vi "MotorSPS.vi"() -> ()   [LabVIEW 2010]
uses:
  StepMotor.lvclass
  Archive.lvclass
  <vilib>/Utility/miscctls.llb/LVScalePositionTypeDef.ctl
  <vilib>/Utility/xml.llb/Write to XML File(string).vi
  <vilib>/Utility/xml.llb/Read From XML File(string).vi
  Параметры СПШ.vi
  <vilib>/Utility/miscctls.llb/LVRowAndColumnTypeDef.ctl
panel:
  in  "Reload":bool
  out "Разрешение энкодера":dbl format="%#_10g"
  in  "Макс скорость двигателя":dbl caption="max скорость двигателя"
  in  "Редукция":dbl
  in  "Останов":bool
  out "Archive Data":refnum<class "Archive.lvclass">
  out "Archive Event":refnum<class "Archive.lvclass">
  out "Статус связи с СПШ":bool
  in  "Скорость передачи":i32(ring)=16 items=["75", "110", "134", "150", "300", "600", "1200", "1800", "2400", "4800", "7200", "9600", "14400", "19200", "38400", "57600", "115200", "128000"]
  in  "Имя порта":refnum<visa-resource-name>="COM6"
  out "Индикатор Статуса Конт":bool
  in  "Статус контроллера СПШ":T1(ring)
  out "StepMotor":refnum<class "StepMotor.lvclass">
  in  "Выход из программы":bool
  in  "Tab Control":T2(tab)
  out "Начальная позиция":dbl
  in  "Контроль концевиков":bool=TRUE
  out "Текущая позиция":dbl
  out "Условие энкодер":bool
  out "Инкремент импульсов":dbl
  in  "Контроль энкодера":bool
  out "Условие время":bool
  out "Лимит времени":dbl format="%<%M:%S>T"
  in  "Контроль времени":bool
  in  "Способ управления СПШ":T3(radio) caption="Способ управления двигателем"
  out "СкорРучРежРед":dbl caption="Скорость вала редуктора" format="%#_g об/мин"
  in  "Расчитать скорость":bool
  in  "Поворт экрана":dbl=180.0 min=0.0 max=360.0 step=1.0 format="%#_g °"
  in  "Время в мин":dbl=18.0 min=1.0 max=60.0 step=1.0 format="%2d мин"
  out "СкорРучРежМот":dbl caption="Скорость вала мотора" format="%#_g об/мин"
  in  "Напраление вращения":enum32{"Лево", "Право"}(radio)
  in  "Стоп Руч":bool
  in  "Пуск Руч":bool caption="Пуск ручной"
  out "ИсхСостСтарСтоп":bool
  in  "Двигатель в исходное сотояние":bool
  in  "Скорость двигателя":dbl caption="Скорость двигателя  об/мин" min=0.0 max=720.0 step=5.0
  out "Скорость редуктора":dbl caption="Скорость редуктора об/мин"
  in  "КонтрольКон":T4(radio)=enum."КонтрольПравКон" caption="Контроль концевика"
  out "РучнойСтартСтоп":bool
  out "Журнал событий":i32(listbox)
  in  "Количество циклов":i32
  out "ЦиклСтартСтоп":bool
  in  "Остоновить цикл":bool
  in  "Запустить цикл":bool
  in  "Шаги одного цикла":string[][](table)=[["7", "37"], ["4", "37"], ["4", "37"], ["9", "37"]]
  in  "Режим работы двигателя":T5(radio)=enum."Цикл реверсирования 180°"
  out "Прав.Конц":bool
  out "Лев.Конц":bool
  out "GaugeAngle":cluster{dbl, dbl}(knob) caption="Gauge" scale=0.0..360.0
  out "Значение энкодера":dbl caption="Лимит импульсов энкодера"
  out "Выбег":dbl
  out "Заданная позиция":dbl
  in  "SpeedSlide":dbl(slide) step=5.0 scale=0.0..720.0
  in  "Tree":string(tree)
  out "Waveform Chart":dynamicdata(graph)
  out "error":errorcluster
  in  "Период регистрации":string(combo)="1" caption="Период регистрации файла"
  in  "Номер банка программ":u16(ring) items=["0", "1", "2", "3", "4", "5", "6", "7"]
  in  "OK Button":bool
  # "Параметры установки"
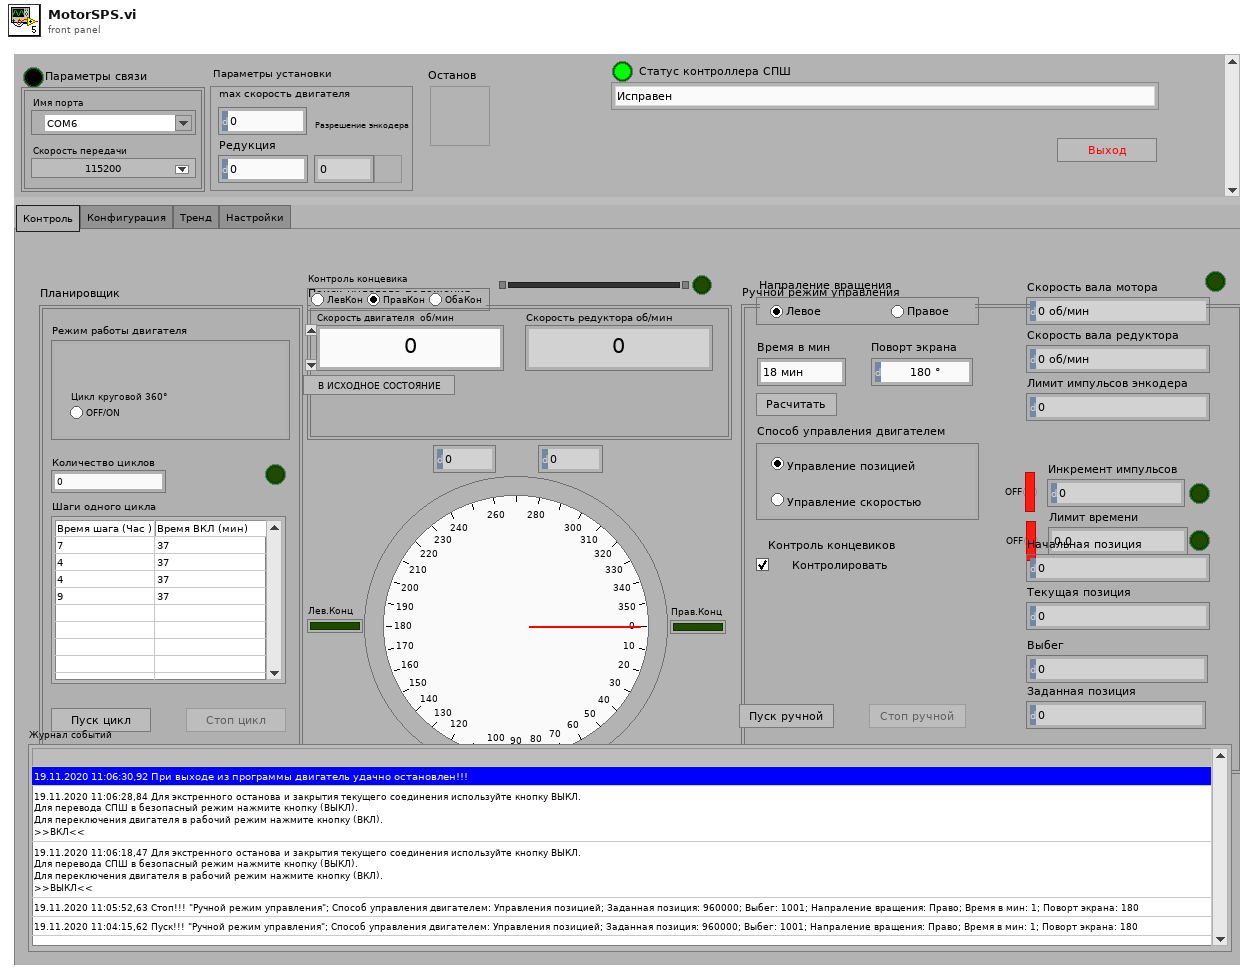
[diagram p1: front panel]
types:
  T1 = enum16{"Исправен", "Останов по команде", "Останов - высокое противодействующее усилие", "Останов - короткое замыкангие", "Выход из температурного диапазона", "Повышенное силовое напряжение", "Низкое силовое напряжение", "Повышанное цифровое напряжение", "Низкое цифровое напряжение", "Силовое напряжение превышает напряжение, установленое пользователем", "Останов - превышение допустимой перегрузки", "Останов - сработала защита IGBT модуля", "Останов - ощибка поиска фаз по UVW трекам", "Останов - ошибка в настройках энкодера", "Останов - сбой в работе энкодера", "Останов - ошибка фазировки двигателя"}
  T2 = enum32{"Контроль", "Конфигурация", "Тренд", "Настройки"}
  T3 = enum32{"Управления позицией", "Управления скоростью"}
  T4 = enum32{"КонтрольЛевКон", "КонтрольПравКон", "КонтрольОбаКон"}
  T5 = enum32{"Цикл круговой 360° ", "Цикл реверсирования 180°"}
  T6 = enum8{"Enabled", "Disabled", "Disabled and Grayed Out"}
  T7 = cluster{"Имя порта":refnum<visa-resource-name>, "Скорость передачи":i32, "Макс скорост двигатенля":dbl, "Редукция":dbl, "Разрешение энкодера":dbl, "Период регистрации":string}
  T8 = enum16{"open", "replace", "create", "open or create", "replace or create", "replace or create with confirmation"}
  T9 = enum16{"Порт ввода 1", "Порт ввода 2", "Порт ввода 3", "Порт ввода 4"}
  T10 = typedef "LVScalePositionTypeDef.ctl" = cluster{"Start":dbl, "Range":dbl}
  T11 = cluster{"Имя":string, "Группа":string, "Наименование":string, "Ед. изм":u16, "Список":string, "Адрес":u32, "Описание":string, "Мин":i32, "Макс":i32, "Сервис":bool, "Только чтение":bool, "Разработка":bool, "К-во бит":u16, "Шаг":u32, "Обработка":bool, "Макрос":string}[]
  T12 = cluster{"Двигатель в исходное сотояние":bool, "DisabledEnum":enum8{"Enabled", "Disabled", "Disabled and Grayed Out"}}
  T13 = cluster{"Стоп Руч":bool, "DisabledEnum":enum8{"Enabled", "Disabled", "Disabled and Grayed Out"}}
  T14 = cluster{"Пуск Руч":bool, "DisabledEnum":enum8{"Enabled", "Disabled", "Disabled and Grayed Out"}}
  T15 = cluster{"Скорость двигателя":dbl, "Maximum":dbl, "Minimum":dbl}
  T16 = cluster{"SpeedSlide":dbl, "Scale.Maximum":dbl, "Scale.Minimum":dbl}
  T17 = cluster{"GaugeAngle":cluster{dbl, dbl}, "Scale.Flipped":bool, "Scale.SclPos":T10}
  T18 = cluster{"РучнойСтартСтоп":bool, "Напраление вращения":enum32{"Лево", "Право"}, "Время в мин":dbl, "Поворт экрана":dbl, "СкорРучРежМот":dbl, "СкорРучРежРед":dbl, "Значение энкодера":dbl, "Расчитать скорость":bool, "Способ управления СПШ":enum32{"Управления позицией", "Управления скоростью"}, "Контроль энкодера":bool, "Инкремент импульсов":dbl, "Условие энкодер":bool, "Контроль времени":bool, "Лимит времени":dbl, "Условие время":bool, "Контроль концевиков":bool, "Начальная позиция":dbl, "Текущая позиция":dbl, "Выбег":dbl, "Заданная позиция":dbl, cluster{"Пуск Руч":bool, "DisabledEnum":enum8{"Enabled", "Disabled", "Disabled and Grayed Out"}}, cluster{"Стоп Руч":bool, "DisabledEnum":enum8{"Enabled", "Disabled", "Disabled and Grayed Out"}}}
  T19 = cluster{"ИсхСостСтарСтоп":bool, "КонтрольКон":enum32{"КонтрольЛевКон", "КонтрольПравКон", "КонтрольОбаКон"}, cluster{"SpeedSlide":dbl, "Scale.Maximum":dbl, "Scale.Minimum":dbl}, cluster{"Скорость двигателя":dbl, "Maximum":dbl, "Minimum":dbl}, "Скорость редуктора":dbl, cluster{"Двигатель в исходное сотояние":bool, "DisabledEnum":enum8{"Enabled", "Disabled", "Disabled and Grayed Out"}}}
  T20 = cluster{"Ручной режим управления":cluster{"РучнойСтартСтоп":bool, "Напраление вращения":enum32{"Лево", "Право"}, "Время в мин":dbl, "Поворт экрана":dbl, "СкорРучРежМот":dbl, "СкорРучРежРед":dbl, "Значение энкодера":dbl, "Расчитать скорость":bool, "Способ управления СПШ":enum32{"Управления позицией", "Управления скоростью"}, "Контроль энкодера":bool, "Инкремент импульсов":dbl, "Условие энкодер":bool, "Контроль времени":bool, "Лимит времени":dbl, "Условие время":bool, "Контроль концевиков":bool, "Начальная позиция":dbl, "Текущая позиция":dbl, "Выбег":dbl, "Заданная позиция":dbl, "ПускРуч":cluster{"Пуск Руч":bool, "DisabledEnum":enum8{"Enabled", "Disabled", "Disabled and Grayed Out"}}, "СтопРуч":cluster{"Стоп Руч":bool, "DisabledEnum":enum8{"Enabled", "Disabled", "Disabled and Grayed Out"}}}, "Поиск нулевого положения":cluster{"ИсхСостСтарСтоп":bool, "КонтрольКон":enum32{"КонтрольЛевКон", "КонтрольПравКон", "КонтрольОбаКон"}, "Слайдер скорости":cluster{"SpeedSlide":dbl, "Scale.Maximum":dbl, "Scale.Minimum":dbl}, "Индикатор скорости":cluster{"Скорость двигателя":dbl, "Maximum":dbl, "Minimum":dbl}, "Скорость редуктора":dbl, "Двигаться в исходное состояние":cluster{"ПускИсход":bool, "DisabledEnum":enum8{"Enabled", "Disabled", "Disabled and Grayed Out"}}}, "Прав.Конц":bool, "Лев.Конц":bool, "Стрелочный индикатор":cluster{"GaugeAngle":cluster{dbl, dbl}, "Scale.Flipped":bool, "Scale.SclPos":T10}, "Индикатор Статуса Конт":bool, "Статус контроллера СПШ":enum16{"Исправен", "Останов по команде", "Останов - высокое противодействующее усилие", "Останов - короткое замыкангие", "Выход из температурного диапазона", "Повышенное силовое напряжение", "Низкое силовое напряжение", "Повышанное цифровое напряжение", "Низкое цифровое напряжение", "Силовое напряжение превышает напряжение, установленое пользователем", "Останов - превышение допустимой перегрузки", "Останов - сработала защита IGBT модуля", "Останов - ощибка поиска фаз по UVW трекам", "Останов - ошибка в настройках энкодера", "Останов - сбой в работе энкодера", "Останов - ошибка фазировки двигателя"}, "Журнал событий":cluster{"Item Names":string[], "CellBG":u32}}
  T21 = typedef "LVRowAndColumnTypeDef.ctl" = cluster{"Row":i32, "Column":i32}
  T22 = typedef "LVDateTimeRec.ctl" = cluster{"fractional second":dbl, "second":i32, "minute":i32, "hour":i32, "day of month":i32, "month":i32, "year":i32, "day of week":i32, "day of year":i32, "DST":i32}
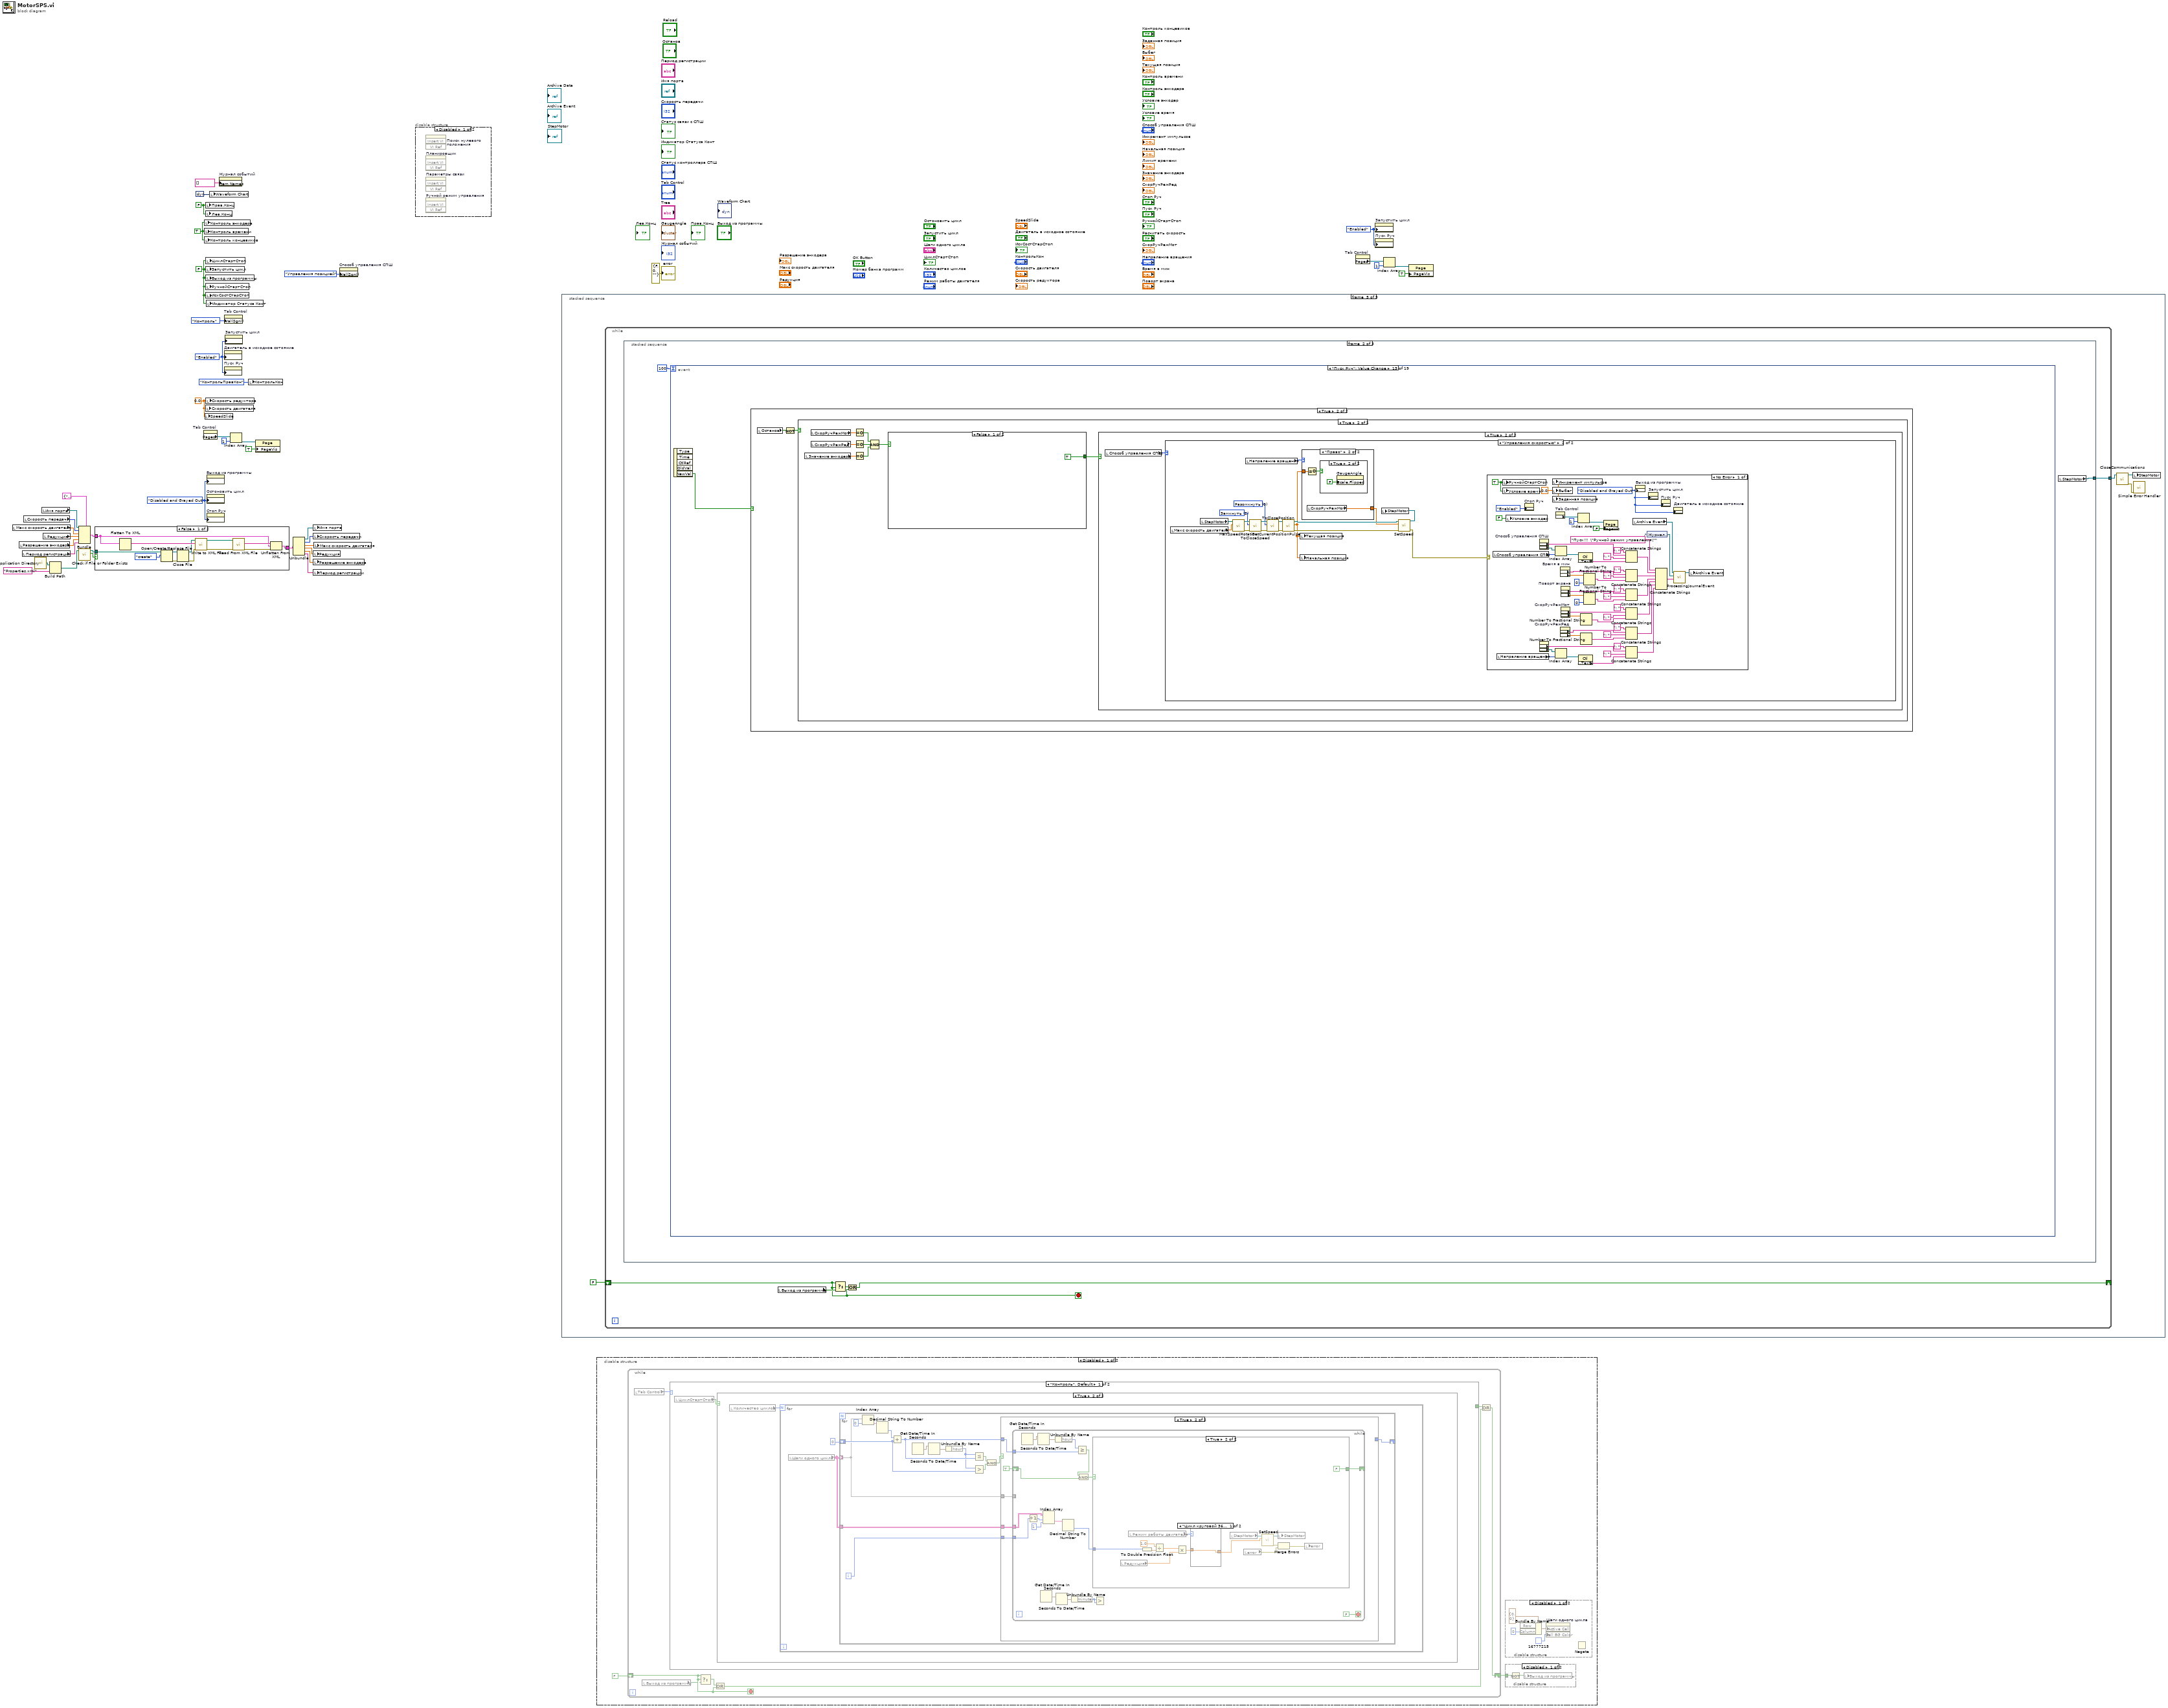
[diagram p0: block diagram]
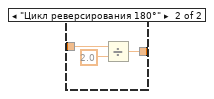
[diagram p7: hidden frame]
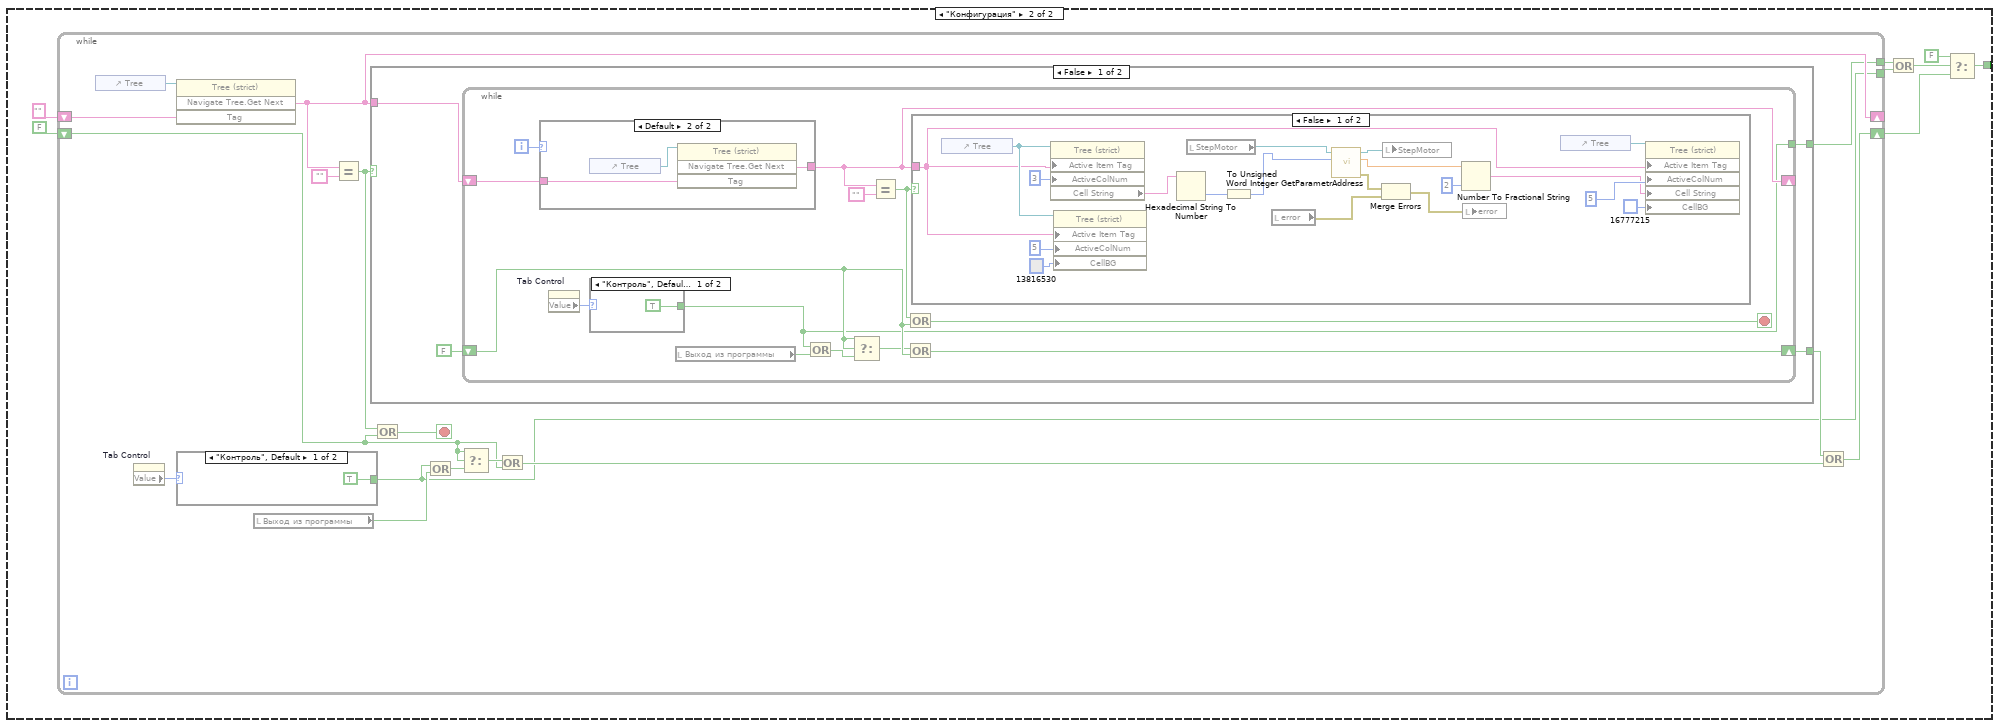
[diagram p8: hidden frame]
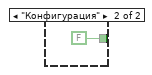
[diagram p9: hidden frame]
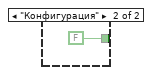
[diagram p10: hidden frame]
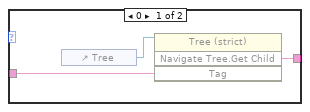
[diagram p12: hidden frame]
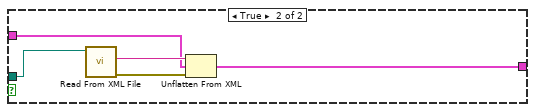
[diagram p15: hidden frame]
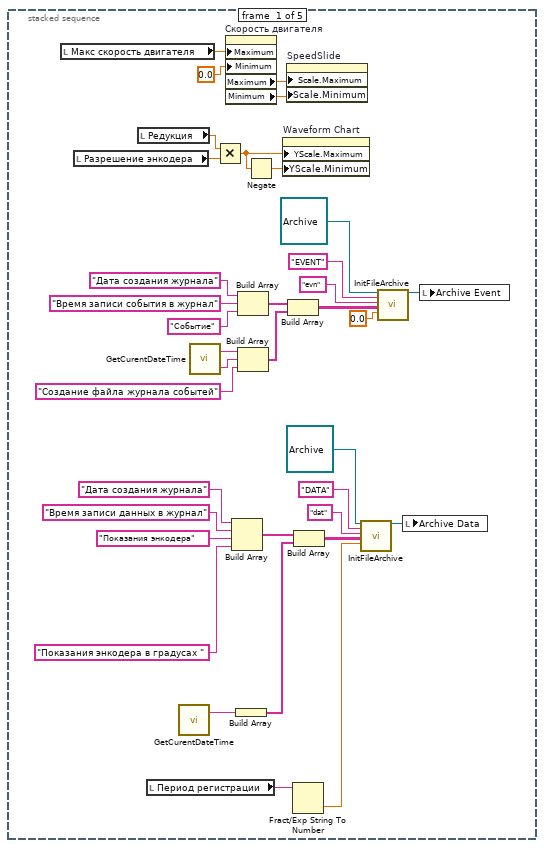
[diagram p17: hidden frame]
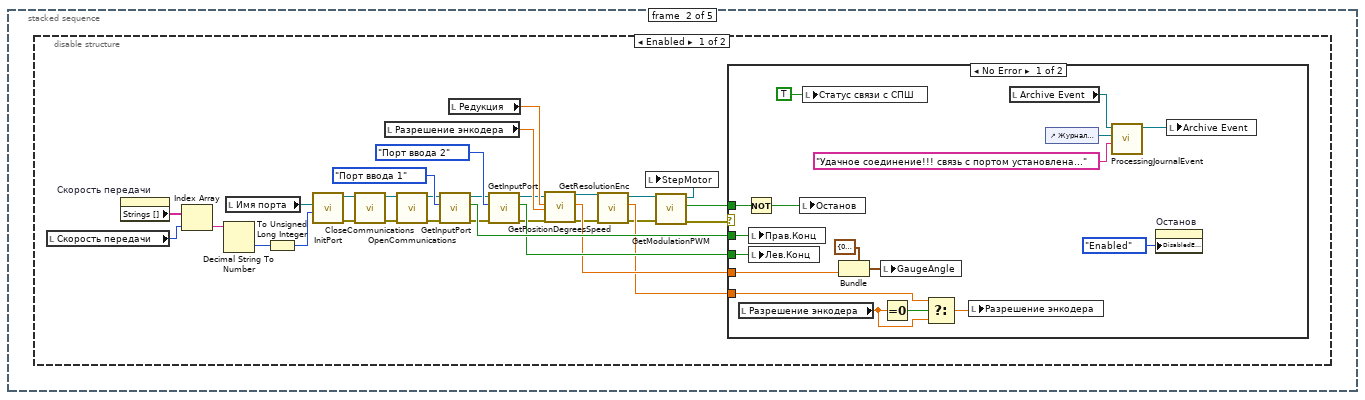
[diagram p18: hidden frame]
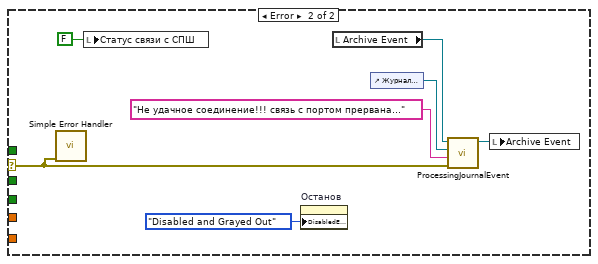
[diagram p19: hidden frame]
diagram:
  w3 = T6."Enabled" ("Disabled")
  w29 = TRUE ("Контроль времени")
  w31 = FALSE ("Прав.Конц")
  w30 = 0.0 ("Скорость об/мин")
  w33 = T6."Enabled" ("Disabled")
  w34 = T6."Disabled and Grayed Out" ("Disabled")
  w8 = FALSE ("Запустить цикл")
  n1 = local read "Макс скорость двигателя"() -> (w20:dbl)
  n2 = local read "Разрешение энкодера"() -> (w18:dbl)
  n3 = local read "Период регистрации"() -> (w17:string)
  n4 = local read "Скорость передачи"() -> (w21:i32)
  n5 = call <vilib>:"Application Directory.vi"() -> ("Application Directory"=w24:path)
  n6 = local read "Имя порта"() -> (w22:refnum<visa-resource-name>)
  n7 = local read "Редукция"() -> (w19:dbl)
  n8 = Build Path(base path=w24, name or relative path="Properties.xml" ("string")) -> (appended path=w27:path)
  n9 = Bundle(cluster=T7 {"Имя порта"="", "Скорость передачи"=0, "Макс скорост двигатенля"=0.0, "Редукция"=0.0, "Разрешение энкодера"=0.0, "Период регистрации"=""} ("Properties"), "Имя порта"=w22, "Скорость передачи"=w21, "Макс скорост двигатенля"=w20, "Редукция"=w19, "Разрешение энкодера"=w18, "Период регистрации"=w17) -> (w16:T7)
  n10 = call <vilib>:"Check if File or Folder Exists.vi"("path"=w27) -> ("file or folder exists?"=w25:bool, "dup path"=w23:path)  [unwired: 8 in, 1 out]
  n11 = case shown="False" w25 {
    tunnel: [w44 w57] -> w10
    tunnel: w23 -> [w43 w56]
    tunnel: w16 -> [w42 w55]
    frame False {
      n12 = Flatten To XML(anything=w42) -> (xml string=w53:string)
      n13 = Open/Create/Replace File(file path (use dialog)=w43, operation (0:open)=T8."create") -> (refnum out=w52:refnum<file>, error out=w51:errorcluster)  [unwired: 4 in, 1 out]
      n14 = Close File(refnum=w52, error in=w51) -> (path=w50:path, error out=w47:errorcluster)
      n15 = call-poly <vilib>:"Write to XML File.vi"("error in (no error)"=w47, "XML Input"=w53, "XML File Path"=w50) -> ("error out"=w48:errorcluster, "XML File Path(duplicate)"=w49:path)  [unwired: 6 in, 1 out]
      n16 = call-poly <vilib>:"Read From XML File.vi"("error in (no error)"=w48, "XML File Path"=w49) -> ("error out"=w45:errorcluster, "XML Elements"=w46:string)  [unwired: 7 in, 1 out]
      n17 = Unflatten From XML(xml string=w46, type=w42, error in (no error)=w45) -> (value=w44:T7)  [unwired: 1 out]
    }
    frame True {
      n18 = call-poly <vilib>:"Read From XML File.vi"("XML File Path"=w56) -> ("error out"=w58:errorcluster, "XML Elements"=w59:string)  [unwired: 8 in, 1 out]
      n19 = Unflatten From XML(xml string=w59, type=w55, error in (no error)=w58) -> (value=w57:T7)  [unwired: 1 out]
    }
  }
  n20 = property on="Tab Control" class="TabCtl (strict)"() -> ("Pages"=w36:refnum<vi>[])  [unwired: 2 in, 2 out]
  n21 = local write "Контроль энкодера"(w29) -> ()
  n22 = local write "Контроль времени"(w29) -> ()
  n23 = local write "Контроль концевиков"(w29) -> ()
  n24 = local write "SpeedSlide"(w30) -> ()
  n25 = local write "Прав.Конц"(w31) -> ()
  n26 = local write "Лев.Конц"(w31) -> ()
  n27 = local write "Скорость двигателя"(w30) -> ()
  n28 = local write "ЦиклСтартСтоп"(w8) -> ()
  n29 = local write "Запустить цикл"(w8) -> ()
  n30 = local write "Выход из программы"(w8) -> ()
  n31 = local write "РучнойСтартСтоп"(w8) -> ()
  n32 = local write "ИсхСостСтарСтоп"(w8) -> ()
  n33 = local write "Скорость редуктора"(w30) -> ()
  n34 = local write "Индикатор Статуса Конт"(w8) -> ()
  n35 = property on="Выход из программы" class="Bool (strict)"("DisabledEnum"=w34) -> ()  [unwired: 2 in, 2 out]
  n36 = property on="Остоновить цикл" class="Bool (strict)"("DisabledEnum"=w34) -> ()  [unwired: 2 in, 2 out]
  n37 = property on="Стоп Руч" class="Bool (strict)"("DisabledEnum"=w34) -> ()  [unwired: 2 in, 2 out]
  n38 = local write "Waveform Chart"(dynamicdata [] ("Waveform Chart")) -> ()
  n39 = property on="Журнал событий" class="LstBox (strict)"("Item Names"=string[] []) -> ()  [unwired: 2 in, 2 out]
  n40 = property on="Tab Control" class="TabCtl (strict)"("Val(Sgnl)"=enum32{"Контроль", "Конфигурация"}."Контроль" ("Value (Signaling)")) -> ()  [unwired: 2 in, 2 out]
  n41 = property on="Двигатель в исходное сотояние" class="Bool (strict)"("DisabledEnum"=w33) -> ()  [unwired: 2 in, 2 out]
  n42 = property on="Пуск Руч" class="Bool (strict)"("DisabledEnum"=w33) -> ()  [unwired: 2 in, 2 out]
  n43 = property on="Запустить цикл" class="Bool (strict)"("DisabledEnum"=w33) -> ()  [unwired: 2 in, 2 out]
  n44 = Index Array(array=w36, index=1) -> (element=w38:refnum<vi>)
  n45 = local write "КонтрольКон"(enum32{"КонтрольЛевКон", "КонтрольПравКон"}."КонтрольПравКон" ("КонтрольКон")) -> ()
  n46 = property class="Page"(reference=w38, "PageVis"=TRUE ("Page Visible")) -> ()  [unwired: 1 in, 2 out]
  n47 = Unbundle(w10) -> ("Имя порта"=w15:refnum<visa-resource-name>, "Скорость передачи"=w14:i32, "Макс скорост двигатенля"=w1:dbl, "Редукция"=w13:dbl, "Разрешение энкодера"=w12:dbl, "Период регистрации"=w9:string)
  n48 = local write "Имя порта"(w15) -> ()
  n49 = local write "Скорость передачи"(w14) -> ()
  n50 = local write "Редукция"(w13) -> ()
  n51 = local write "Разрешение энкодера"(w12) -> ()
  n52 = local write "Период регистрации"(w9) -> ()
  n53 = local write "Макс скорость двигателя"(w1) -> ()
  n54 = property on="Способ управления СПШ" class="RadioBtnsControl (strict)"("Val(Sgnl)"=T3."Управления позицией" ("Value (Signaling)")) -> ()  [unwired: 2 in, 2 out]
  n55 = disable-structure shown="Disabled" {
    frame Disabled {
      n56 = invoke on="Поиск нулевого положения" class="SubPanel" method="Insert VI"() -> ()  [unwired: 4 in, 4 out]
      n57 = invoke on="Планировщик" class="SubPanel" method="Insert VI"() -> ()  [unwired: 4 in, 4 out]
      n58 = invoke on="Параметры связи" class="SubPanel" method="Insert VI"() -> ()  [unwired: 4 in, 4 out]
      n59 = invoke on="Ручной режим управления" class="SubPanel" method="Insert VI"() -> ()  [unwired: 4 in, 4 out]
    }
    frame Enabled {
    }
  }
  n60 = stacked-sequence {
    frame #0 {
      n61 = local read "Макс скорость двигателя"() -> (w95:dbl)
      n62 = local read "Разрешение энкодера"() -> (w92:dbl)
      n63 = local read "Редукция"() -> (w91:dbl)
      n64 = local read "Период регистрации"() -> (w73:string)
      n65 = call "GetCurentDateTime.vi"() -> ("date"=w70:string)  [unwired: 2 in, 1 out]
      n66 = call "GetCurentDateTime.vi"() -> ("time"=w85:string, "date"=w84:string)  [unwired: 2 in]
      n67 = Multiply(x=w91, y=w92) -> (x*y=w93:dbl)
      n68 = property on="Скорость двигателя" class="DigNum (strict)"("Maximum"=w95, "Minimum"=0.0 ("Data Entry Limits:Minimum")) -> ("Maximum"=w89:dbl, "Minimum"=w90:dbl)  [unwired: 2 in, 2 out]
      n69 = Build Array("Дата создания журнала", "Время записи данных в журнал", "Показания энкодера" ("element"), "Показания энкодера в градусах " ("element")) -> (w62:string[])
      n70 = Build Array(w70) -> (w66:string[])
      n71 = Build Array("Дата создания журнала", "Время записи события в журнал", "Событие" ("element")) -> (w79:string[])
      n72 = Build Array(w84, w85, "Создание файла журнала событей" ("element")) -> (w75:string[])
      n73 = Negate(x=w93) -> (-x=w94:dbl)
      n74 = property on="Waveform Chart" class="WFChart (strict)"("YScale.Maximum"=w93, "YScale.Minimum"=w94) -> ()  [unwired: 2 in, 2 out]
      n75 = property on="SpeedSlide" class="Slide (strict)"("Scale.Maximum"=w89, "Scale.Minimum"=w90) -> ()  [unwired: 2 in, 2 out]
      n76 = Build Array(w79, w75) -> (w82:string[][])
      n77 = Fract/Exp String To Number(string=w73) -> (number=w72:dbl)  [unwired: 3 in, 1 out]
      n78 = Build Array(w62, w66) -> (w68:string[][])
      n79 = call-dynamic "InitFileArchive.vi"("Archive In"=refnum<class "Archive.lvclass"> refnum ("Archive.lvclass"), "Имя папки"="DATA", "Расширение имени файла"="dat", "Заголовок таблицы"=w68, "Период регистрации"=w72) -> ("Archive out"=w69:refnum<class "Archive.lvclass">)  [unwired: 13 in, 1 out]
      n80 = call-dynamic "InitFileArchive.vi"("Archive In"=refnum<class "Archive.lvclass"> refnum ("Archive.lvclass"), "Имя папки"="EVENT", "Расширение имени файла"="evn", "Заголовок таблицы"=w82, "Период регистрации"=0.0) -> ("Archive out"=w83:refnum<class "Archive.lvclass">)  [unwired: 13 in, 1 out]
      n81 = local write "Archive Data"(w69) -> ()
      n82 = local write "Archive Event"(w83) -> ()
    }
    frame #1 {
      n83 = disable-structure shown="Enabled" {
        frame Enabled {
          n84 = local read "Скорость передачи"() -> (w121:i32)
          n85 = property on="Скорость передачи" class="Ring (strict)"() -> ("Strings []"=w117:string[])  [unwired: 2 in, 2 out]
          n86 = Index Array(array=w117, index=w121) -> (element=w118:string)
          n87 = Decimal String To Number(string=w118) -> (number=w119:i32)  [unwired: 2 in, 1 out]
          n88 = local read "Имя порта"() -> (w122:refnum<visa-resource-name>)
          n89 = To Unsigned Long Integer(number=w119) -> (unsigned 32bit integer=w120:u32)
          n90 = call "InitPort.vi"("Скорость передачи"=w120, "Порт"=w122) -> ("error out"=w126:errorcluster, "StepMotor out"=w125:refnum<class "StepMotor.lvclass">)  [unwired: 8 in]
          n91 = call-dynamic "CloseCommunications .vi"("error in (no error)"=w126, "StepMotor in"=w125) -> ("error out"=w124:errorcluster, "StepMotor out"=w123:refnum<class "StepMotor.lvclass">)  [unwired: 8 in]
          n92 = local read "Разрешение энкодера"() -> (w108:dbl)
          n93 = call-dynamic "OpenCommunications .vi"("error in (no error)"=w124, "StepMotor in"=w123) -> ("error out"=w114:errorcluster, "StepMotor out"=w115:refnum<class "StepMotor.lvclass">)  [unwired: 8 in]
          n94 = call-dynamic "GetInputPort.vi"("error in (no error)"=w114, "PortInput"=T9."Порт ввода 1", "StepMotor in"=w115) -> ("error out"=w110:errorcluster, "Состояние"=w113:bool, "StepMotor out"=w111:refnum<class "StepMotor.lvclass">)  [unwired: 6 in]
          n95 = local read "Редукция"() -> (w107:dbl)
          n96 = call-dynamic "GetInputPort.vi"("error in (no error)"=w110, "PortInput"=T9."Порт ввода 2", "StepMotor in"=w111) -> ("error out"=w105:errorcluster, "Состояние"=w109:bool, "StepMotor out"=w106:refnum<class "StepMotor.lvclass">)  [unwired: 6 in]
          n97 = call "GetPositionDegreesSpeed.vi"("StepMotor in"=w106, "Редукция"=w107, "Разрешение энкодера"=w108, "error in (no error)"=w105) -> ("StepMotor out"=w103:refnum<class "StepMotor.lvclass">, "Значение"=w104:dbl, "error out"=w102:errorcluster)  [unwired: 11 in, 2 out]
          n98 = call-dynamic "GetResolutionEnc.vi"("error in (no error)"=w102, "StepMotor in"=w103) -> ("error out"=w99:errorcluster, "Разрешение энкодера"=w101:dbl, "StepMotor out"=w100:refnum<class "StepMotor.lvclass">)  [unwired: 7 in]
          n99 = call-dynamic "GetModulationPWM.vi"("error in (no error)"=w99, "StepMotor in"=w100) -> ("error out"=w96:errorcluster, "Значение"=w98:bool, "StepMotor out"=w97:refnum<class "StepMotor.lvclass">)  [unwired: 7 in]
          n100 = local write "StepMotor"(w97) -> ()
          n101 = case shown="No Error" w96 {
            selector: w96 -> [_ w145]
            tunnel: w113 -> [w138 _]
            tunnel: w109 -> [w137 _]
            tunnel: w104 -> [w135 _]
            tunnel: w101 -> [w129 _]
            tunnel: w98 -> [w134 _]
            frame No Error {
              n102 = local read "Разрешение энкодера"() -> (w127:dbl)
              n103 = Not(x=w134) -> (.not. x?=w133:bool)
              n104 = local write "Прав.Конц"(w138) -> ()
              n105 = local write "Лев.Конц"(w137) -> ()
              n106 = local write "Останов"(w133) -> ()
              n107 = local write "Статус связи с СПШ"(TRUE ("Статус связи с СПШ")) -> ()
              n108 = Bundle(cluster=cluster{dbl, dbl} {0.0, 0.0} ("GaugeAngle"), w135) -> (w136:cluster{dbl, dbl})  [unwired: 1 in]
              n109 = local write "GaugeAngle"(w136) -> ()
              n110 = Equal To 0?(x=w127) -> (x = 0?=w130:bool)
              n111 = Select(t=w129, s=w130, f=w127) -> (s? t:f=w128:dbl)
              n112 = local write "Разрешение энкодера"(w128) -> ()
              n113 = local read "Archive Event"() -> (w140:refnum<class "Archive.lvclass">)
              n114 = control-ref of="Журнал событий"() -> (w141:refnum<vi>)
              n115 = call "ProcessingJournalEvent.vi"("Новая строка в журнале"="Удачное соединение!!! связь с портом установлена...", "Журнал событий"=w141, "ArchiveInput"=w140) -> ("Archive Out"=w139:refnum<class "Archive.lvclass">)  [unwired: 8 in]
              n116 = property on="Останов" class="Bool (strict)"("DisabledEnum"=T6."Enabled" ("Disabled")) -> ()  [unwired: 2 in, 2 out]
              n117 = local write "Archive Event"(w139) -> ()
            }
            frame Error {
              n118 = call <vilib>:"Simple Error Handler.vi"("error in (no error)"=w145) -> ()  [unwired: 1 in, 8 out]
              n119 = local write "Статус связи с СПШ"(FALSE ("Статус связи с СПШ")) -> ()
              n120 = property on="Останов" class="Bool (strict)"("DisabledEnum"=T6."Disabled and Grayed Out" ("Disabled")) -> ()  [unwired: 2 in, 2 out]
              n121 = local read "Archive Event"() -> (w147:refnum<class "Archive.lvclass">)
              n122 = control-ref of="Журнал событий"() -> (w148:refnum<vi>)
              n123 = call "ProcessingJournalEvent.vi"("error IO"=w145, "Новая строка в журнале"="Не удачное соединение!!! связь с портом прервана…", "Журнал событий"=w148, "ArchiveInput"=w147) -> ("Archive Out"=w146:refnum<class "Archive.lvclass">)  [unwired: 7 in]
              n124 = local write "Archive Event"(w146) -> ()
            }
          }
        }
        frame Disabled {
        }
      }
    }
    frame #2 {
      n125 = disable-structure shown="Enabled" {
        frame Enabled {
          w152 = FALSE ("Visible Items:Symbols Visible")
          n126 = control-ref of="Tree"() -> (w166:refnum<vi>)
          n127 = invoke class="Tree (strict)" method="Edit Tree Items.Delete"(reference=w166, "Delete Children"=TRUE ("Delete Children?")) -> (reference out=w158:refnum<vi>, error out=w157:errorcluster)  [unwired: 3 in, 3 out]
          n128 = property class="VI"() -> (error out=w161:errorcluster, "Panel"=w163:refnum<vi>)  [unwired: 2 in, 1 out]
          n129 = property class="Tree (strict)"(reference=w158, error in=w157, "ColHdrString"=string[] ["Группа", "Наименование", "Единица", "Адрес", "Количество бит", "Значение", "Чтение\\Запись"] ("Child Text")) -> (reference out=w156:refnum<vi>, error out=w155:errorcluster)
          n130 = global read "Параметры СПШ.vi" "Параметры СПШ"() -> (w165:T11)
          n131 = property class="Pnl"(reference=w163, error in=w161, "DeferPanUpdts"=TRUE ("Defer Panel Updates")) -> ()  [unwired: 2 out]
          n132 = for {
            tunnel: w165 -> [w179] mode=indexing
            shift-right: [w175] -> w160
            shift-left: w156 -> [w176]
            shift-right: [w174] -> w151
            shift-left: w155 -> [w177]
            n133 = Unbundle By Name(w179) -> ("Группа"=w178:string)
            n134 = while {
              shift-right: [w221] -> w167
              shift-left: "" ("Tag") -> [w222]
              shift-right: [w218] -> w171
              shift-left: TRUE -> [w217]
              tunnel: w177 -> [w216]
              tunnel: [w215] -> w169
              tunnel: w176 -> [w214]
              tunnel: [w213] -> w168
              shift-right: [w219] -> w172
              shift-left: w178 -> [w223]
              stop <- w220 stop-if-true
              n135 = invoke class="Tree (strict)" method="Navigate Tree.Get Next"(reference=w214, error in=w216, "Tag"=w222) -> (reference out=w213:refnum<vi>, error out=w215:errorcluster, "Navigate Tree:Get Next Item"=w221:string)  [unwired: 1 in, 1 out]
              n136 = Equal?(x=w221, y="") -> (x = y?=w220:bool)
              n137 = case shown="True" w220 {
                tunnel: w221 -> [w228 _]
                tunnel: w223 -> [w229 w235]
                tunnel: [w227 w235] -> w219
                tunnel: [w226 w236] -> w218
                tunnel: w217 -> [w225 w236]
                frame False {
                  n138 = Equal?(x=w228, y=w229) -> (x = y?=w230:bool)
                  n139 = case shown="True" w230 {
                    tunnel: w229 -> [w231 w234]
                    tunnel: [w231 w234] -> w227
                    tunnel: [w232 FALSE] -> w226
                    tunnel: w225 -> [w232 _]
                    frame False {
                    }
                    frame True {
                    }
                  }
                }
                frame True {
                }
              }
            }
            n140 = case shown="True" w171 {
              tunnel: w172 -> [_ w184]
              tunnel: w169 -> [w180 w188]
              tunnel: w168 -> [w181 w187]
              tunnel: [w181 w186] -> w175
              tunnel: [w180 w185] -> w174
              tunnel: w167 -> [_ w183]
              frame False {
              }
              frame True {
                n141 = for {
                  tunnel: w188 -> [w198]
                  tunnel: w187 -> [w197]
                  tunnel: [w196] -> w186
                  tunnel: [w195] -> w185
                  tunnel: w184 -> [w191]
                  tunnel: w183 -> [w194]
                  tunnel: string[][] [["cp", "Контур тока"], ["vp", "Контур скорости"], ["pp", "Контур положения"], ["st", "Общие"], ["ip", "Интерфейс"], ["ep", "Сервисные параметры"], ["io", "Порты ввода-вывода"], ["pd", "Технологический ПИД регулятор"], ["ct", "Параметры управления"], ["dd", "Динамические парамтры"], ["ss", "Системные парамтры"], ["tp", "Параметры тестирования"], ["up", "Пользовательские парметры"]] ("Child Text") -> [w190] mode=indexing
                  n142 = Index Array(array=w190, index=0) -> (element=w192:string)
                  n143 = Equal?(x=w191, y=w192) -> (x = y?=w189:bool)
                  n144 = case shown="True" w189 {
                    tunnel: w198 -> [w199 w212]
                    tunnel: w197 -> [w200 w211]
                    tunnel: [w200 w210] -> w196
                    tunnel: [w199 w209] -> w195
                    tunnel: w194 -> [_ w208]
                    tunnel: w191 -> [_ w201]
                    tunnel: w190 -> [_ w206]
                    frame False {
                    }
                    frame True {
                      n145 = Index Array(array=w206, index=1) -> (element=w203:string)
                      n146 = Concatenate Strings(w201, ": " ("string"), w203) -> (w204:string)
                      n147 = invoke class="Tree (strict)" method="Edit Tree Items.Add Item"(reference=w211, error in=w212, "Parent Tag"=w208, "Child Position"=-1, "Left Cell"=w204, "Child Tag"=w201) -> (reference out=w210:refnum<vi>, error out=w209:errorcluster)  [unwired: 3 in, 7 out]
                    }
                  }
                }
              }
            }
          }
          n148 = property class="Tree (strict)"(reference=w160, error in=w151, "Visible Items:Symbols Visible"=w152) -> (reference out=w154:refnum<vi>)  [unwired: 1 out]
          n149 = invoke class="Tree (strict)" method="Open/Close.Open/Close All"(reference=w154, "Open"=w152) -> (error out=w153:errorcluster)  [unwired: 2 in, 3 out]
          n150 = call <vilib>:"Simple Error Handler.vi"("error in (no error)"=w153) -> ()  [unwired: 4 in, 5 out]
        }
        frame Disabled {
        }
      }
    }
    frame #3 {
      n151 = disable-structure shown="Enabled" {
        frame Enabled {
          n152 = while {
            shift-right: [w247] -> _
            shift-left: "" ("Tag") -> [w249]
            tunnel: [T6."Enabled" ("Disabled")] -> w239
            tunnel: [w241] -> w237
            stop <- w243 stop-if-true
            n153 = control-ref of="Tree"() -> (w250:refnum<vi>)
            n154 = invoke class="Tree (strict)" method="Navigate Tree.Get Next"(reference=w250, "Tag"=w249) -> (error out=w246:errorcluster, "Navigate Tree:Get Next Item"=w245:string)  [unwired: 2 in, 2 out]
            n155 = global read "Параметры СПШ.vi" "Параметры СПШ"() -> (w248:T11)
            n156 = for {
              tunnel: w248 -> [w254] mode=indexing
              tunnel: w245 -> [w253]
              tunnel: [w253] -> w247
              tunnel: w246 -> [_]
              n157 = Unbundle By Name(w254) -> ("Группа"=w252:string)
              n158 = Equal?(x=w253, y=w252) -> (x = y?=w251:bool)
              n159 = case shown="True" w251 {
                tunnel: w254 -> [_ w279]
                tunnel: w253 -> [_ w274]
                frame False {
                }
                frame True {
                  n160 = Unbundle By Name(w279) -> ("Имя"=w257:string, "Наименование"=w278:string, "Ед. изм"=w277:u16, "Адрес"=w275:u32, "К-во бит"=w276:u16, "Только чтение"=w256:bool)
                  n161 = To Long Integer(number=w277) -> (32bit integer=w272:i32)
                  n162 = To Unsigned Word Integer(number=w275) -> (unsigned 16bit integer=w260:u16)
                  n163 = Quotient & Remainder(x=w276, y=u16 8) -> (floor(x/y)=w270:u16)  [unwired: 1 out]
                  n164 = Select(t="Read", s=w256, f="Write\\Read") -> (s? t:f=w265:string)
                  n165 = Index Array(array=string[] ["", "дискрет", "об/(сек^2)", "сек", "об/мин", "А", "имп.", "град.", "В", "мксек", "Банк", "мсек", "кГц", "А2сек", "nсек"] ("Strings []"), index=w272) -> (element=w269:string)
                  n166 = Number To Decimal String(number=w270) -> (decimal integer string=w255:string)  [unwired: 1 in]
                  n167 = Number To Hexadecimal String(1:i16 4 ("width (-)"), 2:w260) -> (0:w258:string)
                  n168 = control-ref of="Tree"() -> (w261:refnum<vi>)
                  n169 = Build Array(w278, w269, w258, w255, "0" ("element"), w265) -> (w273:string[])
                  n170 = invoke class="Tree (strict)" method="Edit Tree Items.Add Item"(reference=w261, "Parent Tag"=w274, "Child Position"=-1, "Left Cell"=w257, "Child Text"=w273, "Child Only?"=TRUE) -> ()  [unwired: 3 in, 9 out]
                }
              }
            }
            n171 = Equal?(x=w245, y="") -> (x = y?=w243:bool)
            n172 = property class="VI"() -> ("Panel"=w241:refnum<vi>)  [unwired: 2 in, 2 out]
          }
          n173 = property on="Выход из программы" class="Bool (strict)"("DisabledEnum"=w239) -> ()  [unwired: 2 in, 2 out]
          n174 = property class="Pnl"(reference=w237, "DeferPanUpdts"=FALSE ("Defer Panel Updates")) -> ()  [unwired: 1 in, 2 out]
        }
        frame Disabled {
        }
      }
    }
    frame #4 {
      n175 = while {
        shift-right: [w285] -> _
        shift-left: FALSE ("Выход из программы") -> [w284]
        tunnel: [w286] -> w281
        stop <- w284 stop-if-true
        n176 = stacked-sequence {
          tunnel: [_ w345 _] -> w286
          frame #0 {
            n177 = local read "Двигатель в исходное сотояние"() -> (w292:bool)
            n178 = local read "Статус контроллера СПШ"() -> (w301:T1)
            n179 = local read "Индикатор Статуса Конт"() -> (w302:bool)
            n180 = local read "Способ управления СПШ"() -> (w335:T3)
            n181 = local read "Напраление вращения"() -> (w342:enum32{"Лево", "Право"})
            n182 = local read "Контроль концевиков"() -> (w328:bool)
            n183 = local read "Инкремент импульсов"() -> (w333:dbl)
            n184 = local read "Скорость редуктора"() -> (w313:dbl)
            n185 = local read "Скорость двигателя"() -> (w320:dbl)
            n186 = local read "Расчитать скорость"() -> (w336:bool)
            n187 = local read "Контроль энкодера"() -> (w334:bool)
            n188 = local read "Значение энкодера"() -> (w337:dbl)
            n189 = local read "Начальная позиция"() -> (w327:dbl)
            n190 = local read "Контроль времени"() -> (w331:bool)
            n191 = local read "Заданная позиция"() -> (w324:dbl)
            n192 = local read "РучнойСтартСтоп"() -> (w343:bool)
            n193 = local read "ИсхСостСтарСтоп"() -> (w317:bool)
            n194 = local read "Текущая позиция"() -> (w326:dbl)
            n195 = local read "Условие энкодер"() -> (w332:bool)
            n196 = local read "СкорРучРежМот"() -> (w339:dbl)
            n197 = local read "СкорРучРежРед"() -> (w338:dbl)
            n198 = local read "Лимит времени"() -> (w330:dbl)
            n199 = local read "Поворт экрана"() -> (w340:dbl)
            n200 = local read "Условие время"() -> (w329:bool)
            n201 = local read "КонтрольКон"() -> (w316:T4)
            n202 = local read "Время в мин"() -> (w341:dbl)
            n203 = property on="SpeedSlide" class="Slide (strict)"() -> ("Scale.Maximum"=w322:dbl, "Scale.Minimum"=w321:dbl)  [unwired: 2 in, 2 out]
            n204 = local read "GaugeAngle"() -> (w312:cluster{dbl, dbl})
            n205 = local read "Прав.Конц"() -> (w305:bool)
            n206 = local read "SpeedSlide"() -> (w323:dbl)
            n207 = local read "Лев.Конц"() -> (w304:bool)
            n208 = property on="GaugeAngle" class="Knob (strict)"() -> ("Scale.Flipped"=w311:bool)  [unwired: 2 in, 2 out]
            n209 = local read "Стоп Руч"() -> (w299:bool)
            n210 = local read "Пуск Руч"() -> (w296:bool)
            n211 = property on="GaugeAngle" class="Knob (strict)"() -> ("Scale.SclPos"=w310:T10)  [unwired: 2 in, 2 out]
            n212 = property on="Журнал событий" class="LstBox (strict)"() -> ("Item Names"=w307:string[])  [unwired: 2 in, 2 out]
            n213 = local read "Выбег"() -> (w325:dbl)
            n214 = property on="Скорость двигателя" class="DigNum (strict)"() -> ("Maximum"=w319:dbl, "Minimum"=w318:dbl)  [unwired: 2 in, 2 out]
            n215 = property on="Пуск Руч" class="Bool (strict)"() -> ("DisabledEnum"=w297:T6)  [unwired: 2 in, 2 out]
            n216 = property on="Стоп Руч" class="Bool (strict)"() -> ("DisabledEnum"=w298:T6)  [unwired: 2 in, 2 out]
            n217 = property on="Двигатель в исходное сотояние" class="Bool (strict)"() -> ("DisabledEnum"=w293:T6)  [unwired: 2 in, 2 out]
            n218 = property on="Журнал событий" class="LstBox (strict)"() -> ("CellBG"=w306:u32)  [unwired: 2 in, 2 out]
            n219 = Bundle("Двигатель в исходное сотояние"=w292, "DisabledEnum"=w293) -> (w291:T12)  [unwired: 1 in]
            n220 = Bundle("Стоп Руч"=w299, "DisabledEnum"=w298) -> (w294:T13)  [unwired: 1 in]
            n221 = Bundle("Пуск Руч"=w296, "DisabledEnum"=w297) -> (w295:T14)  [unwired: 1 in]
            n222 = Bundle("Скорость двигателя"=w320, "Maximum"=w319, "Minimum"=w318) -> (w314:T15)  [unwired: 1 in]
            n223 = Bundle("SpeedSlide"=w323, "Scale.Maximum"=w322, "Scale.Minimum"=w321) -> (w315:T16)  [unwired: 1 in]
            n224 = Bundle("GaugeAngle"=w312, "Scale.Flipped"=w311, "Scale.SclPos"=w310) -> (w303:T17)  [unwired: 1 in]
            n225 = Bundle("Item Names"=w307, "CellBG"=w306) -> (w300:cluster{"Item Names":string[], "CellBG":u32})  [unwired: 1 in]
            n226 = Bundle("РучнойСтартСтоп"=w343, "Напраление вращения"=w342, "Время в мин"=w341, "Поворт экрана"=w340, "СкорРучРежМот"=w339, "СкорРучРежРед"=w338, "Значение энкодера"=w337, "Расчитать скорость"=w336, "Способ управления СПШ"=w335, "Контроль энкодера"=w334, "Инкремент импульсов"=w333, "Условие энкодер"=w332, "Контроль времени"=w331, "Лимит времени"=w330, "Условие время"=w329, "Контроль концевиков"=w328, "Начальная позиция"=w327, "Текущая позиция"=w326, "Выбег"=w325, "Заданная позиция"=w324, w295, w294) -> (w309:T18)  [unwired: 1 in]
            n227 = Bundle("ИсхСостСтарСтоп"=w317, "КонтрольКон"=w316, w315, w314, "Скорость редуктора"=w313, w291) -> (w308:T19)  [unwired: 1 in]
            n228 = shared-variable "My Computer\\Library MotorSPS.lvlib\\MotorSPS Variable"() -> (w289:T20)  [unwired: 1 in, 1 out]
            n229 = Bundle(cluster=w289, "Ручной режим управления"=w309, "Поиск нулевого положения"=w308, "Прав.Конц"=w305, "Лев.Конц"=w304, "Стрелочный индикатор"=w303, "Индикатор Статуса Конт"=w302, "Статус контроллера СПШ"=w301, "Журнал событий"=w300) -> (w290:T20)
            n230 = shared-variable "My Computer\\Library MotorSPS.lvlib\\MotorSPS Variable"(w290) -> ()  [unwired: 1 in, 1 out]
          }
          frame #1 {
            n231 = event shown="[12] \"Пуск Руч\": Value Change" {
              selector: _ -> [_ _ _ _ _ _ _ _ _ _ _ _ _ _ _ _ _ _ _]
              dyn-events: _ -> [_ _ _ _ _ _ _ _ _ _ _ _ _ _ _ _ _ _ _]
              timeout: 100 -> [_ _ _ _ _ _ _ _ _ _ _ _ _ _ _ _ _ _ _]
              event Timeout {
                n232 = event-data() -> ()  [unwired: 1 in, 3 out]
                n233 = local read "Статус связи с СПШ"() -> (w346:bool)
                n234 = case shown="True" w346 {
                  frame False {
                  }
                  frame True {
                    n235 = local read "ИсхСостСтарСтоп"() -> (w348:bool)
                    n236 = local read "РучнойСтартСтоп"() -> (w347:bool)
                    n237 = case shown="True" w348 {
                      frame False {
                      }
                      frame True {
                        n238 = local read "КонтрольКон"() -> (w704:T4)
                        n239 = case shown="\"КонтрольОбаКон\"" w704 {
                          tunnel: [w705 w713 w733] -> w703
                          frame "КонтрольЛевКон", Default {
                            n240 = local read "StepMotor"() -> (w707:refnum<class "StepMotor.lvclass">)
                            n241 = call-dynamic "GetInputPort.vi"("PortInput"=T9."Порт ввода 2", "StepMotor in"=w707) -> ("error out"=w709:errorcluster, "Состояние"=w710:bool, "StepMotor out"=w706:refnum<class "StepMotor.lvclass">)  [unwired: 7 in]
                            n242 = local write "StepMotor"(w706) -> ()
                            n243 = case shown="No Error" w709 {
                              tunnel: w710 -> [w711 _]
                              tunnel: [w711 w712] -> w705
                              frame No Error {
                                n244 = local write "Лев.Конц"(w711) -> ()
                              }
                              frame Error {
                                n245 = local read "Лев.Конц"() -> (w712:bool)
                              }
                            }
                          }
                          frame "КонтрольПравКон" {
                            n246 = local read "StepMotor"() -> (w715:refnum<class "StepMotor.lvclass">)
                            n247 = call-dynamic "GetInputPort.vi"("PortInput"=T9."Порт ввода 1", "StepMotor in"=w715) -> ("error out"=w717:errorcluster, "Состояние"=w718:bool, "StepMotor out"=w714:refnum<class "StepMotor.lvclass">)  [unwired: 7 in]
                            n248 = local write "StepMotor"(w714) -> ()
                            n249 = case shown="No Error" w717 {
                              tunnel: w718 -> [w719 _]
                              tunnel: [w719 w720] -> w713
                              frame No Error {
                                n250 = local write "Прав.Конц"(w719) -> ()
                              }
                              frame Error {
                                n251 = local read "Прав.Конц"() -> (w720:bool)
                              }
                            }
                          }
                          frame "КонтрольОбаКон" {
                            n252 = local read "StepMotor"() -> (w729:refnum<class "StepMotor.lvclass">)
                            n253 = local read "StepMotor"() -> (w724:refnum<class "StepMotor.lvclass">)
                            n254 = call-dynamic "GetInputPort.vi"("PortInput"=T9."Порт ввода 2", "StepMotor in"=w729) -> ("error out"=w727:errorcluster, "Состояние"=w731:bool, "StepMotor out"=w730:refnum<class "StepMotor.lvclass">)  [unwired: 7 in]
                            n255 = local write "StepMotor"(w730) -> ()
                            n256 = call-dynamic "GetInputPort.vi"("PortInput"=T9."Порт ввода 1", "StepMotor in"=w724) -> ("error out"=w726:errorcluster, "Состояние"=w732:bool, "StepMotor out"=w723:refnum<class "StepMotor.lvclass">)  [unwired: 7 in]
                            n257 = local write "StepMotor"(w723) -> ()
                            n258 = case shown="Error" w726 {
                              tunnel: w732 -> [w736 _]
                              tunnel: [w736 w737] -> w721
                              frame No Error {
                                n259 = local write "Прав.Конц"(w736) -> ()
                              }
                              frame Error {
                                n260 = local read "Прав.Конц"() -> (w737:bool)
                              }
                            }
                            n261 = case shown="Error" w727 {
                              tunnel: w731 -> [w734 _]
                              tunnel: [w734 w735] -> w722
                              frame No Error {
                                n262 = local write "Лев.Конц"(w734) -> ()
                              }
                              frame Error {
                                n263 = local read "Лев.Конц"() -> (w735:bool)
                              }
                            }
                            n264 = Or(x=w722, y=w721) -> (x .or. y?=w733:bool)
                          }
                        }
                        n265 = case shown="False" w703 {
                          frame False {
                            n266 = local read "Разрешение энкодера"() -> (w739:dbl)
                            n267 = local read "StepMotor"() -> (w746:refnum<class "StepMotor.lvclass">)
                            n268 = local read "StepMotor"() -> (w744:refnum<class "StepMotor.lvclass">)
                            n269 = local read "Редукция"() -> (w743:dbl)
                            n270 = call-dynamic "GetSpeed.vi"("StepMotor in"=w746) -> ("error out"=w745:errorcluster, "Скорость"=w748:dbl, "StepMotor out"=w747:refnum<class "StepMotor.lvclass">)  [unwired: 8 in]
                            n271 = local write "StepMotor"(w747) -> ()
                            n272 = call "GetPositionDegreesSpeed.vi"("StepMotor in"=w744, "Редукция"=w743, "Разрешение энкодера"=w739) -> ("StepMotor out"=w741:refnum<class "StepMotor.lvclass">, "Значение"=w740:dbl, "+ 0 -"=w738:bool, "error out"=w742:errorcluster)  [unwired: 12 in, 1 out]
                            n273 = local write "StepMotor"(w741) -> ()
                            n274 = case shown="No Error" w745 {
                              selector: w745 -> [_ w752]
                              tunnel: w748 -> [w750 _]
                              frame No Error {
                                n275 = local read "Редукция"() -> (w749:dbl)
                                n276 = Divide(x=w750, y=w749) -> (x/y=w751:dbl)
                                n277 = local write "Скорость редуктора"(w751) -> ()
                              }
                              frame Error {
                                n278 = local read "Archive Event"() -> (w753:refnum<class "Archive.lvclass">)
                                n279 = control-ref of="Журнал событий"() -> (w755:refnum<vi>)
                                n280 = call "ProcessingJournalEvent.vi"("error IO"=w752, "Журнал событий"=w755, "ArchiveInput"=w753) -> ("Archive Out"=w754:refnum<class "Archive.lvclass">)  [unwired: 8 in]
                                n281 = local write "Archive Event"(w754) -> ()
                              }
                            }
                            n282 = case shown="No Error" w742 {
                              selector: w742 -> [_ w767]
                              tunnel: w740 -> [w759 _]
                              tunnel: w738 -> [w758 _]
                              frame No Error {
                                n283 = case shown="True" w758 {
                                frame False {
                                }
                                frame True {
                                n284 = local read "КонтрольКон"() -> (w760:T4)
                                n285 = case shown="\"КонтрольОбаКон\"" w760 {
                                frame "КонтрольЛевКон", Default {
                                n286 = property on="GaugeAngle" class="Knob (strict)"("Scale.Flipped"=TRUE) -> ()  [unwired: 2 in, 2 out]
                                }
                                frame "КонтрольПравКон" {
                                n287 = property on="GaugeAngle" class="Knob (strict)"("Scale.Flipped"=FALSE) -> ()  [unwired: 2 in, 2 out]
                                }
                                frame "КонтрольОбаКон" {
                                n288 = local read "Скорость двигателя"() -> (w764:dbl)
                                n289 = Less Than 0?(x=w764) -> (x < 0?=w763:bool)
                                n290 = case shown="False" w763 {
                                frame False {
                                n291 = property on="GaugeAngle" class="Knob (strict)"("Scale.Flipped"=FALSE) -> ()  [unwired: 2 in, 2 out]
                                }
                                frame True {
                                n292 = property on="GaugeAngle" class="Knob (strict)"("Scale.Flipped"=TRUE) -> ()  [unwired: 2 in, 2 out]
                                }
                                }
                                }
                                }
                                }
                                }
                                n293 = Bundle(cluster=cluster{dbl, dbl} {0.0, 0.0} ("GaugeAngle"), w759) -> (w756:cluster{dbl, dbl})  [unwired: 1 in]
                                n294 = local write "GaugeAngle"(w756) -> ()
                              }
                              frame Error {
                                n295 = local read "Archive Event"() -> (w770:refnum<class "Archive.lvclass">)
                                n296 = control-ref of="Журнал событий"() -> (w768:refnum<vi>)
                                n297 = call "ProcessingJournalEvent.vi"("error IO"=w767, "Журнал событий"=w768, "ArchiveInput"=w770) -> ("Archive Out"=w769:refnum<class "Archive.lvclass">)  [unwired: 8 in]
                                n298 = local write "Archive Event"(w769) -> ()
                              }
                            }
                          }
                          frame True {
                            w784 = u16 2 items=["0", "1", "2", "3", "4", "5", "6", "7"] ("Номер банка программ")
                            n299 = local read "StepMotor"() -> (w774:refnum<class "StepMotor.lvclass">)
                            n300 = local read "Прав.Конц"() -> (w777:bool)
                            n301 = call-dynamic "SetSpeed.vi"("Скорость об/мин"=0.0, "StepMotor in"=w774) -> ("error out"=w775:errorcluster, "StepMotor out"=w776:refnum<class "StepMotor.lvclass">)  [unwired: 8 in]
                            n302 = case shown="True" w777 {
                              frame False {
                              }
                              frame True {
                                n303 = Bundle By Name(cluster=T10 {"Start"=0.0, "Range"=0.0} ("Scale.Scale Position"), "Start"=0.0, "Range"=6.283185307179586) -> (w791:T10)
                                n304 = property on="GaugeAngle" class="Knob (strict)"("Scale.SclPos"=w791) -> ()  [unwired: 2 in, 2 out]
                              }
                            }
                            n305 = call-dynamic "StartProgram.vi"("error in (no error)"=w775, "Номер банка программ"=w784, "StepMotor in"=w776) -> ("error out"=w779:errorcluster, "StepMotor out"=w780:refnum<class "StepMotor.lvclass">)  [unwired: 7 in]
                            n306 = call-dynamic "GetCurrentPositionPulse.vi"("error in (no error)"=w779, "StepMotor in"=w780) -> ("error out"=w772:errorcluster, "Текущая позиция"=w781:dbl, "StepMotor out"=w782:refnum<class "StepMotor.lvclass">)  [unwired: 7 in]
                            n307 = Bundle(cluster=cluster{dbl, dbl} {0.0, 0.0} ("GaugeAngle"), w781) -> (w783:cluster{dbl, dbl})  [unwired: 1 in]
                            n308 = local write "StepMotor"(w782) -> ()
                            n309 = case shown="Error" w772 {
                              frame No Error {
                              }
                              frame Error {
                                n310 = local read "Archive Event"() -> (w786:refnum<class "Archive.lvclass">)
                                n311 = control-ref of="Журнал событий"() -> (w785:refnum<vi>)
                                n312 = call "ProcessingJournalEvent.vi"("Журнал событий"=w785, "ArchiveInput"=w786) -> ("Archive Out"=w787:refnum<class "Archive.lvclass">)  [unwired: 9 in]
                                n313 = local write "Archive Event"(w787) -> ()
                              }
                            }
                            n314 = local read "Лев.Конц"() -> (w778:bool)
                            n315 = local write "GaugeAngle"(w783) -> ()
                            n316 = case shown="True" w778 {
                              frame False {
                              }
                              frame True {
                                n317 = Bundle By Name(cluster=T10 {"Start"=0.0, "Range"=0.0} ("Scale.Scale Position"), "Start"=3.141592653589793, "Range"=6.283185307179586) -> (w795:T10)
                                n318 = property on="GaugeAngle" class="Knob (strict)"("Scale.SclPos"=w795) -> ()  [unwired: 2 in, 2 out]
                              }
                            }
                            n319 = disable-structure shown="Enabled" {
                              frame Enabled {
                                w801 = T6."Enabled" ("Disabled")
                                n320 = property on="Tab Control" class="TabCtl (strict)"() -> ("Pages"=w797:refnum<vi>[])  [unwired: 2 in, 2 out]
                                n321 = local write "ИсхСостСтарСтоп"(FALSE ("ИсхСостСтарСтоп")) -> ()
                                n322 = property on="Запустить цикл" class="Bool (strict)"("DisabledEnum"=w801) -> ()  [unwired: 2 in, 2 out]
                                n323 = property on="Пуск Руч" class="Bool (strict)"("DisabledEnum"=w801) -> ()  [unwired: 2 in, 2 out]
                                n324 = Index Array(array=w797, index=1) -> (element=w799:refnum<vi>)
                                n325 = property class="Page"(reference=w799, "PageVis"=TRUE ("Page Visible")) -> ()  [unwired: 1 in, 2 out]
                              }
                              frame Disabled {
                              }
                            }
                          }
                        }
                      }
                    }
                    n326 = case shown="True" w347 {
                      frame False {
                      }
                      frame True {
                        n327 = local read "Способ управления СПШ"() -> (w400:T3)
                        n328 = case shown="\"Управления скоростью\"" w400 {
                          frame "Управления позицией", Default {
                            n329 = local read "Контроль концевиков"() -> (w415:bool)
                            n330 = local read "Контроль времени"() -> (w417:bool)
                            n331 = case shown="True" w415 {
                              tunnel: [w429 w435] -> w413
                              tunnel: [w429 w434] -> w414
                              tunnel: [w429 w433] -> w412
                              tunnel: [w429 w432] -> w411
                              frame False {
                                w429 = FALSE ("Прав.Конц")
                                n332 = local read "StepMotor"() -> (w427:refnum<class "StepMotor.lvclass">)
                                n333 = local read "StepMotor"() -> (w423:refnum<class "StepMotor.lvclass">)
                                n334 = call-dynamic "GetInputPort.vi"("PortInput"=T9."Порт ввода 1", "StepMotor in"=w427) -> ("error out"=w425:errorcluster, "Состояние"=w419:bool, "StepMotor out"=w426:refnum<class "StepMotor.lvclass">)  [unwired: 7 in]
                                n335 = local write "StepMotor"(w426) -> ()
                                n336 = call-dynamic "GetInputPort.vi"("PortInput"=T9."Порт ввода 2", "StepMotor in"=w423) -> ("error out"=w421:errorcluster, "Состояние"=w420:bool, "StepMotor out"=w422:refnum<class "StepMotor.lvclass">)  [unwired: 7 in]
                                n337 = local write "StepMotor"(w422) -> ()
                                n338 = case shown="No Error" w425 {
                                tunnel: w419 -> [w431 _]
                                frame No Error {
                                n339 = local write "Прав.Конц"(w431) -> ()
                                }
                                frame Error {
                                }
                                }
                                n340 = case shown="No Error" w421 {
                                tunnel: w420 -> [w430 _]
                                frame No Error {
                                n341 = local write "Лев.Конц"(w430) -> ()
                                }
                                frame Error {
                                }
                                }
                              }
                              frame True {
                                n342 = local read "Прав.Конц"() -> (w438:bool)
                                n343 = local read "Лев.Конц"() -> (w439:bool)
                                n344 = local read "Прав.Конц"() -> (w441:bool)
                                n345 = local read "Лев.Конц"() -> (w442:bool)
                                n346 = Not(x=w439) -> (.not. x?=w440:bool)
                                n347 = Not(x=w438) -> (.not. x?=w437:bool)
                                n348 = And(x=w440, y=w437) -> (x .and. y?=w436:bool)
                                n349 = case shown="True" w442 {
                                tunnel: [FALSE w483] -> w434
                                frame False {
                                }
                                frame True {
                                n350 = local read "StepMotor"() -> (w480:refnum<class "StepMotor.lvclass">)
                                n351 = local read "StepMotor"() -> (w486:refnum<class "StepMotor.lvclass">)
                                n352 = call-dynamic "GetInputPort.vi"("PortInput"=T9."Порт ввода 2", "StepMotor in"=w480) -> ("error out"=w482:errorcluster, "Состояние"=w478:bool, "StepMotor out"=w479:refnum<class "StepMotor.lvclass">)  [unwired: 7 in]
                                n353 = local write "StepMotor"(w479) -> ()
                                n354 = call-dynamic "GetInputPort.vi"("PortInput"=T9."Порт ввода 1", "StepMotor in"=w486) -> ("error out"=w484:errorcluster, "Состояние"=w477:bool, "StepMotor out"=w487:refnum<class "StepMotor.lvclass">)  [unwired: 7 in]
                                n355 = local write "StepMotor"(w487) -> ()
                                n356 = case shown="No Error" w484 {
                                tunnel: w477 -> [w489 _]
                                tunnel: [w489 w490] -> w483
                                frame No Error {
                                n357 = local write "Прав.Конц"(w489) -> ()
                                }
                                frame Error {
                                n358 = local read "Прав.Конц"() -> (w490:bool)
                                }
                                }
                                n359 = case shown="No Error" w482 {
                                tunnel: w478 -> [w488 _]
                                frame No Error {
                                n360 = local write "Лев.Конц"(w488) -> ()
                                }
                                frame Error {
                                }
                                }
                                }
                                }
                                n361 = case shown="True" w441 {
                                tunnel: [FALSE w468] -> w435
                                frame False {
                                }
                                frame True {
                                n362 = local read "StepMotor"() -> (w465:refnum<class "StepMotor.lvclass">)
                                n363 = local read "StepMotor"() -> (w471:refnum<class "StepMotor.lvclass">)
                                n364 = call-dynamic "GetInputPort.vi"("PortInput"=T9."Порт ввода 1", "StepMotor in"=w465) -> ("error out"=w467:errorcluster, "Состояние"=w463:bool, "StepMotor out"=w464:refnum<class "StepMotor.lvclass">)  [unwired: 7 in]
                                n365 = local write "StepMotor"(w464) -> ()
                                n366 = call-dynamic "GetInputPort.vi"("PortInput"=T9."Порт ввода 2", "StepMotor in"=w471) -> ("error out"=w469:errorcluster, "Состояние"=w462:bool, "StepMotor out"=w472:refnum<class "StepMotor.lvclass">)  [unwired: 7 in]
                                n367 = local write "StepMotor"(w472) -> ()
                                n368 = case shown="No Error" w467 {
                                tunnel: w463 -> [w473 _]
                                frame No Error {
                                n369 = local write "Прав.Конц"(w473) -> ()
                                }
                                frame Error {
                                }
                                }
                                n370 = case shown="No Error" w469 {
                                tunnel: w462 -> [w474 _]
                                tunnel: [w474 w475] -> w468
                                frame No Error {
                                n371 = local write "Лев.Конц"(w474) -> ()
                                }
                                frame Error {
                                n372 = local read "Лев.Конц"() -> (w475:bool)
                                }
                                }
                                }
                                }
                                n373 = case shown="True" w436 {
                                tunnel: [FALSE w448] -> w433
                                tunnel: [FALSE w453] -> w432
                                frame False {
                                }
                                frame True {
                                n374 = local read "StepMotor"() -> (w450:refnum<class "StepMotor.lvclass">)
                                n375 = local read "StepMotor"() -> (w455:refnum<class "StepMotor.lvclass">)
                                n376 = call-dynamic "GetInputPort.vi"("PortInput"=T9."Порт ввода 2", "StepMotor in"=w450) -> ("error out"=w447:errorcluster, "Состояние"=w446:bool, "StepMotor out"=w449:refnum<class "StepMotor.lvclass">)  [unwired: 7 in]
                                n377 = local write "StepMotor"(w449) -> ()
                                n378 = call-dynamic "GetInputPort.vi"("PortInput"=T9."Порт ввода 1", "StepMotor in"=w455) -> ("error out"=w452:errorcluster, "Состояние"=w445:bool, "StepMotor out"=w454:refnum<class "StepMotor.lvclass">)  [unwired: 7 in]
                                n379 = local write "StepMotor"(w454) -> ()
                                n380 = case shown="No Error" w447 {
                                tunnel: w446 -> [w457 _]
                                tunnel: [w457 w458] -> w448
                                frame No Error {
                                n381 = local write "Лев.Конц"(w457) -> ()
                                }
                                frame Error {
                                n382 = local read "Лев.Конц"() -> (w458:bool)
                                }
                                }
                                n383 = case shown="No Error" w452 {
                                tunnel: w445 -> [w459 _]
                                tunnel: [w459 w460] -> w453
                                frame No Error {
                                n384 = local write "Прав.Конц"(w459) -> ()
                                }
                                frame Error {
                                n385 = local read "Прав.Конц"() -> (w460:bool)
                                }
                                }
                                }
                                }
                              }
                            }
                            n386 = case shown="True" w417 {
                              tunnel: [FALSE ("f") w493] -> w416
                              frame False {
                              }
                              frame True {
                                n387 = local read "Время в мин"() -> (w497:dbl)
                                n388 = local read "Условие время"() -> (w495:bool)
                                n389 = Multiply(x=w497, y=60.0) -> (x*y=w496:dbl)
                                n390 = call "Elapsed Time3"("Time Target (s)"=w496, "Reset"=w495) -> ("Elapsed Time (s)"=w494:dbl, "Time has Elapsed"=w493:bool)  [unwired: 10 in, 6 out]
                                n391 = local write "Лимит времени"(w494) -> ()
                                n392 = local write "Условие время"(w493) -> ()
                              }
                            }
                            n393 = local read "Заданная позиция"() -> (w409:dbl)
                            n394 = local read "Выбег"() -> (w406:dbl)
                            n395 = local read "Текущая позиция"() -> (w407:dbl)
                            n396 = Equal To 0?(x=w406) -> (x = 0?=w410:bool)
                            n397 = Select(t=w409, s=w410, f=w406) -> (s? t:f=w408:dbl)
                            n398 = Equal?(x=w408, y=w407) -> (x = y?=w405:bool)
                            n399 = Compound Arithmetic op=OR(w414, w413, w412, w411, w416, w405) -> (w418:bool)
                            n400 = case shown="False" w418 {
                              frame False {
                                n401 = local read "Разрешение энкодера"() -> (w502:dbl)
                                n402 = local read "StepMotor"() -> (w505:refnum<class "StepMotor.lvclass">)
                                n403 = local read "Редукция"() -> (w503:dbl)
                                n404 = call "GetPositionDegreesPosition.vi"("StepMotor in"=w505, "Редукция"=w503, "Разрешение энкодера"=w502) -> ("StepMotor out"=w504:refnum<class "StepMotor.lvclass">, "Значение"=w501:dbl, "+360 -360"=w500:bool, "+ 0 -"=w499:bool, "error out"=w498:errorcluster)  [unwired: 12 in]
                                n405 = local write "StepMotor"(w504) -> ()
                                n406 = case shown="No Error" w498 {
                                selector: w498 -> [w517 w554]
                                tunnel: w500 -> [w519 _]
                                tunnel: w501 -> [w509 _]
                                tunnel: w499 -> [w518 _]
                                frame No Error {
                                n407 = case shown="True" w519 {
                                tunnel: w517 -> [_ w529]
                                frame False {
                                }
                                frame True {
                                n408 = while {
                                tunnel: [w538] -> w532
                                tunnel: [w537] -> w533
                                tunnel: w529 -> [w536]
                                stop <- w539 stop-if-true
                                n409 = local read "StepMotor"() -> (w544:refnum<class "StepMotor.lvclass">)
                                n410 = call-dynamic "GetPredesignedPosition.vi"("error in (no error)"=w536, "StepMotor in"=w544) -> ("error out"=w545:errorcluster, "Заданная позиция"=w542:dbl, "StepMotor out"=w546:refnum<class "StepMotor.lvclass">)  [unwired: 7 in]
                                n411 = call-dynamic "GetCurrentPositionPulse.vi"("error in (no error)"=w545, "StepMotor in"=w546) -> ("error out"=w538:errorcluster, "Текущая позиция"=w543:dbl, "StepMotor out"=w537:refnum<class "StepMotor.lvclass">)  [unwired: 7 in]
                                n412 = Equal To 0?(x=w543) -> (x = 0?=w541:bool)
                                n413 = Equal To 0?(x=w542) -> (x = 0?=w540:bool)
                                n414 = And(x=w541, y=w540) -> (x .and. y?=w539:bool)
                                }
                                n415 = local read "Напраление вращения"() -> (w535:enum32{"Лево", "Право"})
                                n416 = case shown="\"Лево\", Default" w535 {
                                tunnel: [w551 w553] -> w534
                                frame "Лево", Default {
                                n417 = local read "Выбег"() -> (w552:dbl)
                                n418 = Negate(x=w552) -> (-x=w551:dbl)
                                }
                                frame "Право" {
                                n419 = local read "Выбег"() -> (w553:dbl)
                                }
                                }
                                n420 = call-dynamic "SetPosition.vi"("error in (no error)"=w532, "Позиция"=w534, "StepMotor in"=w533) -> ("error out"=w530:errorcluster, "StepMotor out"=w531:refnum<class "StepMotor.lvclass">)  [unwired: 7 in]
                                n421 = local write "StepMotor"(w531) -> ()
                                n422 = case shown="Error" w530 {
                                selector: w530 -> [_ w547]
                                frame No Error {
                                }
                                frame Error {
                                n423 = local read "Archive Event"() -> (w549:refnum<class "Archive.lvclass">)
                                n424 = control-ref of="Журнал событий"() -> (w548:refnum<vi>)
                                n425 = call "ProcessingJournalEvent.vi"("error IO"=w547, "Журнал событий"=w548, "ArchiveInput"=w549) -> ("Archive Out"=w550:refnum<class "Archive.lvclass">)  [unwired: 8 in]
                                n426 = local write "Archive Event"(w550) -> ()
                                }
                                }
                                }
                                }
                                n427 = case shown="True" w518 {
                                frame False {
                                }
                                frame True {
                                n428 = local read "Напраление вращения"() -> (w526:enum32{"Лево", "Право"})
                                n429 = case shown="\"Лево\", Default" w526 {
                                frame "Лево", Default {
                                n430 = property on="GaugeAngle" class="Knob (strict)"("Scale.Flipped"=TRUE) -> ()  [unwired: 2 in, 2 out]
                                }
                                frame "Право" {
                                n431 = property on="GaugeAngle" class="Knob (strict)"("Scale.Flipped"=FALSE) -> ()  [unwired: 2 in, 2 out]
                                }
                                }
                                }
                                }
                                n432 = local read "Текущая позиция"() -> (w514:dbl)
                                n433 = call "GetCurentDateTime.vi"() -> ("time"=w512:string)  [unwired: 2 in, 1 out]
                                n434 = Number To Fractional String(number=w514) -> (F-format string=w515:string)  [unwired: 3 in]
                                n435 = Number To Fractional String(number=w509) -> (F-format string=w508:string)  [unwired: 3 in]
                                n436 = Bundle(cluster=cluster{dbl, dbl} {0.0, 0.0} ("GaugeAngle"), w509) -> (w520:cluster{dbl, dbl})  [unwired: 1 in]
                                n437 = local write "GaugeAngle"(w520) -> ()
                                n438 = local read "Archive Data"() -> (w510:refnum<class "Archive.lvclass">)
                                n439 = Build Array("", w512, w515, w508) -> (w516:string[])
                                n440 = call-dynamic "WriteInFileArchive.vi"("Строка таблицы"=w516, "Archive in"=w510) -> ("error out"=w507:errorcluster, "Archive out"=w511:refnum<class "Archive.lvclass">)  [unwired: 8 in]
                                n441 = local write "Archive Data"(w511) -> ()
                                n442 = case shown="Error" w507 {
                                selector: w507 -> [_ w522]
                                frame No Error {
                                }
                                frame Error {
                                n443 = local read "Archive Event"() -> (w524:refnum<class "Archive.lvclass">)
                                n444 = control-ref of="Журнал событий"() -> (w525:refnum<vi>)
                                n445 = call "ProcessingJournalEvent.vi"("error IO"=w522, "Новая строка в журнале"="Нет доступа к файлу, возможно файл открыт другой програмой!!!", "Журнал событий"=w525, "ArchiveInput"=w524) -> ("Archive Out"=w523:refnum<class "Archive.lvclass">)  [unwired: 7 in]
                                n446 = local write "Archive Event"(w523) -> ()
                                }
                                }
                                }
                                frame Error {
                                n447 = local read "Archive Event"() -> (w556:refnum<class "Archive.lvclass">)
                                n448 = control-ref of="Журнал событий"() -> (w555:refnum<vi>)
                                n449 = call "ProcessingJournalEvent.vi"("error IO"=w554, "Журнал событий"=w555, "ArchiveInput"=w556) -> ("Archive Out"=w557:refnum<class "Archive.lvclass">)  [unwired: 8 in]
                                n450 = local write "Archive Event"(w557) -> ()
                                }
                                }
                              }
                              frame True {
                                n451 = flat-sequence {
                                tunnel: [w560] -> w558
                                tunnel: w558 -> [w562]
                                frame #0 {
                                n452 = property on="Стоп Руч" class="Bool (strict)"("Val(Sgnl)"=TRUE ("Value (Signaling)")) -> (error out=w560:errorcluster)  [unwired: 2 in, 1 out]
                                }
                                frame #1 {
                                n453 = property on="Стоп Руч" class="Bool (strict)"(error in=w562, "Val(Sgnl)"=FALSE ("Value (Signaling)")) -> ()  [unwired: 1 in, 2 out]
                                }
                                }
                              }
                            }
                          }
                          frame "Управления скоростью" {
                            n454 = local read "Контроль энкодера"() -> (w564:bool)
                            n455 = local read "Контроль концевиков"() -> (w563:bool)
                            n456 = local read "Контроль времени"() -> (w566:bool)
                            n457 = case shown="True" w566 {
                              tunnel: [FALSE ("f") w664] -> w567
                              frame False {
                              }
                              frame True {
                                n458 = local read "Время в мин"() -> (w668:dbl)
                                n459 = local read "Условие время"() -> (w666:bool)
                                n460 = Multiply(x=w668, y=60.0) -> (x*y=w667:dbl)
                                n461 = call "Elapsed Time"("Time Target (s)"=w667, "Reset"=w666) -> ("Elapsed Time (s)"=w665:dbl, "Time has Elapsed"=w664:bool)  [unwired: 10 in, 6 out]
                                n462 = local write "Лимит времени"(w665) -> ()
                                n463 = local write "Условие время"(w664) -> ()
                              }
                            }
                            n464 = case shown="True" w564 {
                              tunnel: [FALSE ("f") w650] -> w565
                              frame False {
                              }
                              frame True {
                                n465 = local read "Инкремент импульсов"() -> (w648:dbl)
                                n466 = local read "Редукция"() -> (w647:dbl)
                                n467 = local read "Разрешение энкодера"() -> (w646:dbl)
                                n468 = local read "StepMotor"() -> (w653:refnum<class "StepMotor.lvclass">)
                                n469 = call "GetPositionDegreeInc.vi"("StepMotor in"=w653, "IncImpulsIn"=w648, "Редукция"=w647, "Разрешение энкодера"=w646) -> ("StepMotor out"=w652:refnum<class "StepMotor.lvclass">, "IncImpulsOut"=w651:dbl, "error out"=w649:errorcluster)  [unwired: 13 in]
                                n470 = local write "StepMotor"(w652) -> ()
                                n471 = case shown="No Error" w649 {
                                selector: w649 -> [_ w657]
                                tunnel: w651 -> [w656 _]
                                tunnel: [w654 w661] -> w650
                                frame No Error {
                                n472 = local write "Инкремент импульсов"(w656) -> ()
                                n473 = local read "Значение энкодера"() -> (w655:dbl)
                                n474 = Greater?(x=w656, y=w655) -> (0:w654:bool)
                                n475 = local write "Условие энкодер"(w654) -> ()
                                }
                                frame Error {
                                n476 = local read "Archive Event"() -> (w659:refnum<class "Archive.lvclass">)
                                n477 = control-ref of="Журнал событий"() -> (w660:refnum<vi>)
                                n478 = call "ProcessingJournalEvent.vi"("error IO"=w657, "Журнал событий"=w660, "ArchiveInput"=w659) -> ("Archive Out"=w658:refnum<class "Archive.lvclass">)  [unwired: 8 in]
                                n479 = local write "Archive Event"(w658) -> ()
                                n480 = local read "Условие энкодер"() -> (w661:bool)
                                }
                                }
                              }
                            }
                            n481 = case shown="True" w563 {
                              tunnel: [w583 w589] -> w571
                              tunnel: [w583 w588] -> w570
                              tunnel: [w583 w587] -> w569
                              tunnel: [w583 w586] -> w568
                              frame False {
                                w583 = FALSE ("Прав.Конц")
                                n482 = local read "StepMotor"() -> (w581:refnum<class "StepMotor.lvclass">)
                                n483 = local read "StepMotor"() -> (w577:refnum<class "StepMotor.lvclass">)
                                n484 = call-dynamic "GetInputPort.vi"("PortInput"=T9."Порт ввода 1", "StepMotor in"=w581) -> ("error out"=w579:errorcluster, "Состояние"=w573:bool, "StepMotor out"=w580:refnum<class "StepMotor.lvclass">)  [unwired: 7 in]
                                n485 = local write "StepMotor"(w580) -> ()
                                n486 = call-dynamic "GetInputPort.vi"("PortInput"=T9."Порт ввода 2", "StepMotor in"=w577) -> ("error out"=w575:errorcluster, "Состояние"=w574:bool, "StepMotor out"=w576:refnum<class "StepMotor.lvclass">)  [unwired: 7 in]
                                n487 = local write "StepMotor"(w576) -> ()
                                n488 = case shown="No Error" w579 {
                                tunnel: w573 -> [w585 _]
                                frame No Error {
                                n489 = local write "Прав.Конц"(w585) -> ()
                                }
                                frame Error {
                                }
                                }
                                n490 = case shown="No Error" w575 {
                                tunnel: w574 -> [w584 _]
                                frame No Error {
                                n491 = local write "Лев.Конц"(w584) -> ()
                                }
                                frame Error {
                                }
                                }
                              }
                              frame True {
                                n492 = local read "Прав.Конц"() -> (w592:bool)
                                n493 = local read "Лев.Конц"() -> (w593:bool)
                                n494 = local read "Прав.Конц"() -> (w595:bool)
                                n495 = local read "Лев.Конц"() -> (w596:bool)
                                n496 = Not(x=w593) -> (.not. x?=w594:bool)
                                n497 = Not(x=w592) -> (.not. x?=w591:bool)
                                n498 = And(x=w594, y=w591) -> (x .and. y?=w590:bool)
                                n499 = case shown="True" w596 {
                                tunnel: [FALSE w637] -> w588
                                frame False {
                                }
                                frame True {
                                n500 = local read "StepMotor"() -> (w634:refnum<class "StepMotor.lvclass">)
                                n501 = local read "StepMotor"() -> (w640:refnum<class "StepMotor.lvclass">)
                                n502 = call-dynamic "GetInputPort.vi"("PortInput"=T9."Порт ввода 2", "StepMotor in"=w634) -> ("error out"=w636:errorcluster, "Состояние"=w632:bool, "StepMotor out"=w633:refnum<class "StepMotor.lvclass">)  [unwired: 7 in]
                                n503 = local write "StepMotor"(w633) -> ()
                                n504 = call-dynamic "GetInputPort.vi"("PortInput"=T9."Порт ввода 1", "StepMotor in"=w640) -> ("error out"=w638:errorcluster, "Состояние"=w631:bool, "StepMotor out"=w641:refnum<class "StepMotor.lvclass">)  [unwired: 7 in]
                                n505 = local write "StepMotor"(w641) -> ()
                                n506 = case shown="No Error" w638 {
                                tunnel: w631 -> [w643 _]
                                tunnel: [w643 w644] -> w637
                                frame No Error {
                                n507 = local write "Прав.Конц"(w643) -> ()
                                }
                                frame Error {
                                n508 = local read "Прав.Конц"() -> (w644:bool)
                                }
                                }
                                n509 = case shown="No Error" w636 {
                                tunnel: w632 -> [w642 _]
                                frame No Error {
                                n510 = local write "Лев.Конц"(w642) -> ()
                                }
                                frame Error {
                                }
                                }
                                }
                                }
                                n511 = case shown="True" w595 {
                                tunnel: [FALSE w622] -> w589
                                frame False {
                                }
                                frame True {
                                n512 = local read "StepMotor"() -> (w619:refnum<class "StepMotor.lvclass">)
                                n513 = local read "StepMotor"() -> (w625:refnum<class "StepMotor.lvclass">)
                                n514 = call-dynamic "GetInputPort.vi"("PortInput"=T9."Порт ввода 1", "StepMotor in"=w619) -> ("error out"=w621:errorcluster, "Состояние"=w617:bool, "StepMotor out"=w618:refnum<class "StepMotor.lvclass">)  [unwired: 7 in]
                                n515 = local write "StepMotor"(w618) -> ()
                                n516 = call-dynamic "GetInputPort.vi"("PortInput"=T9."Порт ввода 2", "StepMotor in"=w625) -> ("error out"=w623:errorcluster, "Состояние"=w616:bool, "StepMotor out"=w626:refnum<class "StepMotor.lvclass">)  [unwired: 7 in]
                                n517 = local write "StepMotor"(w626) -> ()
                                n518 = case shown="No Error" w621 {
                                tunnel: w617 -> [w627 _]
                                frame No Error {
                                n519 = local write "Прав.Конц"(w627) -> ()
                                }
                                frame Error {
                                }
                                }
                                n520 = case shown="No Error" w623 {
                                tunnel: w616 -> [w628 _]
                                tunnel: [w628 w629] -> w622
                                frame No Error {
                                n521 = local write "Лев.Конц"(w628) -> ()
                                }
                                frame Error {
                                n522 = local read "Лев.Конц"() -> (w629:bool)
                                }
                                }
                                }
                                }
                                n523 = case shown="True" w590 {
                                tunnel: [FALSE w602] -> w587
                                tunnel: [FALSE w607] -> w586
                                frame False {
                                }
                                frame True {
                                n524 = local read "StepMotor"() -> (w604:refnum<class "StepMotor.lvclass">)
                                n525 = local read "StepMotor"() -> (w609:refnum<class "StepMotor.lvclass">)
                                n526 = call-dynamic "GetInputPort.vi"("PortInput"=T9."Порт ввода 2", "StepMotor in"=w604) -> ("error out"=w601:errorcluster, "Состояние"=w600:bool, "StepMotor out"=w603:refnum<class "StepMotor.lvclass">)  [unwired: 7 in]
                                n527 = local write "StepMotor"(w603) -> ()
                                n528 = call-dynamic "GetInputPort.vi"("PortInput"=T9."Порт ввода 1", "StepMotor in"=w609) -> ("error out"=w606:errorcluster, "Состояние"=w599:bool, "StepMotor out"=w608:refnum<class "StepMotor.lvclass">)  [unwired: 7 in]
                                n529 = local write "StepMotor"(w608) -> ()
                                n530 = case shown="No Error" w601 {
                                tunnel: w600 -> [w611 _]
                                tunnel: [w611 w612] -> w602
                                frame No Error {
                                n531 = local write "Лев.Конц"(w611) -> ()
                                }
                                frame Error {
                                n532 = local read "Лев.Конц"() -> (w612:bool)
                                }
                                }
                                n533 = case shown="No Error" w606 {
                                tunnel: w599 -> [w613 _]
                                tunnel: [w613 w614] -> w607
                                frame No Error {
                                n534 = local write "Прав.Конц"(w613) -> ()
                                }
                                frame Error {
                                n535 = local read "Прав.Конц"() -> (w614:bool)
                                }
                                }
                                }
                                }
                              }
                            }
                            n536 = Compound Arithmetic op=OR(w570, w571, w569, w568, w567, w565) -> (w572:bool)
                            n537 = case shown="False" w572 {
                              frame False {
                                n538 = local read "Разрешение энкодера"() -> (w674:dbl)
                                n539 = local read "StepMotor"() -> (w676:refnum<class "StepMotor.lvclass">)
                                n540 = local read "Редукция"() -> (w675:dbl)
                                n541 = call "GetPositionDegreesSpeed.vi"("StepMotor in"=w676, "Редукция"=w675, "Разрешение энкодера"=w674) -> ("StepMotor out"=w673:refnum<class "StepMotor.lvclass">, "Значение"=w672:dbl, "+360 -360"=w669:bool, "+ 0 -"=w670:bool, "error out"=w671:errorcluster)  [unwired: 12 in]
                                n542 = local write "StepMotor"(w673) -> ()
                                n543 = case shown="No Error" w671 {
                                selector: w671 -> [_ w694]
                                tunnel: w672 -> [w678 _]
                                tunnel: w670 -> [w688 _]
                                tunnel: w669 -> [w689 _]
                                frame No Error {
                                n544 = Or(x=w689, y=w688) -> (x .or. y?=w687:bool)
                                n545 = case shown="True" w687 {
                                frame False {
                                }
                                frame True {
                                n546 = local read "Напраление вращения"() -> (w691:enum32{"Лево", "Право"})
                                n547 = case shown="\"Лево\", Default" w691 {
                                frame "Лево", Default {
                                n548 = property on="GaugeAngle" class="Knob (strict)"("Scale.Flipped"=TRUE) -> ()  [unwired: 2 in, 2 out]
                                }
                                frame "Право" {
                                n549 = property on="GaugeAngle" class="Knob (strict)"("Scale.Flipped"=FALSE) -> ()  [unwired: 2 in, 2 out]
                                }
                                }
                                }
                                }
                                n550 = local read "Текущая позиция"() -> (w684:dbl)
                                n551 = Bundle(cluster=cluster{dbl, dbl} {0.0, 0.0} ("GaugeAngle"), w678) -> (w690:cluster{dbl, dbl})  [unwired: 1 in]
                                n552 = local write "GaugeAngle"(w690) -> ()
                                n553 = call "GetCurentDateTime.vi"() -> ("time"=w682:string)  [unwired: 2 in, 1 out]
                                n554 = Number To Fractional String(number=w684) -> (F-format string=w685:string)  [unwired: 3 in]
                                n555 = Number To Fractional String(number=w678) -> (F-format string=w679:string)  [unwired: 3 in]
                                n556 = local read "Archive Data"() -> (w680:refnum<class "Archive.lvclass">)
                                n557 = Build Array("", w682, w685, w679) -> (w686:string[])
                                n558 = call-dynamic "WriteInFileArchive.vi"("Строка таблицы"=w686, "Archive in"=w680) -> ("Archive out"=w681:refnum<class "Archive.lvclass">)  [unwired: 8 in, 1 out]
                                n559 = local write "Archive Data"(w681) -> ()
                                }
                                frame Error {
                                n560 = local read "Archive Event"() -> (w697:refnum<class "Archive.lvclass">)
                                n561 = control-ref of="Журнал событий"() -> (w695:refnum<vi>)
                                n562 = call "ProcessingJournalEvent.vi"("error IO"=w694, "Журнал событий"=w695, "ArchiveInput"=w697) -> ("Archive Out"=w696:refnum<class "Archive.lvclass">)  [unwired: 8 in]
                                n563 = local write "Archive Event"(w696) -> ()
                                }
                                }
                              }
                              frame True {
                                n564 = flat-sequence {
                                tunnel: [w700] -> w698
                                tunnel: w698 -> [w702]
                                frame #0 {
                                n565 = property on="Стоп Руч" class="Bool (strict)"("Val(Sgnl)"=TRUE ("Value (Signaling)")) -> (error out=w700:errorcluster)  [unwired: 2 in, 1 out]
                                }
                                frame #1 {
                                n566 = property on="Стоп Руч" class="Bool (strict)"(error in=w702, "Val(Sgnl)"=FALSE ("Value (Signaling)")) -> ()  [unwired: 1 in, 2 out]
                                }
                                }
                              }
                            }
                          }
                        }
                        n567 = local read "StepMotor"() -> (w398:refnum<class "StepMotor.lvclass">)
                        n568 = call-dynamic "GetCurrentPositionPulse.vi"("StepMotor in"=w398) -> ("error out"=w395:errorcluster, "Текущая позиция"=w397:dbl, "StepMotor out"=w399:refnum<class "StepMotor.lvclass">)  [unwired: 8 in]
                        n569 = local write "StepMotor"(w399) -> ()
                        n570 = Merge Signals(w397) -> (w396:dynamicdata)
                        n571 = local write "Текущая позиция"(w397) -> ()
                        n572 = local write "Waveform Chart"(w396) -> ()
                        n573 = case shown="Error" w395 {
                          selector: w395 -> [_ w401]
                          frame No Error {
                          }
                          frame Error {
                            n574 = local read "Archive Event"() -> (w403:refnum<class "Archive.lvclass">)
                            n575 = control-ref of="Журнал событий"() -> (w402:refnum<vi>)
                            n576 = call "ProcessingJournalEvent.vi"("error IO"=w401, "Журнал событий"=w402, "ArchiveInput"=w403) -> ("Archive Out"=w404:refnum<class "Archive.lvclass">)  [unwired: 8 in]
                            n577 = local write "Archive Event"(w404) -> ()
                          }
                        }
                      }
                    }
                    n578 = disable-structure shown="Enabled" {
                      frame Enabled {
                        n579 = local read "ИсхСостСтарСтоп"() -> (w351:bool)
                        n580 = local read "РучнойСтартСтоп"() -> (w349:bool)
                        n581 = Compound Arithmetic op=OR(w351, w349) -> (w350:bool)
                        n582 = case shown="False" w350 {
                          frame False {
                            n583 = local read "StepMotor"() -> (w363:refnum<class "StepMotor.lvclass">)
                            n584 = local read "Разрешение энкодера"() -> (w364:dbl)
                            n585 = call-dynamic "GetInputPort.vi"("PortInput"=T9."Порт ввода 1", "StepMotor in"=w363) -> ("error out"=w361:errorcluster, "Состояние"=w360:bool, "StepMotor out"=w362:refnum<class "StepMotor.lvclass">)  [unwired: 7 in]
                            n586 = local read "Редукция"() -> (w365:dbl)
                            n587 = call-dynamic "GetInputPort.vi"("error in (no error)"=w361, "PortInput"=T9."Порт ввода 2", "StepMotor in"=w362) -> ("error out"=w357:errorcluster, "Состояние"=w359:bool, "StepMotor out"=w358:refnum<class "StepMotor.lvclass">)  [unwired: 6 in]
                            n588 = call "GetPositionDegreesSpeed.vi"("StepMotor in"=w358, "Редукция"=w365, "Разрешение энкодера"=w364, "error in (no error)"=w357) -> ("StepMotor out"=w356:refnum<class "StepMotor.lvclass">, "Значение"=w354:dbl, "error out"=w355:errorcluster)  [unwired: 11 in, 2 out]
                            n589 = call-dynamic "GetStatusSPS.vi"("error in (no error)"=w355, "StepMotor in"=w356) -> ("error out"=w353:errorcluster, "StatusController"=w352:T1, "StepMotor out"=w366:refnum<class "StepMotor.lvclass">)  [unwired: 7 in]
                            n590 = local write "StepMotor"(w366) -> ()
                            n591 = case shown="No Error" w353 {
                              selector: w353 -> [_ w378]
                              tunnel: w360 -> [w373 _]
                              tunnel: w359 -> [w372 _]
                              tunnel: w354 -> [w371 _]
                              tunnel: w352 -> [w370 _]
                              frame No Error {
                                n592 = local write "Прав.Конц"(w373) -> ()
                                n593 = local write "Лев.Конц"(w372) -> ()
                                n594 = Equal To 0?(x=w370) -> (x = 0?=w374:bool)
                                n595 = local write "Статус контроллера СПШ"(w370) -> ()
                                n596 = case shown="False" w374 {
                                frame False {
                                n597 = local write "Индикатор Статуса Конт"(TRUE ("Индикатор Статуса Конт")) -> ()
                                }
                                frame True {
                                n598 = local write "Индикатор Статуса Конт"(FALSE ("Индикатор Статуса Конт")) -> ()
                                }
                                }
                                n599 = Bundle(cluster=cluster{dbl, dbl} {0.0, 0.0} ("GaugeAngle"), w371) -> (w375:cluster{dbl, dbl})  [unwired: 1 in]
                                n600 = local write "GaugeAngle"(w375) -> ()
                              }
                              frame Error {
                                n601 = local read "Archive Event"() -> (w382:refnum<class "Archive.lvclass">)
                                n602 = control-ref of="Журнал событий"() -> (w380:refnum<vi>)
                                n603 = call <vilib>:"Simple Error Handler.vi"("error in (no error)"=w378) -> ()  [unwired: 4 in, 5 out]
                                n604 = call "ProcessingJournalEvent.vi"("error IO"=w378, "Новая строка в журнале"="Возможно, потеряна связь с двигателем!!! ", "Журнал событий"=w380, "ArchiveInput"=w382) -> ("Archive Out"=w381:refnum<class "Archive.lvclass">)  [unwired: 7 in]
                                n605 = local write "Archive Event"(w381) -> ()
                              }
                            }
                          }
                          frame True {
                            n606 = local read "StepMotor"() -> (w385:refnum<class "StepMotor.lvclass">)
                            n607 = call-dynamic "GetStatusSPS.vi"("StepMotor in"=w385) -> ("error out"=w383:errorcluster, "StatusController"=w386:T1, "StepMotor out"=w384:refnum<class "StepMotor.lvclass">)  [unwired: 8 in]
                            n608 = case shown="No Error" w383 {
                              selector: w383 -> [_ w392]
                              tunnel: w386 -> [w387 _]
                              frame No Error {
                                n609 = Equal To 0?(x=w387) -> (x = 0?=w388:bool)
                                n610 = case shown="False" w388 {
                                frame False {
                                n611 = local write "Индикатор Статуса Конт"(TRUE ("Индикатор Статуса Конт")) -> ()
                                }
                                frame True {
                                n612 = local write "Индикатор Статуса Конт"(FALSE ("Индикатор Статуса Конт")) -> ()
                                }
                                }
                                n613 = local write "Статус контроллера СПШ"(w387) -> ()
                              }
                              frame Error {
                                n614 = local read "Archive Event"() -> (w394:refnum<class "Archive.lvclass">)
                                n615 = control-ref of="Журнал событий"() -> (w391:refnum<vi>)
                                n616 = call "ProcessingJournalEvent.vi"("error IO"=w392, "Журнал событий"=w391, "ArchiveInput"=w394) -> ("Archive Out"=w393:refnum<class "Archive.lvclass">)  [unwired: 8 in]
                                n617 = local write "Archive Event"(w393) -> ()
                              }
                            }
                            n618 = local write "StepMotor"(w384) -> ()
                          }
                        }
                      }
                      frame Disabled {
                      }
                    }
                  }
                }
              }
              event "Скорость передачи": Value Change {
                n619 = event-data() -> ("NewVal"=w831:i32)  [unwired: 1 in, 5 out]
                n620 = property on="Скорость передачи" class="Ring (strict)"() -> ("Strings []"=w832:string[])  [unwired: 2 in, 2 out]
                n621 = Index Array(array=w832, index=w831) -> (element=w830:string)
                n622 = Decimal String To Number(string=w830) -> (number=w829:i32)  [unwired: 2 in, 1 out]
                n623 = local read "Имя порта"() -> (w827:refnum<visa-resource-name>)
                n624 = To Unsigned Long Integer(number=w829) -> (unsigned 32bit integer=w828:u32)
                n625 = call "InitPort.vi"("Скорость передачи"=w828, "Порт"=w827) -> ("error out"=w823:errorcluster, "StepMotor out"=w824:refnum<class "StepMotor.lvclass">)  [unwired: 8 in]
                n626 = call-dynamic "CloseCommunications .vi"("error in (no error)"=w823, "StepMotor in"=w824) -> ("error out"=w825:errorcluster, "StepMotor out"=w826:refnum<class "StepMotor.lvclass">)  [unwired: 8 in]
                n627 = local read "Разрешение энкодера"() -> (w817:dbl)
                n628 = call-dynamic "OpenCommunications .vi"("error in (no error)"=w825, "StepMotor in"=w826) -> ("error out"=w810:errorcluster, "StepMotor out"=w811:refnum<class "StepMotor.lvclass">)  [unwired: 8 in]
                n629 = call-dynamic "GetInputPort.vi"("error in (no error)"=w810, "PortInput"=T9."Порт ввода 1", "StepMotor in"=w811) -> ("error out"=w818:errorcluster, "Состояние"=w803:bool, "StepMotor out"=w819:refnum<class "StepMotor.lvclass">)  [unwired: 6 in]
                n630 = local read "Редукция"() -> (w816:dbl)
                n631 = call-dynamic "GetInputPort.vi"("error in (no error)"=w818, "PortInput"=T9."Порт ввода 2", "StepMotor in"=w819) -> ("error out"=w814:errorcluster, "Состояние"=w802:bool, "StepMotor out"=w815:refnum<class "StepMotor.lvclass">)  [unwired: 6 in]
                n632 = call "GetPositionDegreesSpeed.vi"("StepMotor in"=w815, "Редукция"=w816, "Разрешение энкодера"=w817, "error in (no error)"=w814) -> ("StepMotor out"=w813:refnum<class "StepMotor.lvclass">, "Значение"=w804:dbl, "error out"=w812:errorcluster)  [unwired: 11 in, 2 out]
                n633 = call-dynamic "GetResolutionEnc.vi"("error in (no error)"=w812, "StepMotor in"=w813) -> ("error out"=w808:errorcluster, "Разрешение энкодера"=w805:dbl, "StepMotor out"=w809:refnum<class "StepMotor.lvclass">)  [unwired: 7 in]
                n634 = call-dynamic "GetModulationPWM.vi"("error in (no error)"=w808, "StepMotor in"=w809) -> ("error out"=w807:errorcluster, "Значение"=w806:bool, "StepMotor out"=w822:refnum<class "StepMotor.lvclass">)  [unwired: 7 in]
                n635 = local write "StepMotor"(w822) -> ()
                n636 = case shown="Error" w807 {
                  selector: w807 -> [_ w857]
                  tunnel: w806 -> [w839 _]
                  tunnel: w805 -> [w837 _]
                  tunnel: w804 -> [w836 _]
                  tunnel: w803 -> [w835 _]
                  tunnel: w802 -> [w834 _]
                  frame No Error {
                    n637 = local write "Прав.Конц"(w835) -> ()
                    n638 = local write "Лев.Конц"(w834) -> ()
                    n639 = local write "Разрешение энкодера"(w837) -> ()
                    n640 = local write "Статус связи с СПШ"(TRUE ("Статус связи с СПШ")) -> ()
                    n641 = Not(x=w839) -> (.not. x?=w840:bool)
                    n642 = property on="Скорость передачи" class="Ring (strict)"() -> ("RingText.Text"=w849:string)  [unwired: 2 in, 2 out]
                    n643 = local write "Останов"(w840) -> ()
                    n644 = Bundle(cluster=cluster{dbl, dbl} {0.0, 0.0} ("GaugeAngle"), w836) -> (w838:cluster{dbl, dbl})  [unwired: 1 in]
                    n645 = property on="Имя порта" class="VISAName"() -> ("Text.Text"=w847:string)  [unwired: 2 in, 2 out]
                    n646 = local read "Archive Event"() -> (w843:refnum<class "Archive.lvclass">)
                    n647 = local write "GaugeAngle"(w838) -> ()
                    n648 = control-ref of="Журнал событий"() -> (w844:refnum<vi>)
                    n649 = Concatenate Strings("После изменения скорости на " ("Новая строка в журнале"), w849, ", связь с портом " ("string"), w847, " установлена..." ("string")) -> (w845:string)
                    n650 = call "ProcessingJournalEvent.vi"("Новая строка в журнале"=w845, "Журнал событий"=w844, "ArchiveInput"=w843) -> ("Archive Out"=w842:refnum<class "Archive.lvclass">)  [unwired: 8 in]
                    n651 = property on="Останов" class="Bool (strict)"("DisabledEnum"=T6."Enabled" ("Disabled")) -> ()  [unwired: 2 in, 2 out]
                    n652 = local write "Archive Event"(w842) -> ()
                  }
                  frame Error {
                    n653 = local write "Статус связи с СПШ"(FALSE ("Статус связи с СПШ")) -> ()
                    n654 = property on="Скорость передачи" class="Ring (strict)"() -> ("RingText.Text"=w861:string)  [unwired: 2 in, 2 out]
                    n655 = property on="Имя порта" class="VISAName"() -> ("Text.Text"=w859:string)  [unwired: 2 in, 2 out]
                    n656 = local read "Archive Event"() -> (w854:refnum<class "Archive.lvclass">)
                    n657 = property on="Останов" class="Bool (strict)"("DisabledEnum"=T6."Disabled and Grayed Out" ("Disabled")) -> ()  [unwired: 2 in, 2 out]
                    n658 = control-ref of="Журнал событий"() -> (w855:refnum<vi>)
                    n659 = Concatenate Strings("После изменения скорости на " ("Новая строка в журнале"), w861, ", связь с портом " ("string"), w859, " не установлена..." ("string")) -> (w856:string)
                    n660 = call "ProcessingJournalEvent.vi"("error IO"=w857, "Новая строка в журнале"=w856, "Журнал событий"=w855, "ArchiveInput"=w854) -> ("Archive Out"=w853:refnum<class "Archive.lvclass">)  [unwired: 7 in]
                    n661 = local write "Archive Event"(w853) -> ()
                  }
                }
              }
              event "Имя порта": Value Change {
                n662 = event-data() -> ("NewVal"=w889:refnum<visa-resource-name>)  [unwired: 1 in, 5 out]
                n663 = local read "Скорость передачи"() -> (w890:i32)
                n664 = property on="Скорость передачи" class="Ring (strict)"() -> ("Strings []"=w894:string[])  [unwired: 2 in, 2 out]
                n665 = Index Array(array=w894, index=w890) -> (element=w893:string)
                n666 = Decimal String To Number(string=w893) -> (number=w892:i32)  [unwired: 2 in, 1 out]
                n667 = To Unsigned Long Integer(number=w892) -> (unsigned 32bit integer=w891:u32)
                n668 = call "InitPort.vi"("Скорость передачи"=w891, "Порт"=w889) -> ("error out"=w887:errorcluster, "StepMotor out"=w888:refnum<class "StepMotor.lvclass">)  [unwired: 8 in]
                n669 = call-dynamic "CloseCommunications .vi"("error in (no error)"=w887, "StepMotor in"=w888) -> ("error out"=w885:errorcluster, "StepMotor out"=w886:refnum<class "StepMotor.lvclass">)  [unwired: 8 in]
                n670 = local read "Разрешение энкодера"() -> (w879:dbl)
                n671 = call-dynamic "OpenCommunications .vi"("error in (no error)"=w885, "StepMotor in"=w886) -> ("error out"=w874:errorcluster, "StepMotor out"=w875:refnum<class "StepMotor.lvclass">)  [unwired: 8 in]
                n672 = call-dynamic "GetInputPort.vi"("error in (no error)"=w874, "PortInput"=T9."Порт ввода 1", "StepMotor in"=w875) -> ("error out"=w880:errorcluster, "Состояние"=w871:bool, "StepMotor out"=w881:refnum<class "StepMotor.lvclass">)  [unwired: 6 in]
                n673 = local read "Редукция"() -> (w878:dbl)
                n674 = call-dynamic "GetInputPort.vi"("error in (no error)"=w880, "PortInput"=T9."Порт ввода 2", "StepMotor in"=w881) -> ("error out"=w876:errorcluster, "Состояние"=w870:bool, "StepMotor out"=w877:refnum<class "StepMotor.lvclass">)  [unwired: 6 in]
                n675 = call "GetPositionDegreesSpeed.vi"("StepMotor in"=w877, "Редукция"=w878, "Разрешение энкодера"=w879, "error in (no error)"=w876) -> ("StepMotor out"=w869:refnum<class "StepMotor.lvclass">, "Значение"=w872:dbl, "error out"=w868:errorcluster)  [unwired: 11 in, 2 out]
                n676 = call-dynamic "GetResolutionEnc.vi"("error in (no error)"=w868, "StepMotor in"=w869) -> ("error out"=w866:errorcluster, "Разрешение энкодера"=w865:dbl, "StepMotor out"=w867:refnum<class "StepMotor.lvclass">)  [unwired: 7 in]
                n677 = call-dynamic "GetModulationPWM.vi"("error in (no error)"=w866, "StepMotor in"=w867) -> ("error out"=w864:errorcluster, "Значение"=w873:bool, "StepMotor out"=w884:refnum<class "StepMotor.lvclass">)  [unwired: 7 in]
                n678 = local write "StepMotor"(w884) -> ()
                n679 = case shown="Error" w864 {
                  selector: w864 -> [_ w917]
                  tunnel: w873 -> [w901 _]
                  tunnel: w872 -> [w899 _]
                  tunnel: w871 -> [w898 _]
                  tunnel: w870 -> [w897 _]
                  tunnel: w865 -> [w896 _]
                  frame No Error {
                    n680 = local write "Прав.Конц"(w898) -> ()
                    n681 = local write "Лев.Конц"(w897) -> ()
                    n682 = local write "Разрешение энкодера"(w896) -> ()
                    n683 = Not(x=w901) -> (.not. x?=w902:bool)
                    n684 = local write "Статус связи с СПШ"(TRUE ("Статус связи с СПШ")) -> ()
                    n685 = property on="Останов" class="Bool (strict)"("DisabledEnum"=T6."Enabled" ("Disabled")) -> ()  [unwired: 2 in, 2 out]
                    n686 = local write "Останов"(w902) -> ()
                    n687 = Bundle(cluster=cluster{dbl, dbl} {0.0, 0.0} ("GaugeAngle"), w899) -> (w900:cluster{dbl, dbl})  [unwired: 1 in]
                    n688 = local write "GaugeAngle"(w900) -> ()
                    n689 = local read "Archive Event"() -> (w905:refnum<class "Archive.lvclass">)
                    n690 = property on="Имя порта" class="VISAName"() -> ("Text.Text"=w909:string)  [unwired: 2 in, 2 out]
                    n691 = control-ref of="Журнал событий"() -> (w906:refnum<vi>)
                    n692 = Concatenate Strings("После изменения порта, связь с новым портом " ("Новая строка в журнале"), w909, " установлена..." ("string")) -> (w907:string)
                    n693 = call "ProcessingJournalEvent.vi"("Новая строка в журнале"=w907, "Журнал событий"=w906, "ArchiveInput"=w905) -> ("Archive Out"=w904:refnum<class "Archive.lvclass">)  [unwired: 8 in]
                    n694 = local write "Archive Event"(w904) -> ()
                  }
                  frame Error {
                    n695 = local write "Статус связи с СПШ"(FALSE ("Статус связи с СПШ")) -> ()
                    n696 = property on="Останов" class="Bool (strict)"("DisabledEnum"=T6."Disabled and Grayed Out" ("Disabled")) -> ()  [unwired: 2 in, 2 out]
                    n697 = property on="Имя порта" class="VISAName"() -> ("Text.Text"=w919:string)  [unwired: 2 in, 2 out]
                    n698 = local read "Archive Event"() -> (w914:refnum<class "Archive.lvclass">)
                    n699 = control-ref of="Журнал событий"() -> (w915:refnum<vi>)
                    n700 = Concatenate Strings("После изменения порта, связь с новым портом " ("Новая строка в журнале"), w919, " не установилась !!!" ("string")) -> (w916:string)
                    n701 = call "ProcessingJournalEvent.vi"("error IO"=w917, "Новая строка в журнале"=w916, "Журнал событий"=w915, "ArchiveInput"=w914) -> ("Archive Out"=w913:refnum<class "Archive.lvclass">)  [unwired: 7 in]
                    n702 = local write "Archive Event"(w913) -> ()
                  }
                }
              }
              event "Выход из программы": Value Change {
                n703 = event-data() -> ("NewVal"=w922:bool)  [unwired: 1 in, 4 out]
                n704 = case shown="True" w922 {
                  frame False {
                  }
                  frame True {
                    n705 = local read "StepMotor"() -> (w940:refnum<class "StepMotor.lvclass">)
                    n706 = local read "Макс скорость двигателя"() -> (w926:dbl)
                    n707 = local read "Разрешение энкодера"() -> (w928:dbl)
                    n708 = local read "Период регистрации"() -> (w929:string)
                    n709 = local read "Скорость передачи"() -> (w925:i32)
                    n710 = call-dynamic "GetCurrentPositionPulse.vi"("StepMotor in"=w940) -> ("error out"=w936:errorcluster, "Текущая позиция"=w939:dbl, "StepMotor out"=w941:refnum<class "StepMotor.lvclass">)  [unwired: 8 in]
                    n711 = call <vilib>:"Application Directory.vi"() -> ("Application Directory"=w934:path)
                    n712 = call-dynamic "SetPosition.vi"("error in (no error)"=w936, "Позиция"=w939, "StepMotor in"=w941) -> ("error out"=w937:errorcluster, "StepMotor out"=w938:refnum<class "StepMotor.lvclass">)  [unwired: 7 in]
                    n713 = local read "Имя порта"() -> (w924:refnum<visa-resource-name>)
                    n714 = local read "Редукция"() -> (w927:dbl)
                    n715 = Build Path(base path=w934, name or relative path="Properties.xml" ("string")) -> (appended path=w931:path)
                    n716 = call-dynamic "SetSpeed.vi"("error in (no error)"=w937, "Скорость об/мин"=0.0, "StepMotor in"=w938) -> ("error out"=w942:errorcluster, "StepMotor out"=w943:refnum<class "StepMotor.lvclass">)  [unwired: 7 in]
                    n717 = local write "StepMotor"(w943) -> ()
                    n718 = case shown="No Error" w942 {
                      selector: w942 -> [_ w964]
                      frame No Error {
                        n719 = local read "Archive Event"() -> (w957:refnum<class "Archive.lvclass">)
                        n720 = control-ref of="Журнал событий"() -> (w958:refnum<vi>)
                        n721 = call "ProcessingJournalEvent.vi"("Новая строка в журнале"="При выходе из программы двигатель удачно остановлен!!!", "Журнал событий"=w958, "ArchiveInput"=w957) -> ("Archive Out"=w956:refnum<class "Archive.lvclass">)  [unwired: 8 in]
                        n722 = local write "Archive Event"(w956) -> ()
                      }
                      frame Error {
                        n723 = local read "Archive Event"() -> (w961:refnum<class "Archive.lvclass">)
                        n724 = control-ref of="Журнал событий"() -> (w963:refnum<vi>)
                        n725 = call "ProcessingJournalEvent.vi"("error IO"=w964, "Новая строка в журнале"="При выходе из программы двигателю не удалось отправить сообщение!!! Возможно отсутствие связи с двигателем...", "Журнал событий"=w963, "ArchiveInput"=w961) -> ("Archive Out"=w960:refnum<class "Archive.lvclass">)  [unwired: 7 in]
                        n726 = local write "Archive Event"(w960) -> ()
                      }
                    }
                    n727 = Bundle(cluster=T7 {"Имя порта"="", "Скорость передачи"=0, "Макс скорост двигатенля"=0.0, "Редукция"=0.0, "Разрешение энкодера"=0.0, "Период регистрации"=""} ("Properties"), "Имя порта"=w924, "Скорость передачи"=w925, "Макс скорост двигатенля"=w926, "Редукция"=w927, "Разрешение энкодера"=w928, "Период регистрации"=w929) -> (w923:T7)
                    n728 = call <vilib>:"Check if File or Folder Exists.vi"("path"=w931) -> ("error out"=w932:errorcluster, "dup path"=w933:path)  [unwired: 8 in, 1 out]
                    n729 = case shown="No Error" w932 {
                      tunnel: w933 -> [w945 w949]
                      tunnel: w923 -> [w946 w948]
                      frame No Error {
                        n730 = Flatten To XML(anything=w946) -> (xml string=w947:string)
                        n731 = call-poly <vilib>:"Write to XML File.vi"("XML Input"=w947, "XML File Path"=w945) -> ()  [unwired: 7 in, 3 out]
                      }
                      frame Error {
                        n732 = Flatten To XML(anything=w948) -> (xml string=w954:string)
                        n733 = Open/Create/Replace File(file path (use dialog)=w949, operation (0:open)=T8."create") -> (refnum out=w953:refnum<file>, error out=w952:errorcluster)  [unwired: 4 in, 1 out]
                        n734 = Close File(refnum=w953, error in=w952) -> (path=w951:path, error out=w950:errorcluster)
                        n735 = call-poly <vilib>:"Write to XML File.vi"("error in (no error)"=w950, "XML Input"=w954, "XML File Path"=w951) -> ()  [unwired: 6 in, 3 out]
                      }
                    }
                  }
                }
              }
              event "OK Button": Value Change {
                n736 = event-data() -> ("NewVal"=w965:bool)  [unwired: 1 in, 4 out]
                n737 = case shown="True" w965 {
                  frame False {
                  }
                  frame True {
                    n738 = local read "Номер банка программ"() -> (w970:u16)
                    n739 = local read "StepMotor"() -> (w972:refnum<class "StepMotor.lvclass">)
                    n740 = call-dynamic "StartProgram.vi"("Номер банка программ"=w970, "StepMotor in"=w972) -> ("error out"=w967:errorcluster, "StepMotor out"=w971:refnum<class "StepMotor.lvclass">)  [unwired: 8 in]
                    n741 = local write "StepMotor"(w971) -> ()
                    n742 = local read "Archive Event"() -> (w968:refnum<class "Archive.lvclass">)
                    n743 = control-ref of="Журнал событий"() -> (w966:refnum<vi>)
                    n744 = call "ProcessingJournalEvent.vi"("error IO"=w967, "Журнал событий"=w966, "ArchiveInput"=w968) -> ("Archive Out"=w969:refnum<class "Archive.lvclass">)  [unwired: 8 in]
                    n745 = local write "Archive Event"(w969) -> ()
                  }
                }
              }
              event "Двигатель в исходное сотояние": Value Change {
                n746 = event-data() -> ("NewVal"=w973:bool)  [unwired: 1 in, 4 out]
                n747 = case shown="False" w973 {
                  selector: w973 -> [_ w976]
                  frame False {
                  }
                  frame True {
                    n748 = local read "Останов"() -> (w975:bool)
                    n749 = Not(x=w975) -> (.not. x?=w974:bool)
                    n750 = case shown="True" w974 {
                      tunnel: w976 -> [_ w979]
                      frame False {
                        n751 = One Button Dialog(message="Двигатель экстренно остановлен, чтобы продолжить, необходимо отжать кнопку \"ОСТАНОВ\" ", button name ("OK")="Хорошо я понял!!!") -> ()  [unwired: 1 out]
                      }
                      frame True {
                        n752 = local read "Прав.Конц"() -> (w985:bool)
                        n753 = local read "Лев.Конц"() -> (w984:bool)
                        n754 = Not(x=w985) -> (.not. x?=w981:bool)
                        n755 = Not(x=w984) -> (.not. x?=w982:bool)
                        n756 = And(x=w981, y=w982) -> (x .and. y?=w980:bool)
                        n757 = And(x=w979, y=w980) -> (x .and. y?=w983:bool)
                        n758 = case shown="False" w983 {
                          frame False {
                            n759 = One Button Dialog(message="Двигатель уже в исходном состоянии!!!\nВыберите \"Ручной режим\" или режим \"Планировщика\"....", button name ("OK")="Я понял....") -> ()  [unwired: 1 out]
                          }
                          frame True {
                            w999 = u16 0 items=["Разомкнуть"=0, "Замкнуть"=2] ("Status")
                            w1000 = u16 2 items=["Разомкнуть"=0, "Замкнуть"=2] ("Status")
                            n760 = local read "Макс скорость двигателя"() -> (w988:dbl)
                            n761 = local read "StepMotor"() -> (w1001:refnum<class "StepMotor.lvclass">)
                            n762 = local read "Скорость двигателя"() -> (w990:dbl)
                            n763 = call-dynamic "MaxSpeedRotation.vi"("Speed"=w988, "StepMotor in"=w1001) -> ("error out"=w997:errorcluster, "StepMotor out"=w998:refnum<class "StepMotor.lvclass">)  [unwired: 8 in]
                            n764 = local read "Редукция"() -> (w991:dbl)
                            n765 = call-dynamic "ToCloseSpeed.vi"("error in (no error)"=w997, "Status"=w1000, "StepMotor in"=w998) -> ("error out"=w995:errorcluster, "StepMotor out"=w996:refnum<class "StepMotor.lvclass">)  [unwired: 7 in]
                            n766 = Divide(x=w990, y=w991) -> (x/y=w992:dbl)
                            n767 = call-dynamic "ToClosePosition.vi"("error in (no error)"=w995, "Status"=w999, "StepMotor in"=w996) -> ("error out"=w993:errorcluster, "StepMotor out"=w994:refnum<class "StepMotor.lvclass">)  [unwired: 7 in]
                            n768 = local write "Скорость редуктора"(w992) -> ()
                            n769 = call-dynamic "SetSpeed.vi"("error in (no error)"=w993, "Скорость об/мин"=w990, "StepMotor in"=w994) -> ("error out"=w989:errorcluster, "StepMotor out"=w1002:refnum<class "StepMotor.lvclass">)  [unwired: 7 in]
                            n770 = local write "StepMotor"(w1002) -> ()
                            n771 = case shown="No Error" w989 {
                              selector: w989 -> [_ w1065]
                              frame No Error {
                                w1043 = T6."Disabled and Grayed Out" ("Disabled")
                                n772 = local read "КонтрольКон"() -> (w1037:T4)
                                n773 = property on="КонтрольКон" class="RadioBtnsControl (strict)"() -> ("Caption.Text"=w1019:string, "Controls[]"=w1036:refnum<vi>[])  [unwired: 2 in, 2 out]
                                n774 = property on="Tab Control" class="TabCtl (strict)"() -> ("Pages"=w1042:refnum<vi>[])  [unwired: 2 in, 2 out]
                                n775 = local write "ИсхСостСтарСтоп"(TRUE ("ИсхСостСтарСтоп")) -> ()
                                n776 = Index Array(array=w1036, index=w1037) -> (element=w1033:refnum<vi>)
                                n777 = Index Array(array=w1042, index=1) -> (element=w1040:refnum<vi>)
                                n778 = property on="Скорость двигателя" class="DigNum (strict)"() -> ("Caption.Text"=w1030:string, "Value"=w1031:dbl)  [unwired: 2 in, 2 out]
                                n779 = property on="Скорость редуктора" class="DigNum (strict)"() -> ("Caption.Text"=w1023:string, "Value"=w1026:dbl)  [unwired: 2 in, 2 out]
                                n780 = To More Specific Class(target class=refnum<vi> refnum ("reference out"), reference=w1033) -> (specific class reference=w1034:refnum<vi>)  [unwired: 1 in, 1 out]
                                n781 = property on="Запустить цикл" class="Bool (strict)"("DisabledEnum"=w1043) -> ()  [unwired: 2 in, 2 out]
                                n782 = property on="Пуск Руч" class="Bool (strict)"("DisabledEnum"=w1043) -> ()  [unwired: 2 in, 2 out]
                                n783 = property class="Page"(reference=w1040, "PageVis"=FALSE ("Page Visible")) -> ()  [unwired: 1 in, 2 out]
                                n784 = property on="Property Node" class="Bool (strict)"(reference=w1034) -> ("BoolText.Text"=w1016:string)  [unwired: 1 in, 2 out]
                                n785 = local read "Archive Event"() -> (w1011:refnum<class "Archive.lvclass">)
                                n786 = Number To Fractional String(number=w1031) -> (F-format string=w1027:string)  [unwired: 3 in]
                                n787 = Number To Fractional String(number=w1026) -> (F-format string=w1022:string)  [unwired: 3 in]
                                n788 = control-ref of="Журнал событий"() -> (w1010:refnum<vi>)
                                n789 = local read "StepMotor"() -> (w1014:refnum<class "StepMotor.lvclass">)
                                n790 = call-dynamic "GetCurrentPositionPulse.vi"("StepMotor in"=w1014) -> ("error out"=w1005:errorcluster, "Текущая позиция"=w1012:dbl, "StepMotor out"=w1013:refnum<class "StepMotor.lvclass">)  [unwired: 8 in]
                                n791 = local write "StepMotor"(w1013) -> ()
                                n792 = Concatenate Strings("; " ("string"), w1030, ": " ("string"), w1027) -> (w1021:string)
                                n793 = Concatenate Strings("; " ("string"), w1023, ": " ("string"), w1022) -> (w1020:string)
                                n794 = Concatenate Strings("; " ("string"), w1019, ": " ("string"), w1016) -> (w1015:string)
                                n795 = Concatenate Strings("Пуск!!! поиска нулевого положения" ("string"), w1021, w1020, w1015) -> (w1009:string)
                                n796 = local read "Archive Event"() -> (w1006:refnum<class "Archive.lvclass">)
                                n797 = control-ref of="Журнал событий"() -> (w1004:refnum<vi>)
                                n798 = call "ProcessingJournalEvent.vi"("Новая строка в журнале"=w1009, "Журнал событий"=w1010, "ArchiveInput"=w1011) -> ("Archive Out"=w1008:refnum<class "Archive.lvclass">)  [unwired: 8 in]
                                n799 = call "ProcessingJournalEvent.vi"("error IO"=w1005, "Журнал событий"=w1004, "ArchiveInput"=w1006) -> ("Archive Out"=w1007:refnum<class "Archive.lvclass">)  [unwired: 8 in]
                                n800 = local write "Archive Event"(w1008) -> ()
                                n801 = local read "КонтрольКон"() -> (w1038:T4)
                                n802 = local write "Archive Event"(w1007) -> ()
                                n803 = case shown="\"КонтрольОбаКон\"" w1038 {
                                tunnel: w1012 -> [w1044 w1047 w1051]
                                frame "КонтрольЛевКон", Default {
                                n804 = Less Or Equal To 0?(x=w1044) -> (x <= 0?=w1045:bool)
                                n805 = case shown="True" w1045 {
                                frame False {
                                }
                                frame True {
                                n806 = property on="GaugeAngle" class="Knob (strict)"("Scale.Flipped"=TRUE) -> ()  [unwired: 2 in, 2 out]
                                }
                                }
                                }
                                frame "КонтрольПравКон" {
                                n807 = Greater Or Equal To 0?(x=w1047) -> (x >= 0?=w1048:bool)
                                n808 = case shown="True" w1048 {
                                frame False {
                                }
                                frame True {
                                n809 = property on="GaugeAngle" class="Knob (strict)"("Scale.Flipped"=FALSE) -> ()  [unwired: 2 in, 2 out]
                                }
                                }
                                }
                                frame "КонтрольОбаКон" {
                                n810 = Greater Or Equal To 0?(x=w1051) -> (x >= 0?=w1054:bool)
                                n811 = local read "Скорость двигателя"() -> (w1056:dbl)
                                n812 = local read "Скорость двигателя"() -> (w1052:dbl)
                                n813 = Less Or Equal To 0?(x=w1051) -> (x <= 0?=w1057:bool)
                                n814 = Less Or Equal To 0?(x=w1056) -> (x <= 0?=w1058:bool)
                                n815 = Greater Or Equal To 0?(x=w1052) -> (x >= 0?=w1053:bool)
                                n816 = And(x=w1058, y=w1057) -> (x .and. y?=w1050:bool)
                                n817 = And(x=w1054, y=w1053) -> (x .and. y?=w1055:bool)
                                n818 = case shown="True" w1050 {
                                frame False {
                                }
                                frame True {
                                n819 = property on="GaugeAngle" class="Knob (strict)"("Scale.Flipped"=TRUE) -> ()  [unwired: 2 in, 2 out]
                                }
                                }
                                n820 = case shown="True" w1055 {
                                frame False {
                                }
                                frame True {
                                n821 = property on="GaugeAngle" class="Knob (strict)"("Scale.Flipped"=FALSE) -> ()  [unwired: 2 in, 2 out]
                                }
                                }
                                }
                                }
                              }
                              frame Error {
                                n822 = local read "Archive Event"() -> (w1062:refnum<class "Archive.lvclass">)
                                n823 = control-ref of="Журнал событий"() -> (w1063:refnum<vi>)
                                n824 = call "ProcessingJournalEvent.vi"("error IO"=w1065, "Новая строка в журнале"="Ошибка пуска !!!\"Поиска нулевого положения\"", "Журнал событий"=w1063, "ArchiveInput"=w1062) -> ("Archive Out"=w1061:refnum<class "Archive.lvclass">)  [unwired: 7 in]
                                n825 = local write "Archive Event"(w1061) -> ()
                              }
                            }
                          }
                        }
                      }
                    }
                  }
                }
              }
              event "Запустить цикл": Value Change {
                n826 = event-data() -> ("NewVal"=w1066:bool)  [unwired: 1 in, 4 out]
                n827 = case shown="True" w1066 {
                  frame False {
                  }
                  frame True {
                    n828 = local read "Прав.Конц"() -> (w1069:bool)
                    n829 = local read "Лев.Конц"() -> (w1068:bool)
                    n830 = Or(x=w1068, y=w1069) -> (x .or. y?=w1067:bool)
                    n831 = case shown="False" w1067 {
                      selector: w1067 -> [_ w1072]
                      frame False {
                        n832 = One Button Dialog(message="Двигатель не в исходном состоянии!!!\nВыберите режим \"Поиск нулевого положения\"....", button name ("OK")="Я понял....") -> ()  [unwired: 1 out]
                      }
                      frame True {
                        w1073 = T6."Disabled and Grayed Out" ("Disabled")
                        n833 = local write "ЦиклСтартСтоп"(w1072) -> ()
                        n834 = property on="Tab Control" class="TabCtl (strict)"() -> ("Pages"=w1077:refnum<vi>[])  [unwired: 2 in, 2 out]
                        n835 = property on="Остоновить цикл" class="Bool (strict)"("DisabledEnum"=T6."Enabled" ("Disabled")) -> ()  [unwired: 2 in, 2 out]
                        n836 = Index Array(array=w1077, index=1) -> (element=w1075:refnum<vi>)
                        n837 = property class="Page"(reference=w1075, "PageVis"=FALSE ("Page Visible")) -> ()  [unwired: 1 in, 2 out]
                        n838 = property on="Запустить цикл" class="Bool (strict)"("DisabledEnum"=w1073) -> ()  [unwired: 2 in, 2 out]
                        n839 = property on="Выход из программы" class="Bool (strict)"("DisabledEnum"=w1073) -> ()  [unwired: 2 in, 2 out]
                        n840 = property on="Пуск Руч" class="Bool (strict)"("DisabledEnum"=w1073) -> ()  [unwired: 2 in, 2 out]
                        n841 = property on="Двигатель в исходное сотояние" class="Bool (strict)"("DisabledEnum"=w1073) -> ()  [unwired: 2 in, 2 out]
                      }
                    }
                  }
                }
              }
              event "Остоновить цикл": Value Change {
                n842 = event-data() -> ("NewVal"=w1079:bool)  [unwired: 1 in, 4 out]
                n843 = case shown="True" w1079 {
                  selector: w1079 -> [_ w1085]
                  frame False {
                  }
                  frame True {
                    n844 = local read "StepMotor"() -> (w1083:refnum<class "StepMotor.lvclass">)
                    n845 = Not(x=w1085) -> (.not. x?=w1084:bool)
                    n846 = local write "ЦиклСтартСтоп"(w1084) -> ()
                    n847 = call-dynamic "SetSpeed.vi"("Скорость об/мин"=0.0, "StepMotor in"=w1083) -> ("error out"=w1080:errorcluster, "StepMotor out"=w1082:refnum<class "StepMotor.lvclass">)  [unwired: 8 in]
                    n848 = local write "StepMotor"(w1082) -> ()
                    n849 = case shown="No Error" w1080 {
                      selector: w1080 -> [_ w1092]
                      frame No Error {
                        w1086 = T6."Enabled" ("Disabled")
                        n850 = property on="Tab Control" class="TabCtl (strict)"() -> ("Pages"=w1090:refnum<vi>[])  [unwired: 2 in, 2 out]
                        n851 = property on="Запустить цикл" class="Bool (strict)"("DisabledEnum"=w1086) -> ()  [unwired: 2 in, 2 out]
                        n852 = property on="Выход из программы" class="Bool (strict)"("DisabledEnum"=w1086) -> ()  [unwired: 2 in, 2 out]
                        n853 = property on="Пуск Руч" class="Bool (strict)"("DisabledEnum"=w1086) -> ()  [unwired: 2 in, 2 out]
                        n854 = property on="Двигатель в исходное сотояние" class="Bool (strict)"("DisabledEnum"=w1086) -> ()  [unwired: 2 in, 2 out]
                        n855 = Index Array(array=w1090, index=1) -> (element=w1088:refnum<vi>)
                        n856 = property class="Page"(reference=w1088, "PageVis"=TRUE ("Page Visible")) -> ()  [unwired: 1 in, 2 out]
                        n857 = property on="Остоновить цикл" class="Bool (strict)"("DisabledEnum"=T6."Disabled and Grayed Out" ("Disabled")) -> ()  [unwired: 2 in, 2 out]
                      }
                      frame Error {
                        n858 = local read "Archive Event"() -> (w1094:refnum<class "Archive.lvclass">)
                        n859 = control-ref of="Журнал событий"() -> (w1093:refnum<vi>)
                        n860 = call "ProcessingJournalEvent.vi"("error IO"=w1092, "Журнал событий"=w1093, "ArchiveInput"=w1094) -> ("Archive Out"=w1095:refnum<class "Archive.lvclass">)  [unwired: 8 in]
                        n861 = local write "Archive Event"(w1095) -> ()
                      }
                    }
                  }
                }
              }
              event "КонтрольКон": Value Change {
                w1096 = 0.0 ("Скорость об/мин")
                n862 = event-data() -> ("NewVal"=w1098:T4)  [unwired: 1 in, 4 out]
                n863 = local read "StepMotor"() -> (w1100:refnum<class "StepMotor.lvclass">)
                n864 = call-dynamic "SetSpeed.vi"("Скорость об/мин"=w1096, "StepMotor in"=w1100) -> ("error out"=w1097:errorcluster, "StepMotor out"=w1099:refnum<class "StepMotor.lvclass">)  [unwired: 8 in]
                n865 = local write "Скорость двигателя"(w1096) -> ()
                n866 = local write "Скорость редуктора"(w1096) -> ()
                n867 = local write "SpeedSlide"(w1096) -> ()
                n868 = local write "StepMotor"(w1099) -> ()
                n869 = case shown="No Error" w1097 {
                  selector: w1097 -> [_ w1141]
                  tunnel: w1098 -> [w1109 _]
                  frame No Error {
                    n870 = property on="КонтрольКон" class="RadioBtnsControl (strict)"() -> ("Caption.Text"=w1127:string, "Controls[]"=w1110:refnum<vi>[])  [unwired: 2 in, 2 out]
                    n871 = Index Array(array=w1110, index=w1109) -> (element=w1113:refnum<vi>)
                    n872 = property on="Скорость двигателя" class="DigNum (strict)"() -> ("Caption.Text"=w1116:string, "Value"=w1115:dbl)  [unwired: 2 in, 2 out]
                    n873 = property on="Скорость редуктора" class="DigNum (strict)"() -> ("Caption.Text"=w1123:string, "Value"=w1120:dbl)  [unwired: 2 in, 2 out]
                    n874 = case shown="\"КонтрольОбаКон\"" w1109 {
                      tunnel: [0.0 ("Data Entry Limits:Minimum") w1135 w1139] -> w1106
                      tunnel: [w1132 0.0 ("Data Entry Limits:Minimum") w1138] -> w1105
                      frame "КонтрольЛевКон", Default {
                        n875 = local read "Макс скорость двигателя"() -> (w1133:dbl)
                        n876 = Negate(x=w1133) -> (-x=w1132:dbl)
                      }
                      frame "КонтрольПравКон" {
                        n877 = local read "Макс скорость двигателя"() -> (w1135:dbl)
                      }
                      frame "КонтрольОбаКон" {
                        n878 = local read "Макс скорость двигателя"() -> (w1137:dbl)
                        n879 = local read "Макс скорость двигателя"() -> (w1139:dbl)
                        n880 = Negate(x=w1137) -> (-x=w1138:dbl)
                      }
                    }
                    n881 = To More Specific Class(target class=refnum<vi> refnum ("reference out"), reference=w1113) -> (specific class reference=w1112:refnum<vi>)  [unwired: 1 in, 1 out]
                    n882 = property on="Property Node" class="Bool (strict)"(reference=w1112) -> ("BoolText.Text"=w1130:string)  [unwired: 1 in, 2 out]
                    n883 = local read "Archive Event"() -> (w1102:refnum<class "Archive.lvclass">)
                    n884 = Number To Fractional String(number=w1115) -> (F-format string=w1119:string)  [unwired: 3 in]
                    n885 = Number To Fractional String(number=w1120) -> (F-format string=w1124:string)  [unwired: 3 in]
                    n886 = control-ref of="Журнал событий"() -> (w1103:refnum<vi>)
                    n887 = Concatenate Strings("; " ("string"), w1116, ": " ("string"), w1119) -> (w1125:string)
                    n888 = Concatenate Strings("; " ("string"), w1123, ": " ("string"), w1124) -> (w1126:string)
                    n889 = Concatenate Strings("; " ("string"), w1127, ": " ("string"), w1130) -> (w1131:string)
                    n890 = property on="Скорость двигателя" class="DigNum (strict)"("Maximum"=w1106, "Minimum"=w1105) -> ("Maximum"=w1108:dbl, "Minimum"=w1107:dbl)  [unwired: 2 in, 2 out]
                    n891 = Concatenate Strings("Смена направления!!! поиска нулевого положения" ("string"), w1125, w1126, w1131) -> (w1104:string)
                    n892 = call "ProcessingJournalEvent.vi"("Новая строка в журнале"=w1104, "Журнал событий"=w1103, "ArchiveInput"=w1102) -> ("Archive Out"=w1101:refnum<class "Archive.lvclass">)  [unwired: 8 in]
                    n893 = local write "Archive Event"(w1101) -> ()
                    n894 = property on="SpeedSlide" class="Slide (strict)"("Scale.Maximum"=w1108, "Scale.Minimum"=w1107) -> ()  [unwired: 2 in, 2 out]
                  }
                  frame Error {
                    n895 = local read "Archive Event"() -> (w1144:refnum<class "Archive.lvclass">)
                    n896 = control-ref of="Журнал событий"() -> (w1143:refnum<vi>)
                    n897 = call "ProcessingJournalEvent.vi"("error IO"=w1141, "Новая строка в журнале"="Ошибка смены направления!!! \"Поиска нулевого положения\"", "Журнал событий"=w1143, "ArchiveInput"=w1144) -> ("Archive Out"=w1140:refnum<class "Archive.lvclass">)  [unwired: 7 in]
                    n898 = local write "Archive Event"(w1140) -> ()
                  }
                }
              }
              event "Макс скорость двигателя": Value Change {
                n899 = event-data() -> ("NewVal"=w1145:dbl)  [unwired: 1 in, 4 out]
                n900 = local read "КонтрольКон"() -> (w1146:T4)
                n901 = case shown="\"КонтрольПравКон\"" w1146 {
                  tunnel: w1145 -> [w1147 w1152]
                  frame "КонтрольЛевКон", Default {
                    n902 = To Double Precision Float(number=w1147) -> (double precision float=w1150:dbl)
                    n903 = Multiply(x=w1150, y=-1.0) -> (x*y=w1148:dbl)
                    n904 = property on="Скорость двигателя" class="DigNum (strict)"("Maximum"=0.0 ("Data Entry Limits:Minimum"), "Minimum"=w1148) -> ()  [unwired: 2 in, 2 out]
                  }
                  frame "КонтрольПравКон" {
                    n905 = To Double Precision Float(number=w1152) -> (double precision float=w1154:dbl)
                    n906 = property on="Скорость двигателя" class="DigNum (strict)"("Maximum"=w1154, "Minimum"=0.0 ("Data Entry Limits:Minimum")) -> ()  [unwired: 2 in, 2 out]
                  }
                }
              }
              event "Скорость двигателя", "SpeedSlide": Value Change {
                n907 = event-data() -> ("CtlRef"=w1155:refnum<vi>, "NewVal"=w1158:dbl)  [unwired: 1 in, 3 out]
                n908 = property on="Скорость двигателя" class="DigNum (strict)"() -> ("Maximum"=w1162:dbl, "Minimum"=w1161:dbl)  [unwired: 2 in, 2 out]
                n909 = local read "ИсхСостСтарСтоп"() -> (w1160:bool)
                n910 = property class="Num"(reference=w1155) -> ("ClassName"=w1157:string)  [unwired: 1 in, 2 out]
                n911 = In Range and Coerce(upper limit=w1162, x=w1158, lower limit=w1161) -> (coerced(x)=w1156:dbl, In Range?=w1159:bool)
                n912 = And(x=w1159, y=w1160) -> (x .and. y?=w1163:bool)
                n913 = case shown="True" w1163 {
                  tunnel: w1156 -> [_ w1166]
                  frame False {
                  }
                  frame True {
                    n914 = local read "Редукция"() -> (w1167:dbl)
                    n915 = Divide(x=w1166, y=w1167) -> (x/y=w1168:dbl)
                    n916 = local read "StepMotor"() -> (w1171:refnum<class "StepMotor.lvclass">)
                    n917 = local write "Скорость редуктора"(w1168) -> ()
                    n918 = call-dynamic "SetSpeed.vi"("Скорость об/мин"=w1166, "StepMotor in"=w1171) -> ("error out"=w1169:errorcluster, "StepMotor out"=w1170:refnum<class "StepMotor.lvclass">)  [unwired: 8 in]
                    n919 = local write "StepMotor"(w1170) -> ()
                    n920 = case shown="No Error" w1169 {
                      selector: w1169 -> [_ w1203]
                      frame No Error {
                        n921 = local read "КонтрольКон"() -> (w1176:T4)
                        n922 = property on="КонтрольКон" class="RadioBtnsControl (strict)"() -> ("Caption.Text"=w1194:string, "Controls[]"=w1177:refnum<vi>[])  [unwired: 2 in, 2 out]
                        n923 = Index Array(array=w1177, index=w1176) -> (element=w1180:refnum<vi>)
                        n924 = property on="Скорость двигателя" class="DigNum (strict)"() -> ("Caption.Text"=w1183:string, "Value"=w1182:dbl)  [unwired: 2 in, 2 out]
                        n925 = property on="Скорость редуктора" class="DigNum (strict)"() -> ("Caption.Text"=w1190:string, "Value"=w1187:dbl)  [unwired: 2 in, 2 out]
                        n926 = To More Specific Class(target class=refnum<vi> refnum ("reference out"), reference=w1180) -> (specific class reference=w1179:refnum<vi>)  [unwired: 1 in, 1 out]
                        n927 = property on="Property Node" class="Bool (strict)"(reference=w1179) -> ("BoolText.Text"=w1197:string)  [unwired: 1 in, 2 out]
                        n928 = Number To Fractional String(number=w1182) -> (F-format string=w1186:string)  [unwired: 3 in]
                        n929 = Number To Fractional String(number=w1187) -> (F-format string=w1191:string)  [unwired: 3 in]
                        n930 = local read "Archive Event"() -> (w1174:refnum<class "Archive.lvclass">)
                        n931 = control-ref of="Журнал событий"() -> (w1173:refnum<vi>)
                        n932 = Concatenate Strings("; " ("string"), w1183, ": " ("string"), w1186) -> (w1192:string)
                        n933 = Concatenate Strings("; " ("string"), w1190, ": " ("string"), w1191) -> (w1193:string)
                        n934 = Concatenate Strings("; " ("string"), w1194, ": " ("string"), w1197) -> (w1198:string)
                        n935 = Concatenate Strings("Изменение скорости двигателя!!! поиска нулевого положения" ("string"), w1192, w1193, w1198) -> (w1175:string)
                        n936 = call "ProcessingJournalEvent.vi"("Новая строка в журнале"=w1175, "Журнал событий"=w1173, "ArchiveInput"=w1174) -> ("Archive Out"=w1172:refnum<class "Archive.lvclass">)  [unwired: 8 in]
                        n937 = local write "Archive Event"(w1172) -> ()
                      }
                      frame Error {
                        n938 = local read "Archive Event"() -> (w1200:refnum<class "Archive.lvclass">)
                        n939 = control-ref of="Журнал событий"() -> (w1201:refnum<vi>)
                        n940 = call "ProcessingJournalEvent.vi"("error IO"=w1203, "Новая строка в журнале"="Ошибка изменения скорости двигателя!!! \"Поиска нулевого положения\"", "Журнал событий"=w1201, "ArchiveInput"=w1200) -> ("Archive Out"=w1199:refnum<class "Archive.lvclass">)  [unwired: 7 in]
                        n941 = local write "Archive Event"(w1199) -> ()
                      }
                    }
                  }
                }
                n942 = case shown="\"Digital\", Default" w1157 {
                  tunnel: w1156 -> [w1164 w1165]
                  frame "Slide" {
                    n943 = local write "Скорость двигателя"(w1164) -> ()
                  }
                  frame "Digital", Default {
                    n944 = local write "SpeedSlide"(w1165) -> ()
                  }
                }
              }
              event "Расчитать скорость": Value Change {
                n945 = event-data() -> ("NewVal"=w1204:bool)  [unwired: 1 in, 4 out]
                n946 = case shown="True" w1204 {
                  frame False {
                  }
                  frame True {
                    n947 = local read "Разрешение энкодера"() -> (w1205:dbl)
                    n948 = local read "Время в мин"() -> (w1219:dbl)
                    n949 = local read "Редукция"() -> (w1206:dbl)
                    n950 = local read "Поворт экрана"() -> (w1221:dbl)
                    n951 = local read "Поворт экрана"() -> (w1211:dbl)
                    n952 = Divide(x=1.0, y=w1219) -> (x/y=w1214:dbl)
                    n953 = local read "Редукция"() -> (w1207:dbl)
                    n954 = Multiply(x=w1214, y=w1206) -> (x*y=w1218:dbl)
                    n955 = Divide(x=w1221, y=360.0 ("x")) -> (x/y=w1215:dbl)
                    n956 = Divide(x=w1211, y=360.0 ("x")) -> (x/y=w1210:dbl)
                    n957 = Multiply(x=w1205, y=w1207) -> (x*y=w1209:dbl)
                    n958 = Multiply(x=w1215, y=w1218) -> (x*y=w1217:dbl)
                    n959 = Multiply(x=w1215, y=w1214) -> (x*y=w1213:dbl)
                    n960 = local write "СкорРучРежМот"(w1217) -> ()
                    n961 = local write "СкорРучРежРед"(w1213) -> ()
                    n962 = Multiply(x=w1210, y=w1209) -> (x*y=w1208:dbl)
                    n963 = local write "Значение энкодера"(w1208) -> ()
                  }
                }
              }
              event "Пуск Руч": Value Change {
                n964 = event-data() -> ("NewVal"=w1222:bool)  [unwired: 1 in, 4 out]
                n965 = case shown="True" w1222 {
                  frame False {
                  }
                  frame True {
                    n966 = local read "Останов"() -> (w1224:bool)
                    n967 = Not(x=w1224) -> (.not. x?=w1223:bool)
                    n968 = case shown="True" w1223 {
                      frame False {
                        n969 = One Button Dialog(message="Двигатель экстренно остановлен, чтобы продолжить, необходимо отжать кнопку \"ОСТАНОВ\" ", button name ("OK")="Хорошо я понял!!!") -> ()  [unwired: 1 out]
                      }
                      frame True {
                        n970 = local read "Значение энкодера"() -> (w1229:dbl)
                        n971 = local read "СкорРучРежМот"() -> (w1234:dbl)
                        n972 = local read "СкорРучРежРед"() -> (w1232:dbl)
                        n973 = Equal To 0?(x=w1234) -> (x = 0?=w1233:bool)
                        n974 = Equal To 0?(x=w1232) -> (x = 0?=w1231:bool)
                        n975 = Equal To 0?(x=w1229) -> (x = 0?=w1230:bool)
                        n976 = Compound Arithmetic op=AND(w1233, w1231, w1230) -> (w1228:bool)
                        n977 = case shown="False" w1228 {
                          tunnel: [TRUE w1236] -> w1227
                          frame False {
                          }
                          frame True {
                            n978 = property on="Время в мин" class="DigNum (strict)"() -> ("Caption.Text"=w1250:string, "Value"=w1249:dbl)  [unwired: 2 in, 2 out]
                            n979 = property on="Поворт экрана" class="DigNum (strict)"() -> ("Caption.Text"=w1246:string, "Value"=w1245:dbl)  [unwired: 2 in, 2 out]
                            n980 = Number To Fractional String(number=w1249, precision (6)=i16 0) -> (F-format string=w1248:string)  [unwired: 2 in]
                            n981 = Number To Fractional String(number=w1245, precision (6)=i16 0) -> (F-format string=w1243:string)  [unwired: 2 in]
                            n982 = call <vilib>:"Space Constant.vi"() -> ("String"=w1244:string)
                            n983 = Concatenate Strings("Внимание!!! Вы не вычислили скорость мотора, скорость редуктора, лимит ипульсов энкодера.\nЕсли хотите расчитать с исходными данными  " ("message"), w1250, w1244, w1248, ", ", w1246, w1244, w1243, ". ") -> (w1239:string)
                            n984 = One Button Dialog(message=w1239, button name ("OK")="Хорошо я понял" ("T button name (\"OK\")")) -> (true=w1237:bool)
                            n985 = Not(x=w1237) -> (.not. x?=w1236:bool)
                          }
                        }
                        n986 = case shown="True" w1227 {
                          frame False {
                          }
                          frame True {
                            n987 = local read "Способ управления СПШ"() -> (w1252:T3)
                            n988 = case shown="\"Управления скоростью\"" w1252 {
                              frame "Управления позицией", Default {
                                w1267 = u16 2 items=["Разомкнуть"=0, "Замкнуть"=2] ("Status")
                                w1270 = u16 2 items=["Разомкнуть"=0, "Замкнуть"=2] ("Ring")
                                n989 = local read "СкорРучРежМот"() -> (w1264:dbl)
                                n990 = local read "StepMotor"() -> (w1271:refnum<class "StepMotor.lvclass">)
                                n991 = call-dynamic "MaxSpeedRotation.vi"("Speed"=w1264, "StepMotor in"=w1271) -> ("error out"=w1268:errorcluster, "StepMotor out"=w1269:refnum<class "StepMotor.lvclass">)  [unwired: 8 in]
                                n992 = call-dynamic "ToCloseSpeed.vi"("error in (no error)"=w1268, "Status"=w1270, "StepMotor in"=w1269) -> ("error out"=w1265:errorcluster, "StepMotor out"=w1266:refnum<class "StepMotor.lvclass">)  [unwired: 7 in]
                                n993 = call-dynamic "ToClosePosition.vi"("error in (no error)"=w1265, "Status"=w1267, "StepMotor in"=w1266) -> ("error out"=w1259:errorcluster, "StepMotor out"=w1260:refnum<class "StepMotor.lvclass">)  [unwired: 7 in]
                                n994 = call-dynamic "GetCurrentPositionPulse.vi"("error in (no error)"=w1259, "StepMotor in"=w1260) -> ("error out"=w1258:errorcluster, "Текущая позиция"=w1253:dbl, "StepMotor out"=w1256:refnum<class "StepMotor.lvclass">)  [unwired: 7 in]
                                n995 = local read "Напраление вращения"() -> (w1261:enum32{"Лево", "Право"})
                                n996 = local write "Начальная позиция"(w1253) -> ()
                                n997 = local write "Текущая позиция"(w1253) -> ()
                                n998 = case shown="\"Лево\", Default" w1261 {
                                tunnel: [w1282 w1304] -> w1254
                                tunnel: [w1281 w1303] -> w1257
                                tunnel: w1258 -> [w1281 w1303]
                                tunnel: [w1280 w1302] -> w1255
                                tunnel: w1256 -> [w1280 w1302]
                                tunnel: w1253 -> [w1277 w1297]
                                frame "Лево", Default {
                                n999 = Less Or Equal To 0?(x=w1277) -> (x <= 0?=w1279:bool)
                                n1000 = local read "Разрешение энкодера"() -> (w1275:dbl)
                                n1001 = case shown="True" w1279 {
                                frame False {
                                }
                                frame True {
                                n1002 = property on="GaugeAngle" class="Knob (strict)"("Scale.Flipped"=TRUE) -> ()  [unwired: 2 in, 2 out]
                                }
                                }
                                n1003 = local read "Редукция"() -> (w1274:dbl)
                                n1004 = local read "Значение энкодера"() -> (w1273:dbl)
                                n1005 = local read "Текущая позиция"() -> (w1278:dbl)
                                n1006 = Multiply(x=w1274, y=w1275) -> (x*y=w1272:dbl)
                                n1007 = Negate(x=w1272) -> (-x=w1276:dbl)
                                n1008 = Subtract(x=w1278, y=w1273) -> (x-y=w1283:dbl)
                                n1009 = Less Or Equal?(x=w1283, y=w1276) -> (x <= y?=w1284:bool)
                                n1010 = case shown="True" w1284 {
                                tunnel: w1283 -> [w1287 w1292]
                                tunnel: [w1287 w1291] -> w1282
                                frame False {
                                n1011 = local write "Выбег"(0.0 ("Выбег")) -> ()
                                }
                                frame True {
                                n1012 = local read "Разрешение энкодера"() -> (w1290:dbl)
                                n1013 = local read "Редукция"() -> (w1289:dbl)
                                n1014 = Multiply(x=w1289, y=w1290) -> (x*y=w1288:dbl)
                                n1015 = Negate(x=w1288) -> (-x=w1291:dbl)
                                n1016 = Subtract(x=w1291, y=w1292) -> (x-y=w1293:dbl)
                                n1017 = local write "Выбег"(w1293) -> ()
                                }
                                }
                                }
                                frame "Право" {
                                n1018 = Greater Or Equal To 0?(x=w1297) -> (x >= 0?=w1301:bool)
                                n1019 = local read "Разрешение энкодера"() -> (w1296:dbl)
                                n1020 = local read "Значение энкодера"() -> (w1298:dbl)
                                n1021 = local read "Текущая позиция"() -> (w1299:dbl)
                                n1022 = case shown="True" w1301 {
                                frame False {
                                }
                                frame True {
                                n1023 = property on="GaugeAngle" class="Knob (strict)"("Scale.Flipped"=FALSE) -> ()  [unwired: 2 in, 2 out]
                                }
                                }
                                n1024 = local read "Редукция"() -> (w1295:dbl)
                                n1025 = Multiply(x=w1295, y=w1296) -> (x*y=w1294:dbl)
                                n1026 = Add(x=w1299, y=w1298) -> (x+y=w1300:dbl)
                                n1027 = Greater Or Equal?(x=w1300, y=w1294) -> (x >= y?=w1305:bool)
                                n1028 = case shown="True" w1305 {
                                tunnel: [w1308 w1309] -> w1304
                                tunnel: w1300 -> [w1308 w1312]
                                frame False {
                                n1029 = local write "Выбег"(0.0 ("Выбег")) -> ()
                                }
                                frame True {
                                n1030 = local read "Разрешение энкодера"() -> (w1310:dbl)
                                n1031 = local read "Редукция"() -> (w1311:dbl)
                                n1032 = Multiply(x=w1311, y=w1310) -> (x*y=w1309:dbl)
                                n1033 = Subtract(x=w1312, y=w1309) -> (x-y=w1313:dbl)
                                n1034 = local write "Выбег"(w1313) -> ()
                                }
                                }
                                }
                                }
                                n1035 = local write "Заданная позиция"(w1254) -> ()
                                n1036 = call-dynamic "SetPosition.vi"("error in (no error)"=w1257, "Позиция"=w1254, "StepMotor in"=w1255) -> ("error out"=w1262:errorcluster, "StepMotor out"=w1263:refnum<class "StepMotor.lvclass">)  [unwired: 7 in]
                                n1037 = local write "StepMotor"(w1263) -> ()
                                n1038 = case shown="No Error" w1262 {
                                selector: w1262 -> [_ w1376]
                                frame No Error {
                                w1365 = TRUE ("Boolean")
                                w1370 = T6."Disabled and Grayed Out" ("Disabled")
                                n1039 = local read "Способ управления СПШ"() -> (w1323:T3)
                                n1040 = local read "Напраление вращения"() -> (w1347:enum32{"Лево", "Право"})
                                n1041 = local write "Инкремент импульсов"(0.0 ("Инкремент импульсо")) -> ()
                                n1042 = local write "Условие энкодер"(FALSE ("Boolean 2")) -> ()
                                n1043 = local write "РучнойСтартСтоп"(w1365) -> ()
                                n1044 = local write "Условие время"(w1365) -> ()
                                n1045 = property on="Tab Control" class="TabCtl (strict)"() -> ("Pages"=w1369:refnum<vi>[])  [unwired: 2 in, 2 out]
                                n1046 = Index Array(array=w1369, index=1) -> (element=w1367:refnum<vi>)
                                n1047 = property on="Способ управления СПШ" class="RadioBtnsControl (strict)"() -> ("Caption.Text"=w1325:string, "Controls[]"=w1322:refnum<vi>[])  [unwired: 2 in, 2 out]
                                n1048 = property on="Напраление вращения" class="RadioBtnsControl (strict)"() -> ("Caption.Text"=w1350:string, "Controls[]"=w1349:refnum<vi>[])  [unwired: 2 in, 2 out]
                                n1049 = property class="Page"(reference=w1367, "PageVis"=FALSE ("Page Visible")) -> ()  [unwired: 1 in, 2 out]
                                n1050 = Index Array(array=w1322, index=w1323) -> (element=w1324:refnum<vi>)
                                n1051 = Index Array(array=w1349, index=w1347) -> (element=w1348:refnum<vi>)
                                n1052 = property on="Выбег" class="DigNum (strict)"() -> ("Caption.Text"=w1359:string, "Value"=w1362:dbl)  [unwired: 2 in, 2 out]
                                n1053 = property on="Время в мин" class="DigNum (strict)"() -> ("Caption.Text"=w1338:string, "Value"=w1342:dbl)  [unwired: 2 in, 2 out]
                                n1054 = property on="Заданная позиция" class="DigNum (strict)"() -> ("Caption.Text"=w1354:string, "Value"=w1357:dbl)  [unwired: 2 in, 2 out]
                                n1055 = property on="Поворт экрана" class="DigNum (strict)"() -> ("Caption.Text"=w1334:string, "Value"=w1339:dbl)  [unwired: 2 in, 2 out]
                                n1056 = property on="Стоп Руч" class="Bool (strict)"("DisabledEnum"=T6."Enabled" ("Disabled")) -> ()  [unwired: 2 in, 2 out]
                                n1057 = property class="Ctl"(reference=w1324) -> ("Label.Text"=w1326:string)  [unwired: 1 in, 2 out]
                                n1058 = property class="Ctl"(reference=w1348) -> ("Label.Text"=w1344:string)  [unwired: 1 in, 2 out]
                                n1059 = Number To Fractional String(number=w1357, precision (6)=i16 0 ("width (-)")) -> (F-format string=w1353:string)  [unwired: 2 in]
                                n1060 = Number To Fractional String(number=w1362, precision (6)=i16 0 ("width (-)")) -> (F-format string=w1361:string)  [unwired: 2 in]
                                n1061 = Number To Fractional String(number=w1342, precision (6)=i16 0 ("width (-)")) -> (F-format string=w1336:string)  [unwired: 2 in]
                                n1062 = Number To Fractional String(number=w1339, precision (6)=i16 0 ("width (-)")) -> (F-format string=w1333:string)  [unwired: 2 in]
                                n1063 = property on="Выход из программы" class="Bool (strict)"("DisabledEnum"=w1370) -> ()  [unwired: 2 in, 2 out]
                                n1064 = property on="Запустить цикл" class="Bool (strict)"("DisabledEnum"=w1370) -> ()  [unwired: 2 in, 2 out]
                                n1065 = property on="Двигатель в исходное сотояние" class="Bool (strict)"("DisabledEnum"=w1370) -> ()  [unwired: 2 in, 2 out]
                                n1066 = property on="Пуск Руч" class="Bool (strict)"("DisabledEnum"=w1370) -> ()  [unwired: 2 in, 2 out]
                                n1067 = Concatenate Strings("; " ("string"), w1325, ": " ("string"), w1326) -> (w1321:string)
                                n1068 = Concatenate Strings("; " ("string"), w1354, ": " ("string"), w1353) -> (w1352:string)
                                n1069 = Concatenate Strings("; " ("string"), w1359, ": " ("string"), w1361) -> (w1351:string)
                                n1070 = Concatenate Strings("; " ("string"), w1350, ": " ("string"), w1344) -> (w1343:string)
                                n1071 = Concatenate Strings("; " ("string"), w1338, ": " ("string"), w1336) -> (w1331:string)
                                n1072 = Concatenate Strings("; " ("string"), w1334, ": " ("string"), w1333) -> (w1330:string)
                                n1073 = local read "Archive Event"() -> (w1317:refnum<class "Archive.lvclass">)
                                n1074 = Concatenate Strings("Пуск!!! \"Ручной режим управления\"" ("Новая строка в журнале"), w1321, w1352, w1351, w1343, w1331, w1330) -> (w1315:string)
                                n1075 = control-ref of="Журнал событий"() -> (w1316:refnum<vi>)
                                n1076 = call "ProcessingJournalEvent.vi"("Новая строка в журнале"=w1315, "Журнал событий"=w1316, "ArchiveInput"=w1317) -> ("Archive Out"=w1314:refnum<class "Archive.lvclass">)  [unwired: 8 in]
                                n1077 = local write "Archive Event"(w1314) -> ()
                                }
                                frame Error {
                                n1078 = local read "Archive Event"() -> (w1373:refnum<class "Archive.lvclass">)
                                n1079 = control-ref of="Журнал событий"() -> (w1374:refnum<vi>)
                                n1080 = call "ProcessingJournalEvent.vi"("error IO"=w1376, "Новая строка в журнале"="Ошибка режима \"Управление позицией\" ", "Журнал событий"=w1374, "ArchiveInput"=w1373) -> ("Archive Out"=w1372:refnum<class "Archive.lvclass">)  [unwired: 7 in]
                                n1081 = local write "Archive Event"(w1372) -> ()
                                }
                                }
                              }
                              frame "Управления скоростью" {
                                w1388 = u16 0 items=["Разомкнуть"=0, "Замкнуть"=2] ("Status")
                                w1387 = u16 2 items=["Разомкнуть"=0, "Замкнуть"=2] ("Status")
                                n1082 = local read "Макс скорость двигателя"() -> (w1377:dbl)
                                n1083 = local read "StepMotor"() -> (w1386:refnum<class "StepMotor.lvclass">)
                                n1084 = call-dynamic "MaxSpeedRotation.vi"("Speed"=w1377, "StepMotor in"=w1386) -> ("error out"=w1390:errorcluster, "StepMotor out"=w1389:refnum<class "StepMotor.lvclass">)  [unwired: 8 in]
                                n1085 = local read "Напраление вращения"() -> (w1393:enum32{"Лево", "Право"})
                                n1086 = call-dynamic "ToCloseSpeed.vi"("error in (no error)"=w1390, "Status"=w1387, "StepMotor in"=w1389) -> ("error out"=w1392:errorcluster, "StepMotor out"=w1391:refnum<class "StepMotor.lvclass">)  [unwired: 7 in]
                                n1087 = call-dynamic "ToClosePosition.vi"("error in (no error)"=w1392, "Status"=w1388, "StepMotor in"=w1391) -> ("error out"=w1384:errorcluster, "StepMotor out"=w1385:refnum<class "StepMotor.lvclass">)  [unwired: 7 in]
                                n1088 = call-dynamic "GetCurrentPositionPulse.vi"("error in (no error)"=w1384, "StepMotor in"=w1385) -> ("error out"=w1382:errorcluster, "Текущая позиция"=w1378:dbl, "StepMotor out"=w1383:refnum<class "StepMotor.lvclass">)  [unwired: 7 in]
                                n1089 = local write "Текущая позиция"(w1378) -> ()
                                n1090 = local write "Начальная позиция"(w1378) -> ()
                                n1091 = case shown="\"Право\"" w1393 {
                                tunnel: [w1458 w1463] -> w1381
                                tunnel: w1378 -> [w1455 w1461]
                                frame "Лево", Default {
                                n1092 = Less Or Equal To 0?(x=w1455) -> (x <= 0?=w1456:bool)
                                n1093 = local read "СкорРучРежМот"() -> (w1457:dbl)
                                n1094 = case shown="True" w1456 {
                                frame False {
                                }
                                frame True {
                                n1095 = property on="GaugeAngle" class="Knob (strict)"("Scale.Flipped"=TRUE) -> ()  [unwired: 2 in, 2 out]
                                }
                                }
                                n1096 = Multiply(x=w1457, y=-1.0) -> (x*y=w1458:dbl)
                                }
                                frame "Право" {
                                n1097 = Greater Or Equal To 0?(x=w1461) -> (x >= 0?=w1462:bool)
                                n1098 = local read "СкорРучРежМот"() -> (w1463:dbl)
                                n1099 = case shown="True" w1462 {
                                frame False {
                                }
                                frame True {
                                n1100 = property on="GaugeAngle" class="Knob (strict)"("Scale.Flipped"=FALSE) -> ()  [unwired: 2 in, 2 out]
                                }
                                }
                                }
                                }
                                n1101 = call-dynamic "SetSpeed.vi"("error in (no error)"=w1382, "Скорость об/мин"=w1381, "StepMotor in"=w1383) -> ("error out"=w1380:errorcluster, "StepMotor out"=w1379:refnum<class "StepMotor.lvclass">)  [unwired: 7 in]
                                n1102 = local write "StepMotor"(w1379) -> ()
                                n1103 = case shown="No Error" w1380 {
                                selector: w1380 -> [_ w1454]
                                frame No Error {
                                w1399 = TRUE ("Boolean")
                                w1398 = 0.0 ("Инкремент импульсо")
                                w1448 = T6."Disabled and Grayed Out" ("Disabled")
                                n1104 = local read "Способ управления СПШ"() -> (w1404:T3)
                                n1105 = local read "Напраление вращения"() -> (w1413:enum32{"Лево", "Право"})
                                n1106 = local write "РучнойСтартСтоп"(w1399) -> ()
                                n1107 = local write "Условие время"(w1399) -> ()
                                n1108 = local write "Условие энкодер"(FALSE ("Boolean 2")) -> ()
                                n1109 = property on="Стоп Руч" class="Bool (strict)"("DisabledEnum"=T6."Enabled" ("Disabled")) -> ()  [unwired: 2 in, 2 out]
                                n1110 = property on="Способ управления СПШ" class="RadioBtnsControl (strict)"() -> ("Caption.Text"=w1406:string, "Controls[]"=w1403:refnum<vi>[])  [unwired: 2 in, 2 out]
                                n1111 = property on="Напраление вращения" class="RadioBtnsControl (strict)"() -> ("Caption.Text"=w1416:string, "Controls[]"=w1415:refnum<vi>[])  [unwired: 2 in, 2 out]
                                n1112 = local write "Инкремент импульсов"(w1398) -> ()
                                n1113 = local write "Выбег"(w1398) -> ()
                                n1114 = local write "Заданная позиция"(w1398) -> ()
                                n1115 = Index Array(array=w1403, index=w1404) -> (element=w1405:refnum<vi>)
                                n1116 = Index Array(array=w1415, index=w1413) -> (element=w1414:refnum<vi>)
                                n1117 = property on="Tab Control" class="TabCtl (strict)"() -> ("Pages"=w1447:refnum<vi>[])  [unwired: 2 in, 2 out]
                                n1118 = property on="Время в мин" class="DigNum (strict)"() -> ("Caption.Text"=w1438:string, "Value"=w1442:dbl)  [unwired: 2 in, 2 out]
                                n1119 = property on="СкорРучРежРед" class="DigNum (strict)"() -> ("Caption.Text"=w1420:string, "Value"=w1423:dbl)  [unwired: 2 in, 2 out]
                                n1120 = property on="Поворт экрана" class="DigNum (strict)"() -> ("Caption.Text"=w1434:string, "Value"=w1439:dbl)  [unwired: 2 in, 2 out]
                                n1121 = property on="СкорРучРежМот" class="DigNum (strict)"() -> ("Caption.Text"=w1424:string, "Value"=w1428:dbl)  [unwired: 2 in, 2 out]
                                n1122 = Index Array(array=w1447, index=1) -> (element=w1445:refnum<vi>)
                                n1123 = property class="Ctl"(reference=w1405) -> ("Label.Text"=w1400:string)  [unwired: 1 in, 2 out]
                                n1124 = property class="Ctl"(reference=w1414) -> ("Label.Text"=w1410:string)  [unwired: 1 in, 2 out]
                                n1125 = Number To Fractional String(number=w1428) -> (F-format string=w1427:string)  [unwired: 3 in]
                                n1126 = Number To Fractional String(number=w1423) -> (F-format string=w1419:string)  [unwired: 3 in]
                                n1127 = Number To Fractional String(number=w1442, precision (6)=i16 0 ("width (-)")) -> (F-format string=w1436:string)  [unwired: 2 in]
                                n1128 = Number To Fractional String(number=w1439, precision (6)=i16 0 ("width (-)")) -> (F-format string=w1433:string)  [unwired: 2 in]
                                n1129 = property class="Page"(reference=w1445, "PageVis"=FALSE ("Page Visible")) -> ()  [unwired: 1 in, 2 out]
                                n1130 = Concatenate Strings("; " ("string"), w1406, ": " ("string"), w1400) -> (w1402:string)
                                n1131 = Concatenate Strings("; " ("string"), w1438, ": " ("string"), w1436) -> (w1430:string)
                                n1132 = Concatenate Strings("; " ("string"), w1434, ": " ("string"), w1433) -> (w1429:string)
                                n1133 = Concatenate Strings("; " ("string"), w1424, ": " ("string"), w1427) -> (w1418:string)
                                n1134 = Concatenate Strings("; " ("string"), w1420, ": " ("string"), w1419) -> (w1417:string)
                                n1135 = Concatenate Strings("; " ("string"), w1416, ": " ("string"), w1410) -> (w1409:string)
                                n1136 = local read "Archive Event"() -> (w1395:refnum<class "Archive.lvclass">)
                                n1137 = property on="Выход из программы" class="Bool (strict)"("DisabledEnum"=w1448) -> ()  [unwired: 2 in, 2 out]
                                n1138 = control-ref of="Журнал событий"() -> (w1396:refnum<vi>)
                                n1139 = property on="Запустить цикл" class="Bool (strict)"("DisabledEnum"=w1448) -> ()  [unwired: 2 in, 2 out]
                                n1140 = Concatenate Strings("Пуск!!!  \"Ручной режим управления\"" ("Новая строка в журнале"), w1402, w1430, w1429, w1418, w1417, w1409) -> (w1397:string)
                                n1141 = property on="Пуск Руч" class="Bool (strict)"("DisabledEnum"=w1448) -> ()  [unwired: 2 in, 2 out]
                                n1142 = property on="Двигатель в исходное сотояние" class="Bool (strict)"("DisabledEnum"=w1448) -> ()  [unwired: 2 in, 2 out]
                                n1143 = call "ProcessingJournalEvent.vi"("Новая строка в журнале"=w1397, "Журнал событий"=w1396, "ArchiveInput"=w1395) -> ("Archive Out"=w1394:refnum<class "Archive.lvclass">)  [unwired: 8 in]
                                n1144 = local write "Archive Event"(w1394) -> ()
                                }
                                frame Error {
                                n1145 = local read "Archive Event"() -> (w1451:refnum<class "Archive.lvclass">)
                                n1146 = control-ref of="Журнал событий"() -> (w1452:refnum<vi>)
                                n1147 = call "ProcessingJournalEvent.vi"("error IO"=w1454, "Новая строка в журнале"="Ошибка выполнения режима \"Управление скоростью\"", "Журнал событий"=w1452, "ArchiveInput"=w1451) -> ("Archive Out"=w1450:refnum<class "Archive.lvclass">)  [unwired: 7 in]
                                n1148 = local write "Archive Event"(w1450) -> ()
                                }
                                }
                              }
                            }
                          }
                        }
                      }
                    }
                  }
                }
              }
              event "Стоп Руч": Value Change {
                n1149 = event-data() -> ("NewVal"=w1465:bool)  [unwired: 1 in, 4 out]
                n1150 = case shown="False" w1465 {
                  selector: w1465 -> [_ w1468]
                  frame False {
                  }
                  frame True {
                    n1151 = Not(x=w1468) -> (.not. x?=w1467:bool)
                    n1152 = local read "Способ управления СПШ"() -> (w1466:T3)
                    n1153 = local write "РучнойСтартСтоп"(w1467) -> ()
                    n1154 = case shown="\"Управления скоростью\"" w1466 {
                      frame "Управления позицией", Default {
                        n1155 = local read "StepMotor"() -> (w1475:refnum<class "StepMotor.lvclass">)
                        n1156 = call-dynamic "GetCurrentPositionPulse.vi"("StepMotor in"=w1475) -> ("error out"=w1476:errorcluster, "Текущая позиция"=w1474:dbl, "StepMotor out"=w1477:refnum<class "StepMotor.lvclass">)  [unwired: 8 in]
                        n1157 = call-dynamic "SetPosition.vi"("error in (no error)"=w1476, "Позиция"=w1474, "StepMotor in"=w1477) -> ("error out"=w1471:errorcluster, "StepMotor out"=w1472:refnum<class "StepMotor.lvclass">)  [unwired: 7 in]
                        n1158 = call-dynamic "SetSpeed.vi"("error in (no error)"=w1471, "Скорость об/мин"=0.0, "StepMotor in"=w1472) -> ("error out"=w1469:errorcluster, "StepMotor out"=w1470:refnum<class "StepMotor.lvclass">)  [unwired: 7 in]
                        n1159 = local write "StepMotor"(w1470) -> ()
                        n1160 = case shown="Error" w1469 {
                          selector: w1469 -> [_ w1534]
                          frame No Error {
                            w1531 = T6."Enabled" ("Disabled")
                            n1161 = local read "Способ управления СПШ"() -> (w1485:T3)
                            n1162 = property on="Tab Control" class="TabCtl (strict)"() -> ("Pages"=w1527:refnum<vi>[])  [unwired: 2 in, 2 out]
                            n1163 = local read "Напраление вращения"() -> (w1509:enum32{"Лево", "Право"})
                            n1164 = Index Array(array=w1527, index=1) -> (element=w1529:refnum<vi>)
                            n1165 = property on="Способ управления СПШ" class="RadioBtnsControl (strict)"() -> ("Caption.Text"=w1487:string, "Controls[]"=w1484:refnum<vi>[])  [unwired: 2 in, 2 out]
                            n1166 = property on="Напраление вращения" class="RadioBtnsControl (strict)"() -> ("Caption.Text"=w1512:string, "Controls[]"=w1511:refnum<vi>[])  [unwired: 2 in, 2 out]
                            n1167 = property class="Page"(reference=w1529, "PageVis"=TRUE ("Page Visible")) -> ()  [unwired: 1 in, 2 out]
                            n1168 = property on="Стоп Руч" class="Bool (strict)"("DisabledEnum"=T6."Disabled and Grayed Out" ("Disabled")) -> ()  [unwired: 2 in, 2 out]
                            n1169 = Index Array(array=w1484, index=w1485) -> (element=w1486:refnum<vi>)
                            n1170 = Index Array(array=w1511, index=w1509) -> (element=w1510:refnum<vi>)
                            n1171 = property on="Выбег" class="DigNum (strict)"() -> ("Caption.Text"=w1521:string, "Value"=w1524:dbl)  [unwired: 2 in, 2 out]
                            n1172 = property on="Время в мин" class="DigNum (strict)"() -> ("Caption.Text"=w1500:string, "Value"=w1504:dbl)  [unwired: 2 in, 2 out]
                            n1173 = property on="Заданная позиция" class="DigNum (strict)"() -> ("Caption.Text"=w1516:string, "Value"=w1519:dbl)  [unwired: 2 in, 2 out]
                            n1174 = property on="Поворт экрана" class="DigNum (strict)"() -> ("Caption.Text"=w1496:string, "Value"=w1501:dbl)  [unwired: 2 in, 2 out]
                            n1175 = property on="Выход из программы" class="Bool (strict)"("DisabledEnum"=w1531) -> ()  [unwired: 2 in, 2 out]
                            n1176 = property class="Ctl"(reference=w1486) -> ("Label.Text"=w1488:string)  [unwired: 1 in, 2 out]
                            n1177 = property class="Ctl"(reference=w1510) -> ("Label.Text"=w1506:string)  [unwired: 1 in, 2 out]
                            n1178 = Number To Fractional String(number=w1519, precision (6)=i16 0 ("width (-)")) -> (F-format string=w1515:string)  [unwired: 2 in]
                            n1179 = Number To Fractional String(number=w1524, precision (6)=i16 0 ("width (-)")) -> (F-format string=w1523:string)  [unwired: 2 in]
                            n1180 = Number To Fractional String(number=w1504, precision (6)=i16 0 ("width (-)")) -> (F-format string=w1498:string)  [unwired: 2 in]
                            n1181 = Number To Fractional String(number=w1501, precision (6)=i16 0 ("width (-)")) -> (F-format string=w1495:string)  [unwired: 2 in]
                            n1182 = property on="Запустить цикл" class="Bool (strict)"("DisabledEnum"=w1531) -> ()  [unwired: 2 in, 2 out]
                            n1183 = property on="Пуск Руч" class="Bool (strict)"("DisabledEnum"=w1531) -> ()  [unwired: 2 in, 2 out]
                            n1184 = property on="Двигатель в исходное сотояние" class="Bool (strict)"("DisabledEnum"=w1531) -> ()  [unwired: 2 in, 2 out]
                            n1185 = Concatenate Strings("; " ("string"), w1487, ": " ("string"), w1488) -> (w1483:string)
                            n1186 = Concatenate Strings("; " ("string"), w1516, ": " ("string"), w1515) -> (w1514:string)
                            n1187 = Concatenate Strings("; " ("string"), w1521, ": " ("string"), w1523) -> (w1513:string)
                            n1188 = Concatenate Strings("; " ("string"), w1512, ": " ("string"), w1506) -> (w1505:string)
                            n1189 = Concatenate Strings("; " ("string"), w1500, ": " ("string"), w1498) -> (w1493:string)
                            n1190 = Concatenate Strings("; " ("string"), w1496, ": " ("string"), w1495) -> (w1492:string)
                            n1191 = local read "Archive Event"() -> (w1481:refnum<class "Archive.lvclass">)
                            n1192 = Concatenate Strings("Стоп!!! \"Ручной режим управления\"" ("Новая строка в журнале"), w1483, w1514, w1513, w1505, w1493, w1492) -> (w1479:string)
                            n1193 = control-ref of="Журнал событий"() -> (w1480:refnum<vi>)
                            n1194 = call "ProcessingJournalEvent.vi"("Новая строка в журнале"=w1479, "Журнал событий"=w1480, "ArchiveInput"=w1481) -> ("Archive Out"=w1478:refnum<class "Archive.lvclass">)  [unwired: 8 in]
                            n1195 = local write "Archive Event"(w1478) -> ()
                          }
                          frame Error {
                            n1196 = local read "Archive Event"() -> (w1537:refnum<class "Archive.lvclass">)
                            n1197 = control-ref of="Журнал событий"() -> (w1536:refnum<vi>)
                            n1198 = call "ProcessingJournalEvent.vi"("error IO"=w1534, "Новая строка в журнале"="Ошибка остановки ручного  режима управления \"Управление позицией\"", "Журнал событий"=w1536, "ArchiveInput"=w1537) -> ("Archive Out"=w1533:refnum<class "Archive.lvclass">)  [unwired: 7 in]
                            n1199 = local write "Archive Event"(w1533) -> ()
                          }
                        }
                      }
                      frame "Управления скоростью" {
                        n1200 = local read "StepMotor"() -> (w1540:refnum<class "StepMotor.lvclass">)
                        n1201 = call-dynamic "SetSpeed.vi"("Скорость об/мин"=0.0, "StepMotor in"=w1540) -> ("error out"=w1538:errorcluster, "StepMotor out"=w1541:refnum<class "StepMotor.lvclass">)  [unwired: 8 in]
                        n1202 = local write "StepMotor"(w1541) -> ()
                        n1203 = case shown="No Error" w1538 {
                          selector: w1538 -> [_ w1599]
                          frame No Error {
                            w1593 = T6."Enabled" ("Disabled")
                            n1204 = local read "Способ управления СПШ"() -> (w1550:T3)
                            n1205 = property on="Tab Control" class="TabCtl (strict)"() -> ("Pages"=w1589:refnum<vi>[])  [unwired: 2 in, 2 out]
                            n1206 = local read "Напраление вращения"() -> (w1559:enum32{"Лево", "Право"})
                            n1207 = Index Array(array=w1589, index=1) -> (element=w1591:refnum<vi>)
                            n1208 = property on="Способ управления СПШ" class="RadioBtnsControl (strict)"() -> ("Caption.Text"=w1552:string, "Controls[]"=w1549:refnum<vi>[])  [unwired: 2 in, 2 out]
                            n1209 = property on="Напраление вращения" class="RadioBtnsControl (strict)"() -> ("Caption.Text"=w1562:string, "Controls[]"=w1561:refnum<vi>[])  [unwired: 2 in, 2 out]
                            n1210 = property class="Page"(reference=w1591, "PageVis"=TRUE ("Page Visible")) -> ()  [unwired: 1 in, 2 out]
                            n1211 = property on="Стоп Руч" class="Bool (strict)"("DisabledEnum"=T6."Disabled and Grayed Out" ("Disabled")) -> ()  [unwired: 2 in, 2 out]
                            n1212 = Index Array(array=w1549, index=w1550) -> (element=w1551:refnum<vi>)
                            n1213 = Index Array(array=w1561, index=w1559) -> (element=w1560:refnum<vi>)
                            n1214 = property on="Время в мин" class="DigNum (strict)"() -> ("Caption.Text"=w1584:string, "Value"=w1588:dbl)  [unwired: 2 in, 2 out]
                            n1215 = property on="СкорРучРежРед" class="DigNum (strict)"() -> ("Caption.Text"=w1566:string, "Value"=w1569:dbl)  [unwired: 2 in, 2 out]
                            n1216 = property on="Поворт экрана" class="DigNum (strict)"() -> ("Caption.Text"=w1580:string, "Value"=w1585:dbl)  [unwired: 2 in, 2 out]
                            n1217 = property on="СкорРучРежМот" class="DigNum (strict)"() -> ("Caption.Text"=w1570:string, "Value"=w1574:dbl)  [unwired: 2 in, 2 out]
                            n1218 = property on="Выход из программы" class="Bool (strict)"("DisabledEnum"=w1593) -> ()  [unwired: 2 in, 2 out]
                            n1219 = property class="Ctl"(reference=w1551) -> ("Label.Text"=w1546:string)  [unwired: 1 in, 2 out]
                            n1220 = property class="Ctl"(reference=w1560) -> ("Label.Text"=w1556:string)  [unwired: 1 in, 2 out]
                            n1221 = Number To Fractional String(number=w1574) -> (F-format string=w1573:string)  [unwired: 3 in]
                            n1222 = Number To Fractional String(number=w1569) -> (F-format string=w1565:string)  [unwired: 3 in]
                            n1223 = Number To Fractional String(number=w1588, precision (6)=i16 0 ("width (-)")) -> (F-format string=w1582:string)  [unwired: 2 in]
                            n1224 = Number To Fractional String(number=w1585, precision (6)=i16 0 ("width (-)")) -> (F-format string=w1579:string)  [unwired: 2 in]
                            n1225 = property on="Запустить цикл" class="Bool (strict)"("DisabledEnum"=w1593) -> ()  [unwired: 2 in, 2 out]
                            n1226 = property on="Пуск Руч" class="Bool (strict)"("DisabledEnum"=w1593) -> ()  [unwired: 2 in, 2 out]
                            n1227 = property on="Двигатель в исходное сотояние" class="Bool (strict)"("DisabledEnum"=w1593) -> ()  [unwired: 2 in, 2 out]
                            n1228 = Concatenate Strings("; " ("string"), w1552, ": " ("string"), w1546) -> (w1548:string)
                            n1229 = Concatenate Strings("; " ("string"), w1584, ": " ("string"), w1582) -> (w1576:string)
                            n1230 = Concatenate Strings("; " ("string"), w1580, ": " ("string"), w1579) -> (w1575:string)
                            n1231 = Concatenate Strings("; " ("string"), w1570, ": " ("string"), w1573) -> (w1564:string)
                            n1232 = Concatenate Strings("; " ("string"), w1566, ": " ("string"), w1565) -> (w1563:string)
                            n1233 = Concatenate Strings("; " ("string"), w1562, ": " ("string"), w1556) -> (w1555:string)
                            n1234 = local read "Archive Event"() -> (w1543:refnum<class "Archive.lvclass">)
                            n1235 = control-ref of="Журнал событий"() -> (w1544:refnum<vi>)
                            n1236 = Concatenate Strings("Стоп!!!  \"Ручной режим управления\"" ("Новая строка в журнале"), w1548, w1576, w1575, w1564, w1563, w1555) -> (w1545:string)
                            n1237 = call "ProcessingJournalEvent.vi"("Новая строка в журнале"=w1545, "Журнал событий"=w1544, "ArchiveInput"=w1543) -> ("Archive Out"=w1542:refnum<class "Archive.lvclass">)  [unwired: 8 in]
                            n1238 = local write "Archive Event"(w1542) -> ()
                          }
                          frame Error {
                            n1239 = local read "Archive Event"() -> (w1596:refnum<class "Archive.lvclass">)
                            n1240 = control-ref of="Журнал событий"() -> (w1597:refnum<vi>)
                            n1241 = call "ProcessingJournalEvent.vi"("error IO"=w1599, "Новая строка в журнале"="Ошибка остановки ручного  режима управления \"Управление скоростью\"", "Журнал событий"=w1597, "ArchiveInput"=w1596) -> ("Archive Out"=w1595:refnum<class "Archive.lvclass">)  [unwired: 7 in]
                            n1242 = local write "Archive Event"(w1595) -> ()
                          }
                        }
                      }
                    }
                  }
                }
              }
              event "Статус контроллера СПШ": Value Change {
                n1243 = event-data() -> ("NewVal"=w1600:T1)  [unwired: 1 in, 4 out]
                n1244 = local read "StepMotor"() -> (w1603:refnum<class "StepMotor.lvclass">)
                n1245 = call-dynamic "SetStatusSPS.vi"("StatusController"=w1600, "StepMotor in"=w1603) -> ("error out"=w1601:errorcluster, "StepMotor out"=w1602:refnum<class "StepMotor.lvclass">)  [unwired: 8 in]
                n1246 = local write "StepMotor"(w1602) -> ()
                n1247 = case shown="No Error" w1601 {
                  selector: w1601 -> [_ w1618]
                  tunnel: w1600 -> [w1614 _]
                  frame No Error {
                    n1248 = property on="Статус контроллера СПШ" class="Enum (strict)"() -> ("Caption.Text"=w1611:string, "Strings []"=w1615:string[])  [unwired: 2 in, 2 out]
                    n1249 = Index Array(array=w1615, index=w1614) -> (element=w1610:string)
                    n1250 = Concatenate Strings("; " ("string"), w1611, ": " ("string"), w1610) -> (w1608:string)
                    n1251 = local read "Archive Event"() -> (w1605:refnum<class "Archive.lvclass">)
                    n1252 = control-ref of="Журнал событий"() -> (w1606:refnum<vi>)
                    n1253 = Concatenate Strings("Установка статуса СПШ !!!" ("Новая строка в журнале"), w1608) -> (w1607:string)
                    n1254 = call "ProcessingJournalEvent.vi"("Новая строка в журнале"=w1607, "Журнал событий"=w1606, "ArchiveInput"=w1605) -> ("Archive Out"=w1604:refnum<class "Archive.lvclass">)  [unwired: 8 in]
                    n1255 = local write "Archive Event"(w1604) -> ()
                  }
                  frame Error {
                    n1256 = local read "Archive Event"() -> (w1617:refnum<class "Archive.lvclass">)
                    n1257 = control-ref of="Журнал событий"() -> (w1620:refnum<vi>)
                    n1258 = call "ProcessingJournalEvent.vi"("error IO"=w1618, "Новая строка в журнале"="Ошибка при установки статуса СПШ !!!", "Журнал событий"=w1620, "ArchiveInput"=w1617) -> ("Archive Out"=w1616:refnum<class "Archive.lvclass">)  [unwired: 7 in]
                    n1259 = local write "Archive Event"(w1616) -> ()
                  }
                }
              }
              event "Способ управления СПШ": Value Change {
                n1260 = event-data() -> ("NewVal"=w1621:T3)  [unwired: 1 in, 4 out]
                n1261 = case shown="\"Управления скоростью\"" w1621 {
                  frame "Управления позицией", Default {
                    w1622 = FALSE ("Контроль времени")
                    n1262 = local write "Контроль энкодера"(w1622) -> ()
                    n1263 = local write "Контроль времени"(w1622) -> ()
                  }
                  frame "Управления скоростью" {
                    w1623 = TRUE ("Контроль времени")
                    n1264 = local write "Контроль энкодера"(w1623) -> ()
                    n1265 = local write "Контроль времени"(w1623) -> ()
                  }
                }
              }
              event "Период регистрации": Value Change {
                n1266 = event-data() -> ("CtlRef"=w1627:refnum<vi>, "NewVal"=w1624:string)  [unwired: 1 in, 3 out]
                n1267 = property class="CmbBox"(reference=w1627) -> ("Label.Text"=w1626:string)  [unwired: 1 in, 2 out]
                n1268 = local read "Archive Data"() -> (w1634:refnum<class "Archive.lvclass">)
                n1269 = Fract/Exp String To Number(string=w1624) -> (number=w1633:dbl)  [unwired: 3 in, 1 out]
                n1270 = local read "Archive Event"() -> (w1630:refnum<class "Archive.lvclass">)
                n1271 = call-dynamic "SetPerioRegistration.vi"("Период регистрации"=w1633, "Archive in"=w1634) -> ("Archive out"=w1635:refnum<class "Archive.lvclass">)  [unwired: 8 in, 1 out]
                n1272 = control-ref of="Журнал событий"() -> (w1632:refnum<vi>)
                n1273 = Concatenate Strings(w1626, " = " ("string"), w1624, " c" ("string")) -> (w1628:string)
                n1274 = local write "Archive Data"(w1635) -> ()
                n1275 = call "ProcessingJournalEvent.vi"("Новая строка в журнале"=w1628, "Журнал событий"=w1632, "ArchiveInput"=w1630) -> ("Archive Out"=w1631:refnum<class "Archive.lvclass">)  [unwired: 8 in]
                n1276 = local write "Archive Event"(w1631) -> ()
              }
              event "Останов": Value Change {
                n1277 = event-data() -> ("CtlRef"=w1636:refnum<vi>, "NewVal"=w1637:bool)  [unwired: 1 in, 3 out]
                n1278 = case shown="False" w1637 {
                  tunnel: w1636 -> [w1642 w1648]
                  frame False {
                    n1279 = property class="Bool (strict)"(reference=w1642) -> ("TipStrip"=w1641:string)  [unwired: 1 in, 2 out]
                    n1280 = local read "StepMotor"() -> (w1646:refnum<class "StepMotor.lvclass">)
                    n1281 = local read "Archive Event"() -> (w1644:refnum<class "Archive.lvclass">)
                    n1282 = call-dynamic "OnModulationPWM.vi"("StepMotor in"=w1646) -> ("StepMotor out"=w1647:refnum<class "StepMotor.lvclass">)  [unwired: 9 in, 1 out]
                    n1283 = control-ref of="Журнал событий"() -> (w1645:refnum<vi>)
                    n1284 = local write "StepMotor"(w1647) -> ()
                    n1285 = Concatenate Strings(w1641, "\r", ">>ВКЛ<<" ("string")) -> (w1638:string)
                    n1286 = call "ProcessingJournalEvent.vi"("Новая строка в журнале"=w1638, "Журнал событий"=w1645, "ArchiveInput"=w1644) -> ("Archive Out"=w1643:refnum<class "Archive.lvclass">)  [unwired: 8 in]
                    n1287 = local write "Archive Event"(w1643) -> ()
                  }
                  frame True {
                    n1288 = stacked-sequence {
                      tunnel: w1648 -> [_ w1666]
                      frame #0 {
                        n1289 = local read "ИсхСостСтарСтоп"() -> (w1650:bool)
                        n1290 = local read "РучнойСтартСтоп"() -> (w1649:bool)
                        n1291 = case shown="True" w1650 {
                          frame False {
                          }
                          frame True {
                            w1657 = T6."Enabled" ("Disabled")
                            n1292 = local write "ИсхСостСтарСтоп"(FALSE ("ИсхСостСтарСтоп")) -> ()
                            n1293 = property on="Tab Control" class="TabCtl (strict)"() -> ("Pages"=w1653:refnum<vi>[])  [unwired: 2 in, 2 out]
                            n1294 = property on="Пуск Руч" class="Bool (strict)"("DisabledEnum"=w1657) -> ()  [unwired: 2 in, 2 out]
                            n1295 = Index Array(array=w1653, index=1) -> (element=w1655:refnum<vi>)
                            n1296 = property on="Запустить цикл" class="Bool (strict)"("DisabledEnum"=w1657) -> ()  [unwired: 2 in, 2 out]
                            n1297 = property class="Page"(reference=w1655, "PageVis"=TRUE ("Page Visible")) -> ()  [unwired: 1 in, 2 out]
                          }
                        }
                        n1298 = case shown="True" w1649 {
                          frame False {
                          }
                          frame True {
                            n1299 = flat-sequence {
                              frame #0 {
                                n1300 = property on="Стоп Руч" class="Bool (strict)"("Val(Sgnl)"=TRUE ("Value (Signaling)")) -> ()  [unwired: 2 in, 2 out]
                              }
                              frame #1 {
                                n1301 = property on="Стоп Руч" class="Bool (strict)"("Val(Sgnl)"=FALSE ("Value (Signaling)")) -> ()  [unwired: 2 in, 2 out]
                              }
                            }
                          }
                        }
                      }
                      frame #1 {
                        n1302 = property class="Bool (strict)"(reference=w1666) -> ("TipStrip"=w1662:string)  [unwired: 1 in, 2 out]
                        n1303 = local read "StepMotor"() -> (w1668:refnum<class "StepMotor.lvclass">)
                        n1304 = local read "Archive Event"() -> (w1664:refnum<class "Archive.lvclass">)
                        n1305 = call-dynamic "OFFModulationPWM.vi"("StepMotor in"=w1668) -> ("StepMotor out"=w1667:refnum<class "StepMotor.lvclass">)  [unwired: 9 in, 1 out]
                        n1306 = control-ref of="Журнал событий"() -> (w1665:refnum<vi>)
                        n1307 = local write "StepMotor"(w1667) -> ()
                        n1308 = Concatenate Strings(w1662, "\r", ">>ВЫКЛ<<" ("string")) -> (w1661:string)
                        n1309 = call "ProcessingJournalEvent.vi"("Новая строка в журнале"=w1661, "Журнал событий"=w1665, "ArchiveInput"=w1664) -> ("Archive Out"=w1663:refnum<class "Archive.lvclass">)  [unwired: 8 in]
                        n1310 = local write "Archive Event"(w1663) -> ()
                      }
                    }
                  }
                }
              }
              event "Reload": Value Change {
                n1311 = event-data() -> ("CtlRef"=w1669:refnum<vi>, "NewVal"=w1670:bool)  [unwired: 1 in, 3 out]
                n1312 = case shown="True" w1670 {
                  tunnel: w1669 -> [_ w1671]
                  frame False {
                  }
                  frame True {
                    n1313 = local read "StepMotor"() -> (w1675:refnum<class "StepMotor.lvclass">)
                    n1314 = call-dynamic "GetResolutionEnc.vi"("StepMotor in"=w1675) -> ("error out"=w1673:errorcluster, "Разрешение энкодера"=w1672:dbl, "StepMotor out"=w1674:refnum<class "StepMotor.lvclass">)  [unwired: 8 in]
                    n1315 = local write "StepMotor"(w1674) -> ()
                    n1316 = case shown="Error" w1673 {
                      selector: w1673 -> [_ w1687]
                      tunnel: w1672 -> [w1683 _]
                      tunnel: w1671 -> [w1677 _]
                      frame No Error {
                        n1317 = property class="Bool (strict)"(reference=w1677) -> ("TipStrip"=w1681:string)  [unwired: 1 in, 2 out]
                        n1318 = property on="Разрешение энкодера" class="DigNum (strict)"("Value"=w1683) -> ("Value"=w1682:dbl)  [unwired: 2 in, 2 out]
                        n1319 = local read "Archive Event"() -> (w1685:refnum<class "Archive.lvclass">)
                        n1320 = Number To Fractional String(number=w1682, precision (6)=i16 0) -> (F-format string=w1679:string)  [unwired: 2 in]
                        n1321 = call <vilib>:"Space Constant.vi"() -> ("String"=w1680:string)
                        n1322 = control-ref of="Журнал событий"() -> (w1686:refnum<vi>)
                        n1323 = Concatenate Strings(w1681, w1680, w1679) -> (w1678:string)
                        n1324 = call "ProcessingJournalEvent.vi"("Новая строка в журнале"=w1678, "Журнал событий"=w1686, "ArchiveInput"=w1685) -> ("Archive Out"=w1684:refnum<class "Archive.lvclass">)  [unwired: 8 in]
                        n1325 = local write "Archive Event"(w1684) -> ()
                      }
                      frame Error {
                        n1326 = call <vilib>:"Simple Error Handler.vi"("error in (no error)"=w1687) -> ()  [unwired: 1 in, 8 out]
                        n1327 = local read "Archive Event"() -> (w1689:refnum<class "Archive.lvclass">)
                        n1328 = control-ref of="Журнал событий"() -> (w1690:refnum<vi>)
                        n1329 = call "ProcessingJournalEvent.vi"("error IO"=w1687, "Новая строка в журнале"="Неудачное соединение!!! связь с портом прервана…", "Журнал событий"=w1690, "ArchiveInput"=w1689) -> ("Archive Out"=w1688:refnum<class "Archive.lvclass">)  [unwired: 7 in]
                        n1330 = local write "Archive Event"(w1688) -> ()
                      }
                    }
                  }
                }
              }
            }
            n1331 = local read "StepMotor"() -> (w345:refnum<class "StepMotor.lvclass">)
          }
          frame #2 {
            n1332 = disable-structure shown="Enabled" {
              frame Disabled {
                n1333 = local read "Двигатель в исходное сотояние"() -> ()  [unwired: 1 out]
                n1334 = local read "Статус контроллера СПШ"() -> ()  [unwired: 1 out]
                n1335 = local read "Способ управления СПШ"() -> ()  [unwired: 1 out]
                n1336 = local read "Напраление вращения"() -> ()  [unwired: 1 out]
                n1337 = local read "Контроль концевиков"() -> ()  [unwired: 1 out]
                n1338 = local read "Расчитать скорость"() -> ()  [unwired: 1 out]
                n1339 = local read "Контроль энкодера"() -> ()  [unwired: 1 out]
                n1340 = local read "Контроль времени"() -> ()  [unwired: 1 out]
                n1341 = local read "КонтрольКон"() -> ()  [unwired: 1 out]
                n1342 = local read "Стоп Руч"() -> ()  [unwired: 1 out]
                n1343 = local read "Пуск Руч"() -> ()  [unwired: 1 out]
              }
              frame Enabled {
              }
            }
            n1344 = disable-structure shown="Enabled" {
              frame Disabled {
                n1345 = shared-variable "My Computer\\Library MotorSPS.lvlib\\MotorSPS Variable"() -> (w1722:T20)  [unwired: 1 in, 1 out]
                n1346 = Unbundle By Name(w1722) -> ("Ручной режим управления.Напраление вращения"=w1721:enum32{"Лево", "Право"}, "Ручной режим управления.Время в мин"=w1719:dbl, "Ручной режим управления.Поворт экрана"=w1716:dbl, "Ручной режим управления.Расчитать скорость"=w1714:bool, "Ручной режим управления.Способ управления СПШ"=w1712:T3, "Ручной режим управления.Контроль энкодера"=w1710:bool, "Ручной режим управления.Контроль времени"=w1709:bool, "Ручной режим управления.Контроль концевиков"=w1706:bool, "Ручной режим управления.ПускРуч.Пуск Руч"=w1704:bool, "Ручной режим управления.СтопРуч.Стоп Руч"=w1702:bool, "Поиск нулевого положения.КонтрольКон"=w1700:T4, "Поиск нулевого положения.Слайдер скорости.SpeedSlide"=w1699:dbl, "Поиск нулевого положения.Индикатор скорости.Скорость двигателя"=w1696:dbl, "Поиск нулевого положения.Двигаться в исходное состояние.ПускИсход"=w1694:bool, "Статус контроллера СПШ"=w1692:T1)
                n1347 = control-ref of="Двигатель в исходное сотояние"() -> (w1695:refnum<vi>)
                n1348 = control-ref of="КонтрольКон"() -> (w1701:refnum<vi>)
                n1349 = control-ref of="Способ управления СПШ"() -> (w1713:refnum<vi>)
                n1350 = control-ref of="Напраление вращения"() -> (w1720:refnum<vi>)
                n1351 = control-ref of="Статус контроллера СПШ"() -> (w1693:refnum<vi>)
                n1352 = control-ref of="Контроль концевиков"() -> (w1707:refnum<vi>)
                n1353 = control-ref of="Расчитать скорость"() -> (w1715:refnum<vi>)
                n1354 = control-ref of="Скорость двигателя"() -> (w1697:refnum<vi>)
                n1355 = control-ref of="Контроль энкодера"() -> (w1711:refnum<vi>)
                n1356 = control-ref of="Пуск Руч"() -> (w1705:refnum<vi>)
                n1357 = control-ref of="SpeedSlide"() -> (w1698:refnum<vi>)
                n1358 = control-ref of="Стоп Руч"() -> (w1703:refnum<vi>)
                n1359 = control-ref of="Контроль времени"() -> (w1708:refnum<vi>)
                n1360 = control-ref of="Время в мин"() -> (w1718:refnum<vi>)
                n1361 = control-ref of="Поворт экрана"() -> (w1717:refnum<vi>)
                n1362 = call "ControlEvent.vi"("NewValue"=w1694, "Ctl Refnum"=w1695) -> ()  [unwired: 10 in]
                n1363 = call "ControlEvent.vi"("NewValue"=w1706, "Ctl Refnum"=w1707) -> ()  [unwired: 10 in]
                n1364 = call "ControlEvent.vi"("NewValue"=w1704, "Ctl Refnum"=w1705) -> ()  [unwired: 10 in]
                n1365 = call "ControlEvent.vi"("NewValue"=w1702, "Ctl Refnum"=w1703) -> ()  [unwired: 10 in]
                n1366 = call "ControlEvent.vi"("NewValue"=w1700, "Ctl Refnum"=w1701) -> ()  [unwired: 10 in]
                n1367 = call "ControlEvent.vi"("NewValue"=w1699, "Ctl Refnum"=w1698) -> ()  [unwired: 10 in]
                n1368 = call "ControlEvent.vi"("NewValue"=w1696, "Ctl Refnum"=w1697) -> ()  [unwired: 10 in]
                n1369 = call "ControlEvent.vi"("NewValue"=w1721, "Ctl Refnum"=w1720) -> ()  [unwired: 10 in]
                n1370 = call "ControlEvent.vi"("NewValue"=w1719, "Ctl Refnum"=w1718) -> ()  [unwired: 10 in]
                n1371 = call "ControlEvent.vi"("NewValue"=w1716, "Ctl Refnum"=w1717) -> ()  [unwired: 10 in]
                n1372 = call "ControlEvent.vi"("NewValue"=w1714, "Ctl Refnum"=w1715) -> ()  [unwired: 10 in]
                n1373 = call "ControlEvent.vi"("NewValue"=w1712, "Ctl Refnum"=w1713) -> ()  [unwired: 10 in]
                n1374 = call "ControlEvent.vi"("NewValue"=w1709, "Ctl Refnum"=w1708) -> ()  [unwired: 10 in]
                n1375 = call "ControlEvent.vi"("NewValue"=w1692, "Ctl Refnum"=w1693) -> ()  [unwired: 10 in]
                n1376 = call "ControlEvent.vi"("NewValue"=w1710, "Ctl Refnum"=w1711) -> ()  [unwired: 10 in]
              }
              frame Enabled {
              }
            }
          }
        }
        n1377 = local read "Выход из программы"() -> (w288:bool)
        n1378 = Select(t=w284, s=w284, f=w288) -> (s? t:f=w287:bool)
        n1379 = Or(x=w287, y=w284) -> (x .or. y?=w285:bool)
      }
      n1380 = call-dynamic "CloseCommunications .vi"("StepMotor in"=w281) -> ("error out"=w280:errorcluster, "StepMotor out"=w282:refnum<class "StepMotor.lvclass">)  [unwired: 9 in]
      n1381 = local write "StepMotor"(w282) -> ()
      n1382 = call <vilib>:"Simple Error Handler.vi"("error in (no error)"=w280) -> ()  [unwired: 1 in, 8 out]
    }
  }
  n1383 = disable-structure shown="Disabled" {
    frame Disabled {
      n1384 = while {
        shift-right: [w1733] -> w1723
        shift-left: FALSE -> [w1737]
        stop <- w1737 stop-if-true
        n1385 = local read "Tab Control"() -> (w1731:T2)
        n1386 = local read "Выход из программы"() -> (w1736:bool)
        n1387 = case shown="\"Контроль\", Default" w1731 {
          tunnel: [_ w1802] -> w1732
          frame "Контроль", Default {
            n1388 = local read "ЦиклСтартСтоп"() -> (w1738:bool)
            n1389 = case shown="True" w1738 {
              frame False {
              }
              frame True {
                n1390 = local read "Количество циклов"() -> (w1739:i32)
                n1391 = for {
                  N: w1739 -> [_]
                  n1392 = local read "Шаги одного цикла"() -> (w1740:string[][])
                  n1393 = for {
                    tunnel: w1740 -> [w1744] mode=indexing
                    shift-right: [w1751] -> _
                    shift-left: 0 ("number") -> [w1748]
                    tunnel: w1740 -> [w1743]
                    i -> [w1742]
                    n1394 = Index Array(array=w1744, index=0) -> (element=w1756:string)
                    n1395 = Decimal String To Number(string=w1756) -> (number=w1752:i32)  [unwired: 2 in, 1 out]
                    n1396 = Add(x=w1752, y=w1748) -> (x+y=w1750:i32)
                    n1397 = Get Date/Time In Seconds() -> (seconds since 1Jan1904=w1755:timestamp)
                    n1398 = Seconds To Date/Time(time stamp (now)=w1755) -> (date time rec=w1754:T22)  [unwired: 1 in]
                    n1399 = Unbundle By Name(w1754) -> ("hour"=w1749:i32)
                    n1400 = Less Or Equal?(x=w1749, y=w1750) -> (x <= y?=w1747:bool)
                    n1401 = Greater?(x=w1749, y=w1748) -> (0:w1746:bool)
                    n1402 = And(x=w1747, y=w1746) -> (x .and. y?=w1745:bool)
                    n1403 = case shown="True" w1745 {
                      tunnel: [w1757 _] -> w1751
                      tunnel: w1750 -> [w1757 w1758]
                      tunnel: w1744 -> [_ w1761]
                      tunnel: w1743 -> [_ w1760]
                      tunnel: w1742 -> [_ w1759]
                      frame False {
                      }
                      frame True {
                        n1404 = while {
                          tunnel: w1761 -> [_]
                          tunnel: w1760 -> [w1768]
                          tunnel: w1759 -> [w1764]
                          tunnel: w1758 -> [w1766]
                          shift-right: [w1774] -> _
                          shift-left: TRUE -> [w1775]
                          stop <- FALSE stop-if-true
                          n1405 = Get Date/Time In Seconds() -> (seconds since 1Jan1904=w1779:timestamp)
                          n1406 = Increment(x=w1764) -> (x+1=w1763:i32)
                          n1407 = Seconds To Date/Time(time stamp (now)=w1779) -> (date time rec=w1780:T22)  [unwired: 1 in]
                          n1408 = Get Date/Time In Seconds() -> (seconds since 1Jan1904=w1772:timestamp)
                          n1409 = Index Array(array=w1768, index (row)=w1763, index (col)=1 ("index (row)")) -> (element=w1765:string)
                          n1410 = Unbundle By Name(w1780) -> ("hour"=w1778:i32)
                          n1411 = Seconds To Date/Time(time stamp (now)=w1772) -> (date time rec=w1771:T22)  [unwired: 1 in]
                          n1412 = Decimal String To Number(string=w1765) -> (number=w1773:i32)  [unwired: 2 in, 1 out]
                          n1413 = Unbundle By Name(w1771) -> ("minute"=w1769:i32)
                          n1414 = Greater Or Equal?(x=w1778, y=w1766) -> (x >= y?=w1776:bool)
                          n1415 = And(x=w1776, y=w1775) -> (x .and. y?=w1777:bool)
                          n1416 = case shown="True" w1777 {
                            tunnel: [_ FALSE] -> w1774
                            tunnel: w1773 -> [_ w1788]
                            frame False {
                            }
                            frame True {
                              n1417 = local read "Редукция"() -> (w1781:dbl)
                              n1418 = local read "Режим работы двигателя"() -> (w1790:T5)
                              n1419 = To Double Precision Float(number=w1788) -> (double precision float=w1789:dbl)
                              n1420 = Divide(x=1.0, y=w1789) -> (x/y=w1792:dbl)
                              n1421 = Multiply(x=w1792, y=w1781) -> (x*y=w1791:dbl)
                              n1422 = case shown="\"Цикл круговой 360° \", Default" w1790 {
                                tunnel: w1791 -> [w1795 w1798]
                                tunnel: [w1795 w1796] -> w1783
                                frame "Цикл круговой 360° ", Default {
                                }
                                frame "Цикл реверсирования 180°" {
                                n1423 = Divide(x=w1798, y=2.0) -> (x/y=w1796:dbl)
                                }
                              }
                              n1424 = local read "StepMotor"() -> (w1785:refnum<class "StepMotor.lvclass">)
                              n1425 = local read "error"() -> (w1787:errorcluster)
                              n1426 = call-dynamic "SetSpeed.vi"("Скорость об/мин"=w1783, "StepMotor in"=w1785) -> ("error out"=w1782:errorcluster, "StepMotor out"=w1784:refnum<class "StepMotor.lvclass">)  [unwired: 8 in]
                              n1427 = local write "StepMotor"(w1784) -> ()
                              n1428 = Merge Errors(w1782, w1787) -> (w1786:errorcluster)
                              n1429 = local write "error"(w1786) -> ()
                            }
                          }
                          n1430 = Greater?(x=w1769, y=w1769) -> ()  [unwired: 1 out]
                        }
                      }
                    }
                  }
                }
              }
            }
          }
          frame "Конфигурация" {
            n1431 = while {
              shift-right: [w1819] -> _
              shift-left: "" ("Tag") -> [w1821]
              shift-right: [w1812] -> w1804
              shift-left: FALSE -> [w1815]
              tunnel: [w1808] -> w1800
              tunnel: [w1807] -> w1801
              stop <- w1817 stop-if-true
              n1432 = control-ref of="Tree"() -> (w1822:refnum<vi>)
              n1433 = property on="Tab Control" class="TabCtl (strict)"() -> ("Value"=w1809:T2)  [unwired: 2 in, 2 out]
              n1434 = invoke class="Tree (strict)" method="Navigate Tree.Get Next"(reference=w1822, "Tag"=w1821) -> ("Navigate Tree:Get Next Item"=w1819:string)  [unwired: 2 in, 3 out]
              n1435 = case shown="\"Контроль\", Default" w1809 {
                tunnel: [TRUE ("x .or. y?") FALSE ("x .or. y?")] -> w1808
                frame "Контроль", Default {
                }
                frame "Конфигурация" {
                }
              }
              n1436 = local read "Выход из программы"() -> (w1811:bool)
              n1437 = Equal?(x=w1819, y="") -> (x = y?=w1818:bool)
              n1438 = case shown="False" w1818 {
                tunnel: w1819 -> [w1828 _]
                tunnel: [w1826 _] -> w1814
                tunnel: [w1825 _] -> w1807
                frame False {
                  n1439 = while {
                    shift-right: [w1838] -> _
                    shift-left: w1828 -> [w1841]
                    shift-right: [w1836] -> w1826
                    shift-left: FALSE -> [w1834]
                    tunnel: [w1829] -> w1825
                    i -> [w1840]
                    stop <- w1835 stop-if-true
                    n1440 = case shown="Default" w1840 {
                      tunnel: w1841 -> [w1864 w1868]
                      tunnel: [w1863 w1866] -> w1838
                      frame 0 {
                        n1441 = control-ref of="Tree"() -> (w1865:refnum<vi>)
                        n1442 = invoke class="Tree (strict)" method="Navigate Tree.Get Child"(reference=w1865, "Tag"=w1864) -> ("Navigate Tree:Get Child"=w1863:string)  [unwired: 2 in, 3 out]
                      }
                      frame Default {
                        n1443 = control-ref of="Tree"() -> (w1867:refnum<vi>)
                        n1444 = invoke class="Tree (strict)" method="Navigate Tree.Get Next"(reference=w1867, "Tag"=w1868) -> ("Navigate Tree:Get Next Item"=w1866:string)  [unwired: 2 in, 3 out]
                      }
                    }
                    n1445 = property on="Tab Control" class="TabCtl (strict)"() -> ("Value"=w1832:T2)  [unwired: 2 in, 2 out]
                    n1446 = case shown="\"Контроль\", Default" w1832 {
                      tunnel: [TRUE ("x .or. y?") FALSE ("x .or. y?")] -> w1829
                      frame "Контроль", Default {
                      }
                      frame "Конфигурация" {
                      }
                    }
                    n1447 = local read "Выход из программы"() -> (w1831:bool)
                    n1448 = Or(x=w1829, y=w1831) -> (x .or. y?=w1830:bool)
                    n1449 = Select(t=w1834, s=w1834, f=w1830) -> (s? t:f=w1833:bool)
                    n1450 = Equal?(x=w1838, y="") -> (x = y?=w1837:bool)
                    n1451 = Or(x=w1837, y=w1834) -> (x .or. y?=w1835:bool)
                    n1452 = Or(x=w1833, y=w1834) -> (x .or. y?=w1836:bool)
                    n1453 = case shown="False" w1837 {
                      tunnel: w1838 -> [w1852 _]
                      frame False {
                        n1454 = control-ref of="Tree"() -> (w1853:refnum<vi>)
                        n1455 = property class="Tree (strict)"(reference=w1853, "Active Item Tag"=w1852, "ActiveColNum"=3 ("Active Cell:Active Column Number")) -> ("Cell String"=w1858:string)  [unwired: 1 in, 2 out]
                        n1456 = property class="Tree (strict)"(reference=w1853, "Active Item Tag"=w1852, "ActiveColNum"=5 ("Active Cell:Active Column Number"), "CellBG"=u32 13816530) -> ()  [unwired: 1 in, 2 out]
                        n1457 = Hexadecimal String To Number(string=w1858) -> (number=w1857:u32)  [unwired: 2 in, 1 out]
                        n1458 = local read "StepMotor"() -> (w1850:refnum<class "StepMotor.lvclass">)
                        n1459 = To Unsigned Word Integer(number=w1857) -> (unsigned 16bit integer=w1849:u16)
                        n1460 = local read "error"() -> (w1860:errorcluster)
                        n1461 = call "GetParametrAddress.vi"("Адрес параметра"=w1849, "StepMotor in"=w1850) -> ("error out"=w1847:errorcluster, "Значение"=w1846:dbl, "StepMotor out"=w1848:refnum<class "StepMotor.lvclass">)  [unwired: 7 in]
                        n1462 = Merge Errors(w1847, w1860) -> (w1861:errorcluster)
                        n1463 = local write "StepMotor"(w1848) -> ()
                        n1464 = Number To Fractional String(number=w1846, precision (6)=i16 2) -> (F-format string=w1845:string)  [unwired: 2 in]
                        n1465 = local write "error"(w1861) -> ()
                        n1466 = control-ref of="Tree"() -> (w1855:refnum<vi>)
                        n1467 = property class="Tree (strict)"(reference=w1855, "Active Item Tag"=w1852, "ActiveColNum"=5 ("Active Cell:Active Column Number"), "Cell String"=w1845, "CellBG"=u32 16777215) -> ()  [unwired: 1 in, 2 out]
                      }
                      frame True {
                      }
                    }
                  }
                }
                frame True {
                }
              }
              n1468 = Or(x=w1818, y=w1815) -> (x .or. y?=w1817:bool)
              n1469 = Or(x=w1808, y=w1811) -> (x .or. y?=w1810:bool)
              n1470 = Select(t=w1815, s=w1815, f=w1810) -> (s? t:f=w1816:bool)
              n1471 = Or(x=w1816, y=w1815) -> (x .or. y?=w1813:bool)
              n1472 = Or(x=w1814, y=w1813) -> (x .or. y?=w1812:bool)
            }
            n1473 = Or(x=w1801, y=w1800) -> (x .or. y?=w1799:bool)
            n1474 = Select(t=FALSE, s=w1799, f=w1804) -> (s? t:f=w1802:bool)
          }
        }
        n1475 = Select(t=w1737, s=w1737, f=w1736) -> (s? t:f=w1735:bool)
        n1476 = Or(x=w1735, y=w1737) -> (x .or. y?=w1734:bool)
        n1477 = Or(x=w1732, y=w1734) -> (x .or. y?=w1733:bool)
      }
      n1478 = disable-structure shown="Disabled" {
        disable-tunnel: w1723 -> [w1726 _]
        frame Disabled {
          n1479 = Not(x=w1726) -> (.not. x?=w1725:bool)
          n1480 = local write "Выход из программы"(w1725) -> ()
        }
        frame Enabled {
        }
      }
      n1481 = disable-structure shown="Disabled" {
        frame Disabled {
          n1482 = Bundle By Name(cluster=T21 {"Row"=0, "Column"=0} ("Active Cell:Active Cell"), "Column"=0) -> (w1728:T21)  [unwired: 1 in]
          n1483 = property on="Шаги одного цикла" class="Tbl (strict)"("Active Cell"=w1728, "Cell BG Color"=u32 16777215) -> ()  [unwired: 2 in, 2 out]
          n1484 = Negate() -> ()  [unwired: 1 in, 1 out]
        }
        frame Enabled {
        }
      }
    }
    frame Enabled {
    }
  }
  n1485 = property on="Tab Control" class="TabCtl (strict)"() -> ("Pages"=w7:refnum<vi>[])  [unwired: 2 in, 2 out]
  n1486 = property on="Запустить цикл" class="Bool (strict)"("DisabledEnum"=w3) -> ()  [unwired: 2 in, 2 out]
  n1487 = property on="Пуск Руч" class="Bool (strict)"("DisabledEnum"=w3) -> ()  [unwired: 2 in, 2 out]
  n1488 = Index Array(array=w7, index=1) -> (element=w5:refnum<vi>)
  n1489 = property class="Page"(reference=w5, "PageVis"=TRUE ("Page Visible")) -> ()  [unwired: 1 in, 2 out]
  "error" <- errorcluster {"status"=FALSE, "code"=0, "source"=""} ("error in (no error)")
